vi "Autonomous Independent.vi"() -> ()   [LabVIEW 2020]
doc: "This VI is called when autonomous begins, and will automatically be terminated when autonomous ends. You can carry out timed or sensor driven robot movement independently without needing to return to the caller."
uses:
  <vilib>/Rock Robotics/WPI/ThirdParty/Phoenix-LabVIEW/Motor Controller/Controls/CTRE_Phoenix_MotorControl_ControlMode.ctl
  <vilib>/Rock Robotics/WPI/Solenoid/WPI_SolenoidValue.ctl
  <vilib>/Rock Robotics/WPI/Utilities/WPI_GetSetVariantRefNum.vi
  <vilib>/Rock Robotics/Network Tables/NT Read String.vi
  <vilib>/Rock Robotics/Network Tables/NT Write Numeric Array.vi
  AutonBoolean.vi
  <vilib>/Rock Robotics/Network Tables/NT Read Number.vi
  <vilib>/Rock Robotics/WPI/Solenoid/WPI_SolenoidSetEnum.vi
panel:
  out "Ty 60":dbl
  out "Ty 59":dbl
  out "Orange Limit Pressed 26":bool
  out "Blue Limit Pressed 26":bool
  out "Ty 58":dbl
  out "Orange Limit Pressed 25":bool
  out "Blue Limit Pressed 25":bool
  out "Ty 57":dbl
  out "Intake 13":bool
  out "Elevate 13":bool
  out "Ty 56":dbl
  out "Ty 55":dbl
  out "Orange Limit Pressed 24":bool
  out "Blue Limit Pressed 24":bool
  out "Ty 54":dbl
  out "Orange Limit Pressed 23":bool
  out "Blue Limit Pressed 23":bool
  out "Ty 53":dbl
  out "Intake 12":bool
  out "Elevate 12":bool
  out "Intake 11":bool
  out "Elevate 11":bool
  out "Orange Limit Pressed 22":bool
  out "Blue Limit Pressed 22":bool
  out "Ty 52":dbl
  out "Orange Limit Pressed 21":bool
  out "Blue Limit Pressed 21":bool
  out "Ty 51":dbl
  out "Ty 50":dbl
  out "Ty 49":dbl
  out "Ty 48":dbl
  out "Ty 47":dbl
  out "Ty 46":dbl
  out "Ty 45":dbl
  out "Intake 10":bool
  out "Elevate 10":bool
  out "Orange Limit Pressed 20":bool
  out "Blue Limit Pressed 20":bool
  out "Ty 44":dbl
  out "Orange Limit Pressed 19":bool
  out "Blue Limit Pressed 19":bool
  out "Ty 43":dbl
  out "Ty 42":dbl
  out "Ty 41":dbl
  out "Ty 40":dbl
  out "Ty 39":dbl
  out "Ty 38":dbl
  out "Ty 37":dbl
  out "Intake 9":bool
  out "Elevate 9":bool
  out "Orange Limit Pressed 18":bool
  out "Blue Limit Pressed 18":bool
  out "Ty 36":dbl
  out "Orange Limit Pressed 17":bool
  out "Blue Limit Pressed 17":bool
  out "Ty 35":dbl
  out "Ty 34":dbl
  out "Ty 33":dbl
  out "Intake 8":bool
  out "Elevate 8":bool
  out "Orange Limit Pressed 16":bool
  out "Blue Limit Pressed 16":bool
  out "Ty 28":dbl
  out "Orange Limit Pressed 15":bool
  out "Blue Limit Pressed 15":bool
  out "Ty 27":dbl
  out "Intake 6":bool
  out "Elevate 6":bool
  out "Orange Limit Pressed 12":bool
  out "Blue Limit Pressed 12":bool
  out "Ty 26":dbl
  out "Orange Limit Pressed 11":bool
  out "Blue Limit Pressed 11":bool
  out "Ty 25":dbl
  out "Intake 7":bool
  out "Elevate 7":bool
  out "Orange Limit Pressed 13":bool
  out "Blue Limit Pressed 13":bool
  out "Ty 29":dbl
  out "Orange Limit Pressed 14":bool
  out "Blue Limit Pressed 14":bool
  out "Ty 30":dbl
  out "Ty 31":dbl
  out "Ty 32":dbl
  out "Ty 24":dbl
  out "Ty 23":dbl
  out "Ty 22":dbl
  out "Ty 21":dbl
  out "Ty 20":dbl
  out "Ty 19":dbl
  out "Ty 18":dbl
  out "Ty 17":dbl
  out "Orange Limit Pressed 10":bool
  out "Blue Limit Pressed 10":bool
  out "Ty 16":dbl
  out "Orange Limit Pressed 9":bool
  out "Blue Limit Pressed 9":bool
  out "Ty 15":dbl
  out "Intake 5":bool
  out "Elevate 5":bool
  out "Ty 14":dbl
  out "Ty 13":dbl
  out "Ty 12":dbl
  out "Ty 11":dbl
  out "Ty 10":dbl
  out "Ty 9":dbl
  out "Orange Limit Pressed 4":bool
  out "Blue Limit Pressed 4":bool
  out "Ty 4":dbl
  out "Orange Limit Pressed 3":bool
  out "Blue Limit Pressed 3":bool
  out "Ty 3":dbl
  out "Intake 2":bool
  out "Elevate 2":bool
  out "Intake":bool
  out "Elevate":bool
  out "Orange Limit Pressed":bool
  out "Blue Limit Pressed":bool
  out "Ty":dbl
  out "Orange Limit Pressed 2":bool
  out "Blue Limit Pressed 2":bool
  out "Ty 2":dbl
  out "Intake 3":bool
  out "Elevate 3":bool
  out "Orange Limit Pressed 5":bool
  out "Blue Limit Pressed 5":bool
  out "Ty 5":dbl
  out "Orange Limit Pressed 6":bool
  out "Blue Limit Pressed 6":bool
  out "Ty 6":dbl
  out "Intake 4":bool
  out "Elevate 4":bool
  out "Orange Limit Pressed 7":bool
  out "Blue Limit Pressed 7":bool
  out "Ty 7":dbl
  out "Orange Limit Pressed 8":bool
  out "Blue Limit Pressed 8":bool
  out "Ty 8":dbl
  # "Be sure to right-click and choose Data Operations>>Make Current Value default if you want to save the array values with the VI"
types:
  T1 = typedef "WPI_JoystickDevRef.ctl" = cluster{"Device":T2}
  T2 = typedef "WPI_JoystickDeviceEnum.ctl" = enum16{"USB 0", "USB 1", "USB 2", "USB 3", "USB 4", "USB 5"}
  T3 = typedef "WPI_SolenoidValue.ctl" = enum16{"Off", "On", "Forward", "Reverse"}
  T4 = typedef "WPI_SwitchDevRef.ctl" = cluster{"DevStatus":errorcluster, "DIO Channel":T5, "CntIndex":T6, "Normally Closed":bool}
  T5 = typedef "FPGA_DIOChannel.ctl" = enum8{"DIO 0", "DIO 1", "DIO 2", "DIO 3", "DIO 4", "DIO 5", "DIO 6", "DIO 7", "DIO 8", "DIO 9", "DIO MXP 0", "DIO MXP 1", "DIO MXP 2", "DIO MXP 3", "DIO MXP 4", "DIO MXP 5", "DIO MXP 6", "DIO MXP 7", "DIO MXP 8", "DIO MXP 9", "DIO MXP 10", "DIO MXP 11", "DIO MXP 12", "DIO MXP 13", "DIO MXP 14", "DIO MXP 15", "SPI Port CS1", "SPI Port CS2", "SPI Port CS3", "SPI Port MISO", "SPI Port MOSI", "Invalid"}
  T6 = typedef "FPGA_CounterCtrSystemIndex.ctl" = enum8{"Ctr 0", "Ctr 1", "Ctr 2", "Ctr 3", "Ctr 4", "Ctr 5", "Ctr 6", "Ctr 7", "Invalid"}
  T7 = typedef "WPI_MotorControlDeviceRef.ctl" = cluster{"DeviceStatus":errorcluster, "Type":T8, "PWM":cluster{"PWM Channel":T9, "DeadBand":T10}, "CAN":cluster{"Device Number":u8, "SetOutput VI Ref":variant, "GetOutput VI Ref":variant, "Enable VI Ref":variant, "Disable VI Ref":variant, "Data":variant}, "Invert":bool, "DIO PWM":cluster{"PWM \"Enable\" Channel":T9, "DIOChannel":T5, "PWM Rate":dbl}}
  T8 = typedef "WPI_MotorControlType.ctl" = enum16{"PWM", "CAN", "DIO PWM"}
  T9 = typedef "FPGA_DIOPWMChannel.ctl" = enum8{"PWM 0", "PWM 1", "PWM 2", "PWM 3", "PWM 4", "PWM 5", "PWM 6", "PWM 7", "PWM 8", "PWM 9", "PWM MXP 0", "PWM MXP 1", "PWM MXP 2", "PWM MXP 3", "PWM MXP 4", "PWM MXP 5", "PWM MXP 6", "PWM MXP 7", "PWM MXP 8", "PWM MXP 9", "Invalid"}
  T10 = typedef "WPI_PWMDeadband.ctl" = cluster{"Name":string, "maxPositivePwm":i32, "minPositivePwm":i32, "centerPwm":i32, "maxNegativePwm":i32, "minNegativePwm":i32, "angularRange":u16}
  T11 = typedef "CTRE_Phoenix_MotorControl_ControlMode.ctl" = u16
  T12 = typedef "WPI_SolenoidDevRef.ctl" = cluster{"DevStatus":errorcluster, "Pneumatics Control Module":u8, "Forward Solenoid Channel":T13, "Reverse Solenoid Channel":T13}
  T13 = typedef "WPI_SolenoidChannel.ctl" = enum8{"Solenoid 0", "Solenoid 1", "Solenoid 2", "Solenoid 3", "Solenoid 4", "Solenoid 5", "Solenoid 6", "Solenoid 7", "Solenoid 8", "Solenoid 9", "Solenoid 10", "Solenoid 11", "Solenoid 12", "Solenoid 13", "Solenoid 14", "Solenoid 15", "Invalid"}
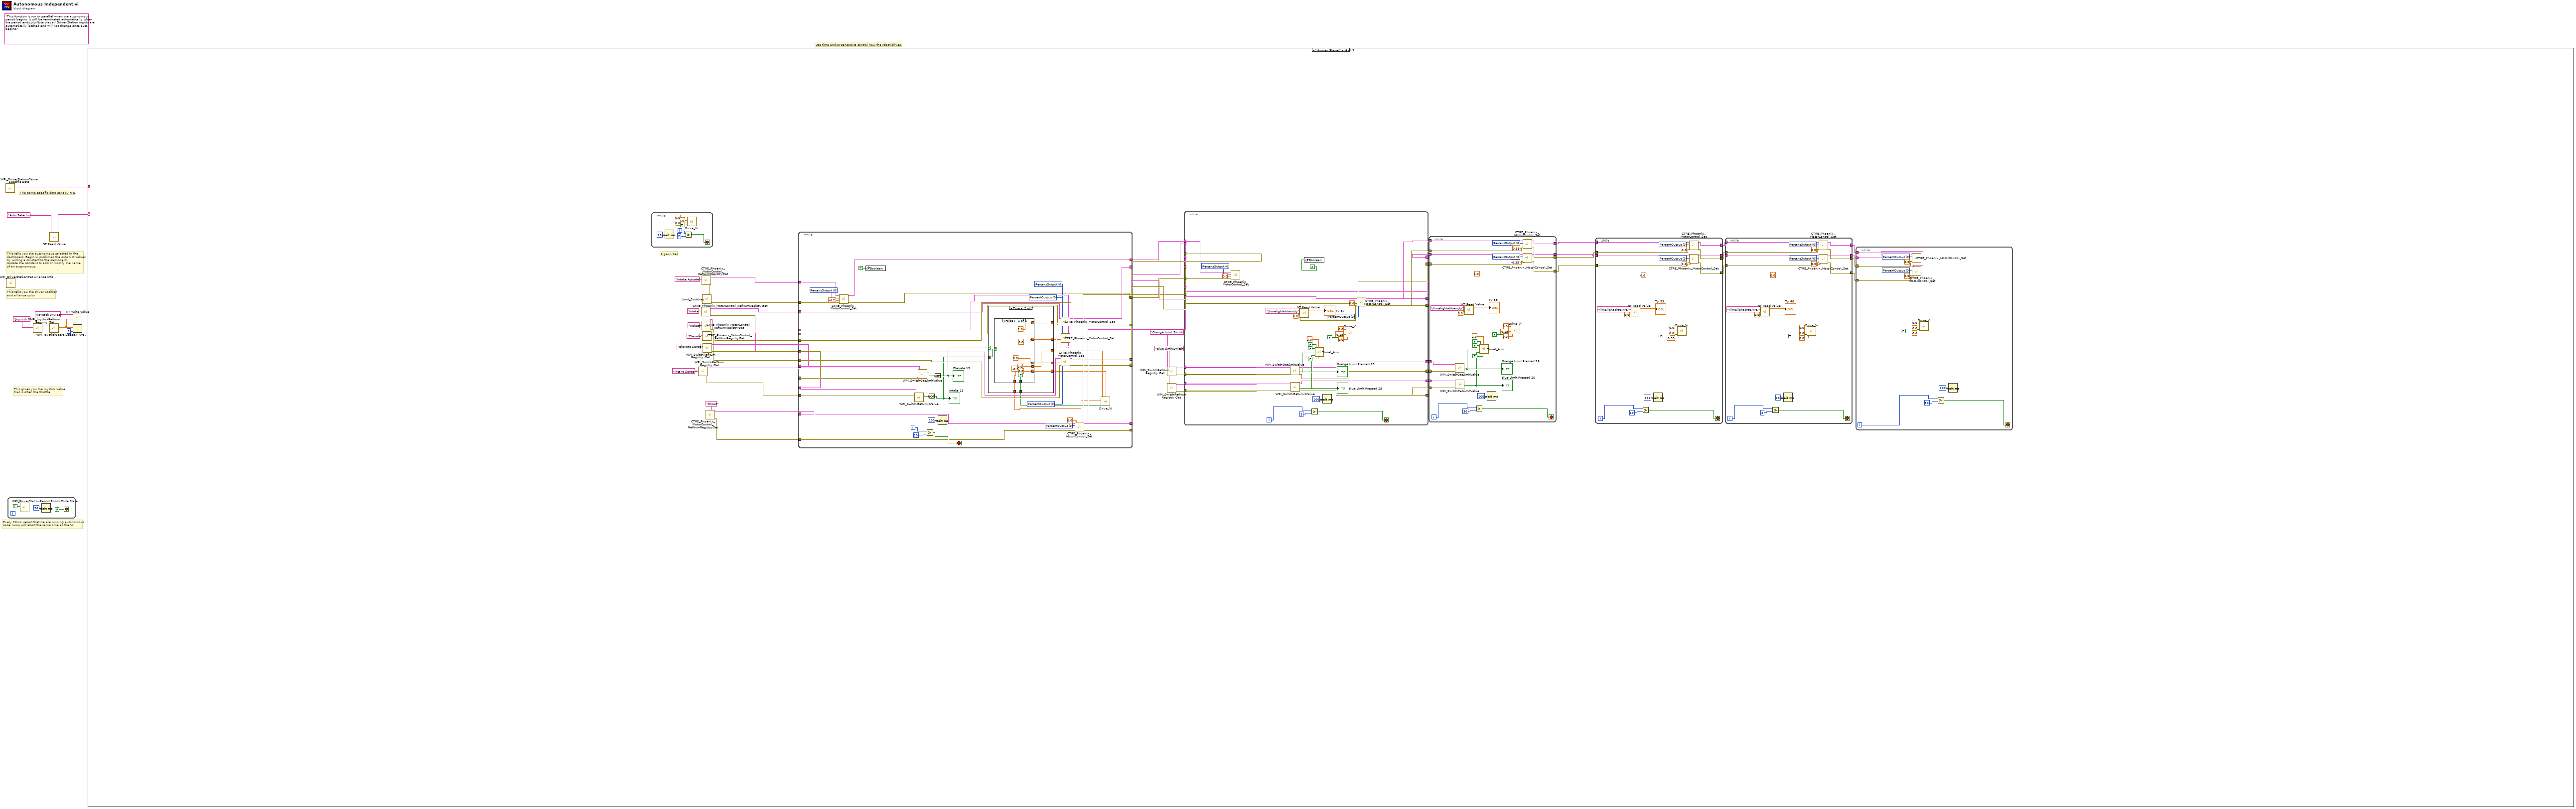
[diagram p0: block diagram]
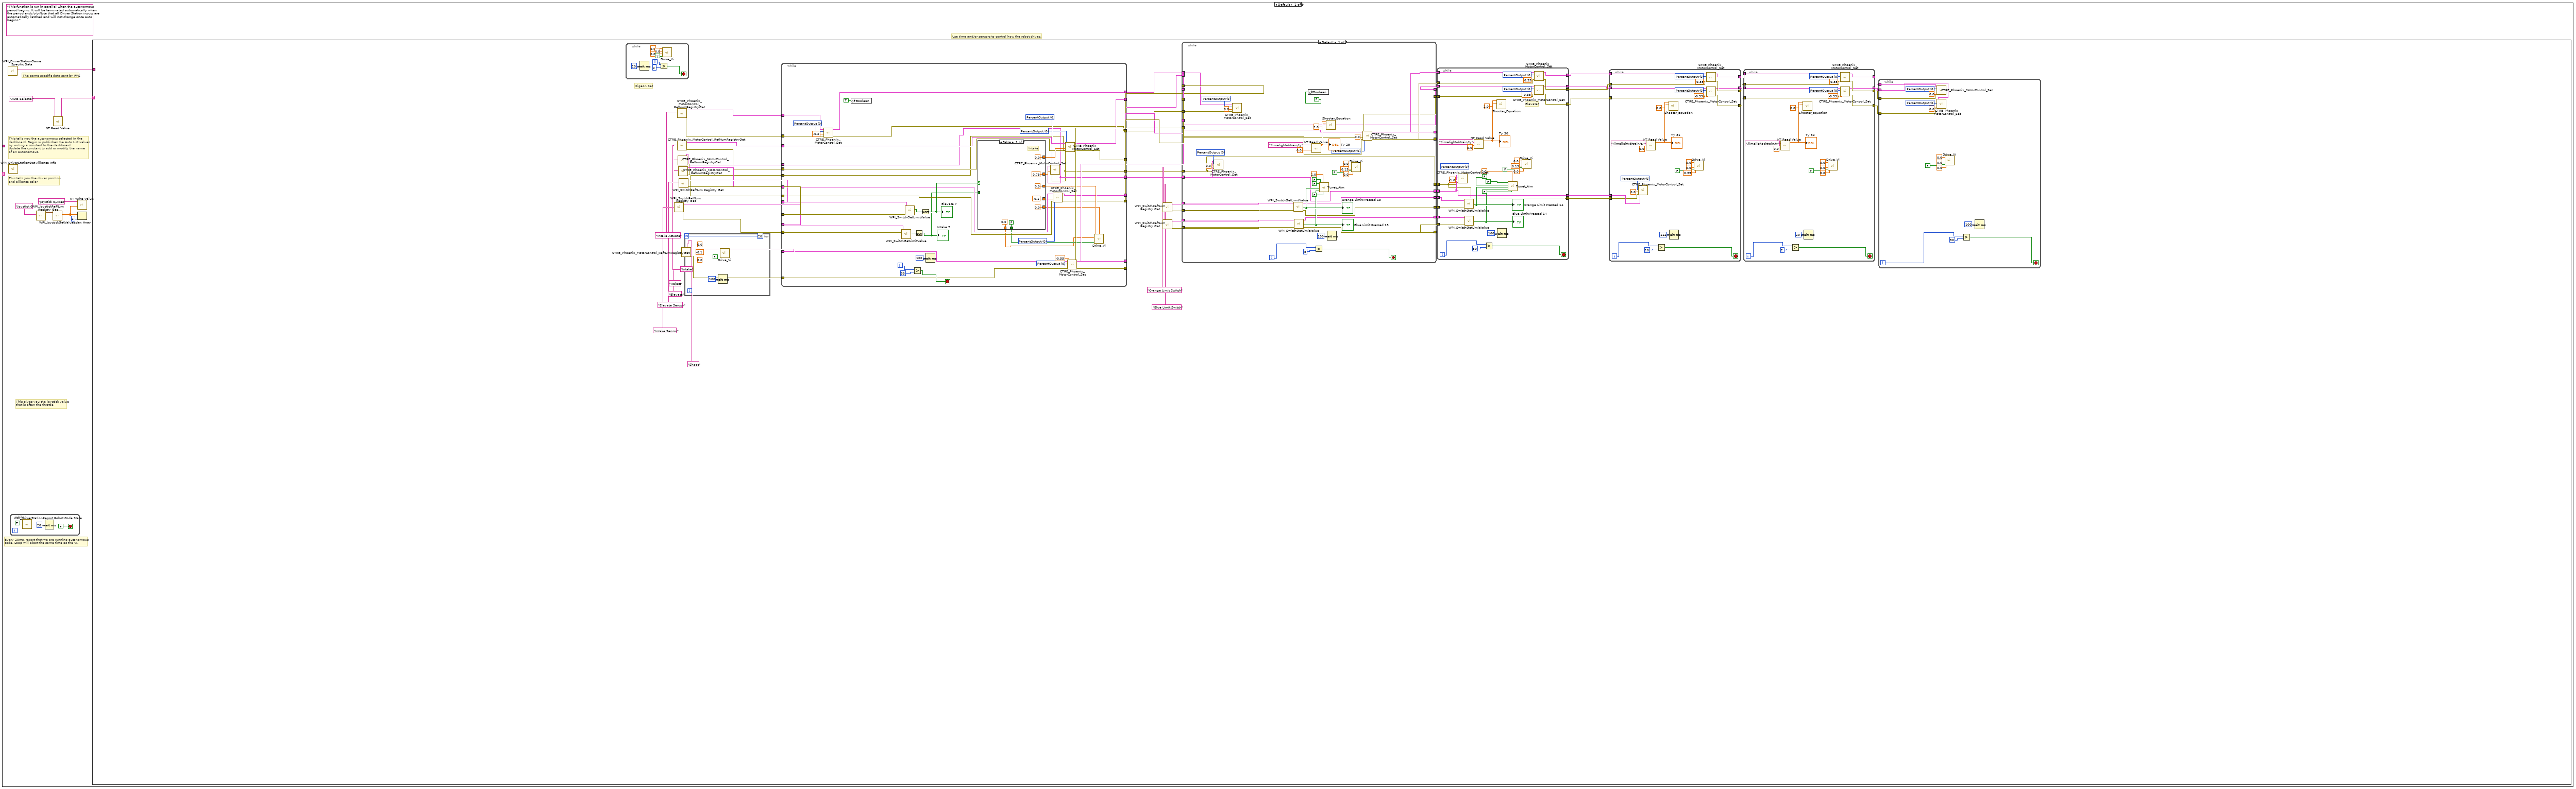
[diagram p2: hidden frame]
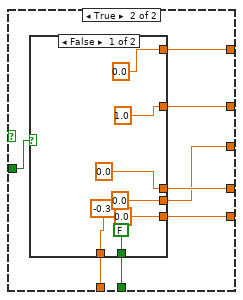
[diagram p3: hidden frame]
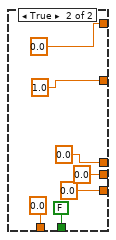
[diagram p4: hidden frame]
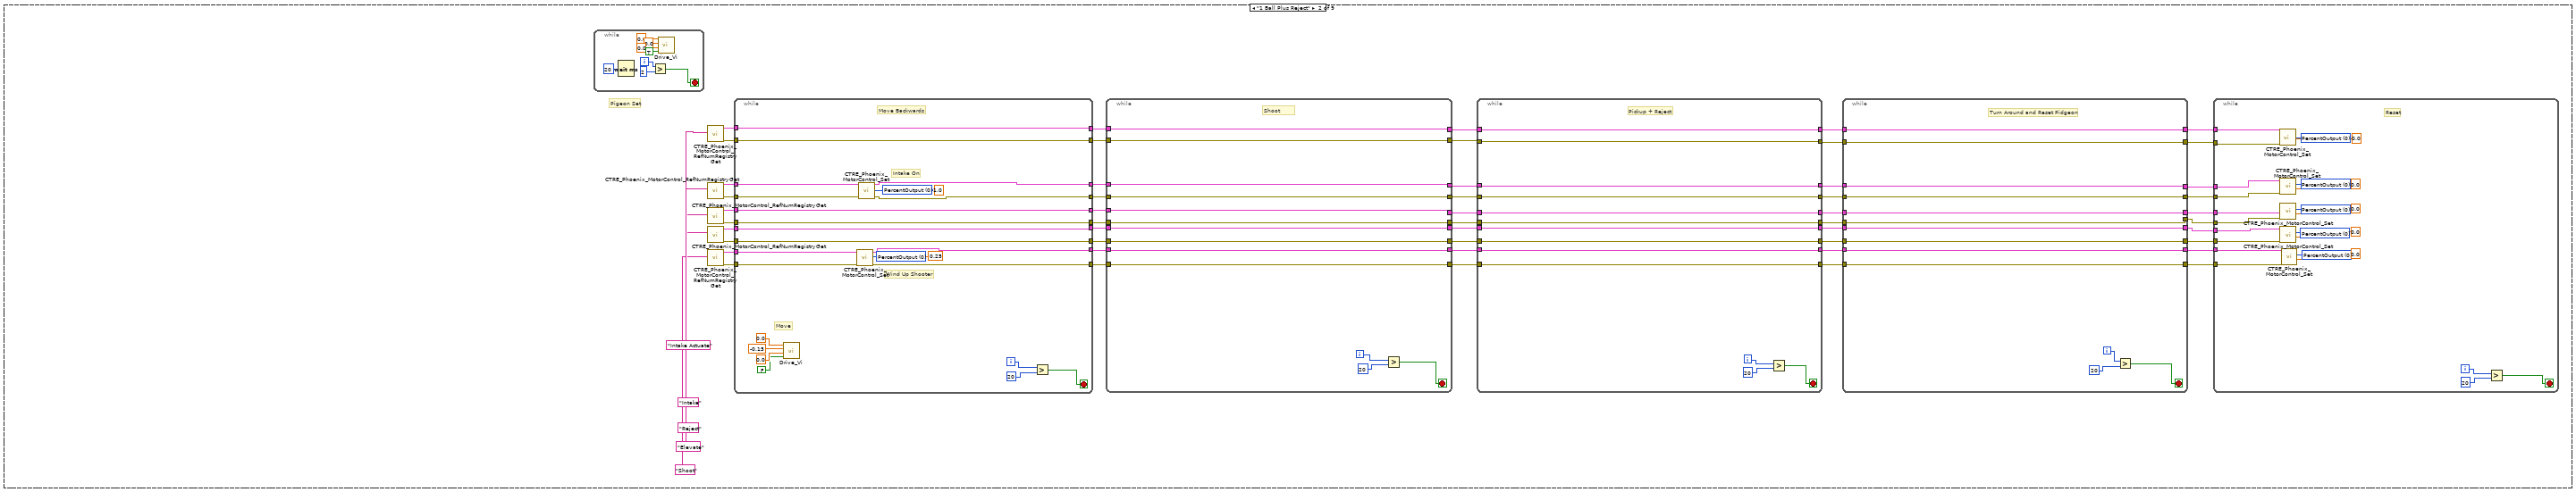
[diagram p5: hidden frame]
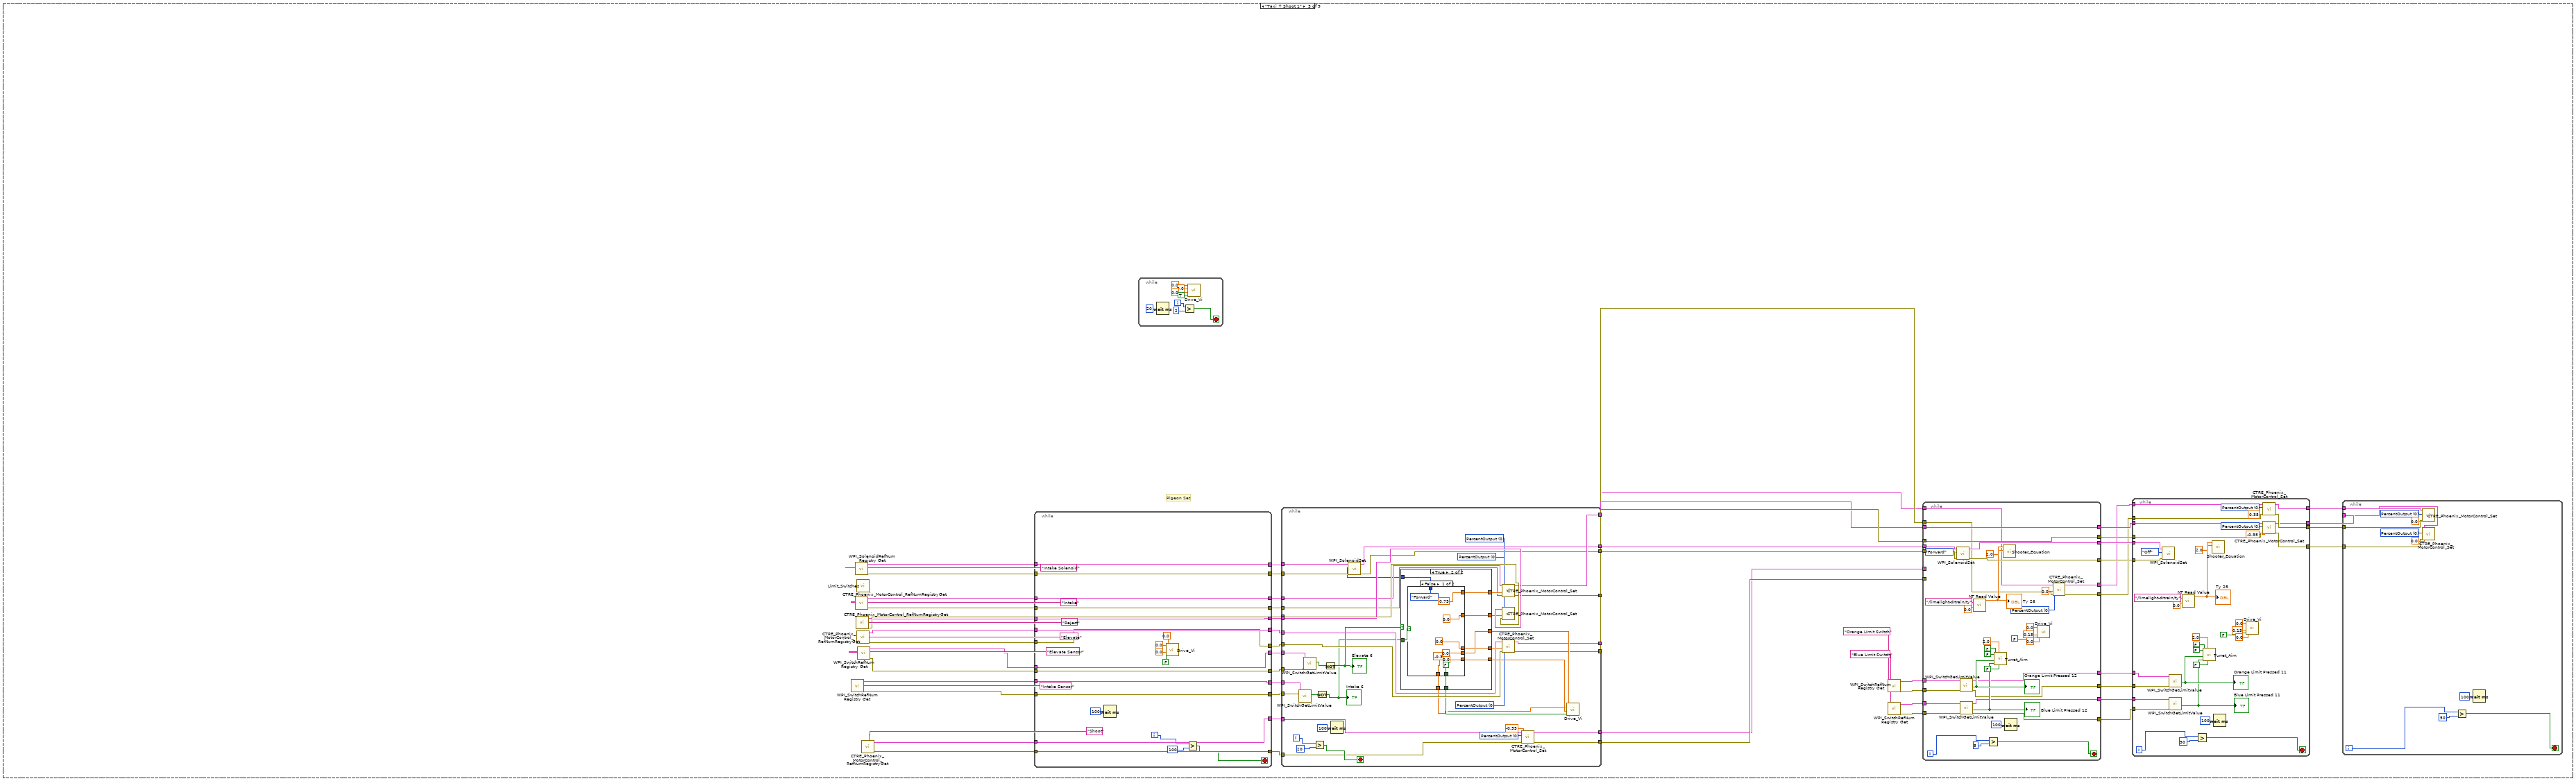
[diagram p6: hidden frame]
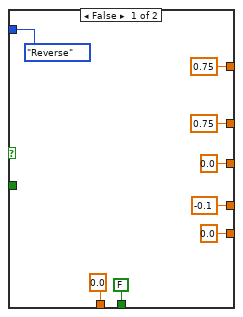
[diagram p7: hidden frame]
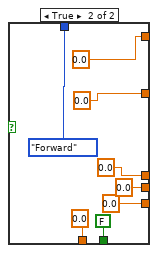
[diagram p8: hidden frame]
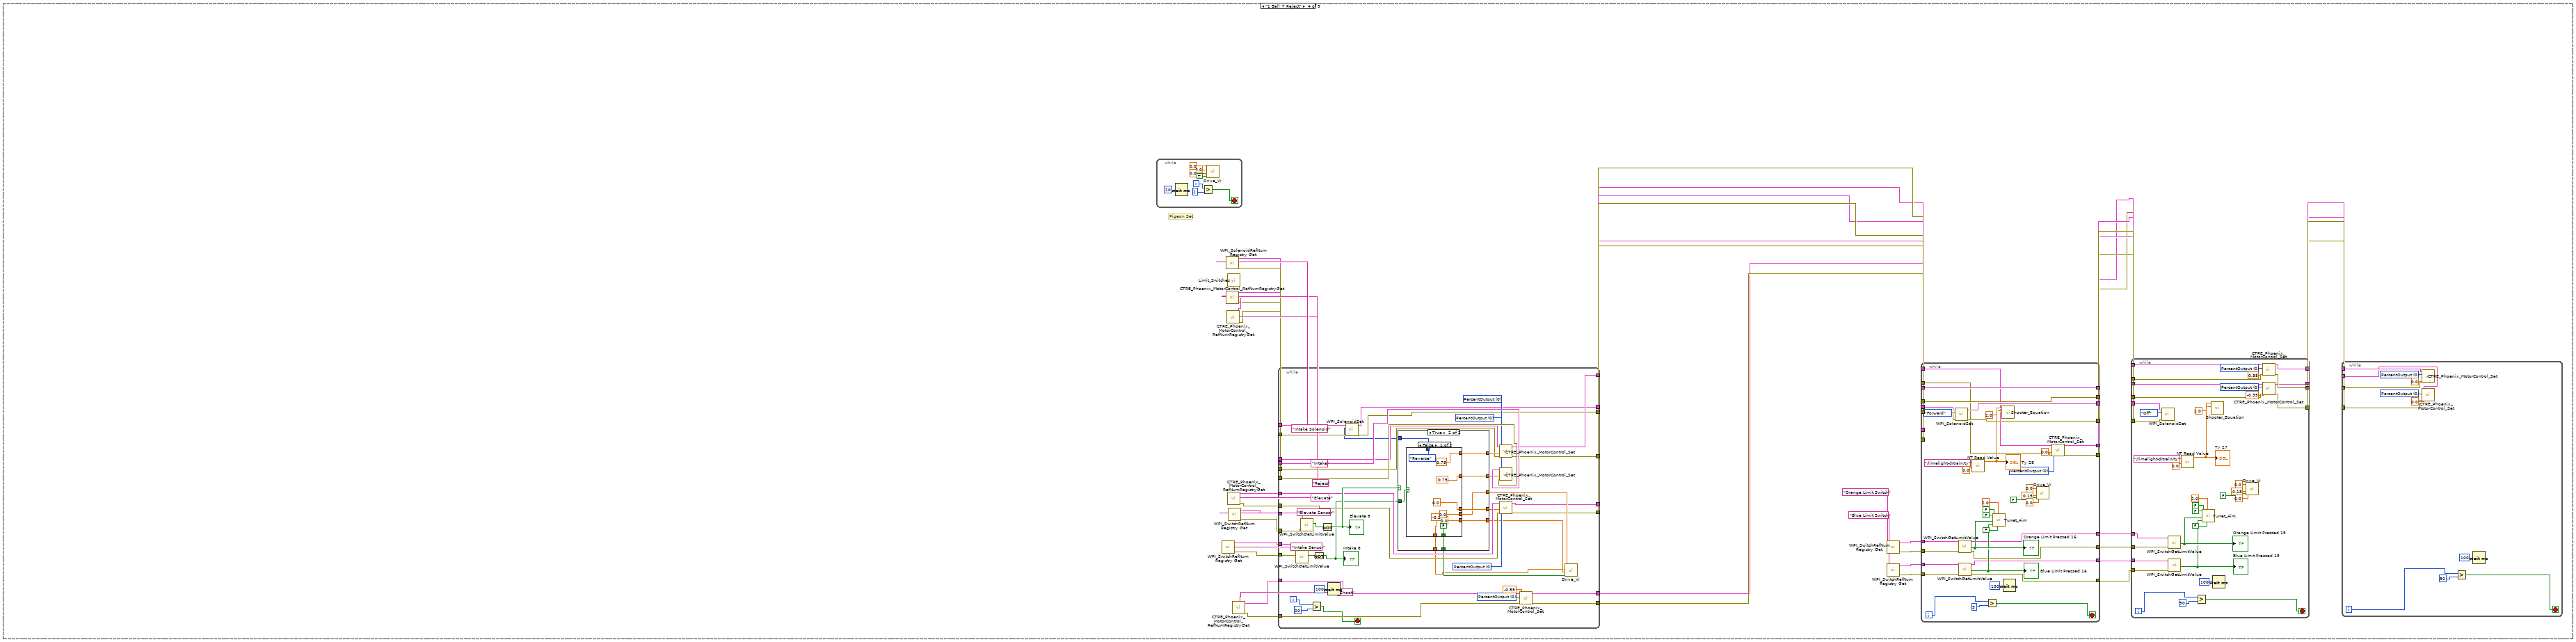
[diagram p9: hidden frame]
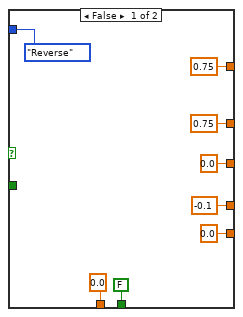
[diagram p10: hidden frame]
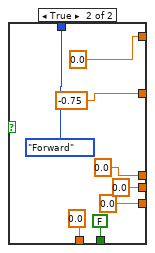
[diagram p11: hidden frame]
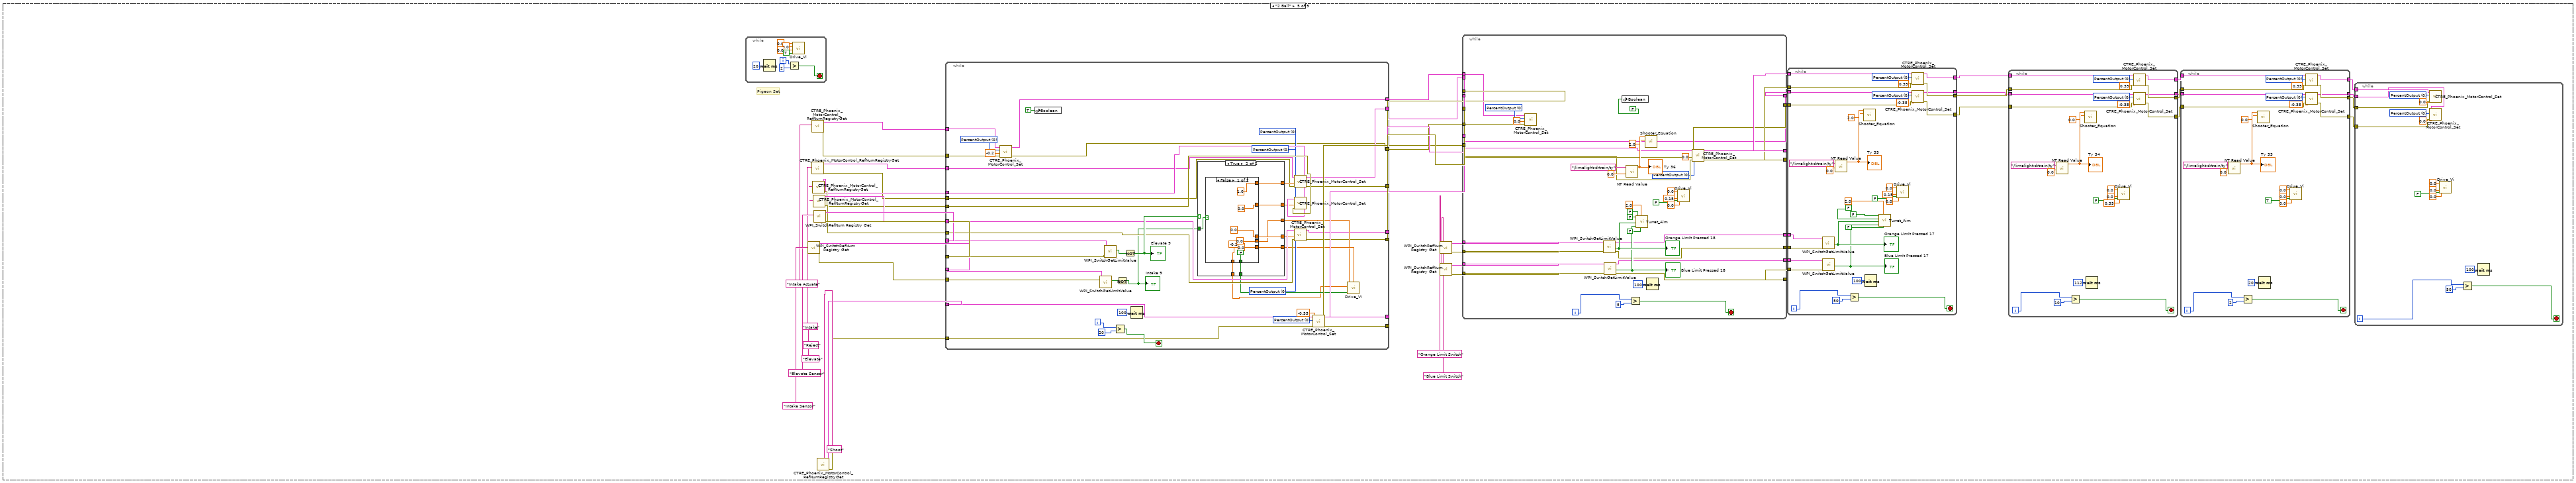
[diagram p12: hidden frame]
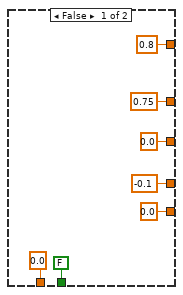
[diagram p13: hidden frame]
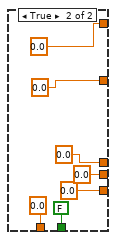
[diagram p14: hidden frame]
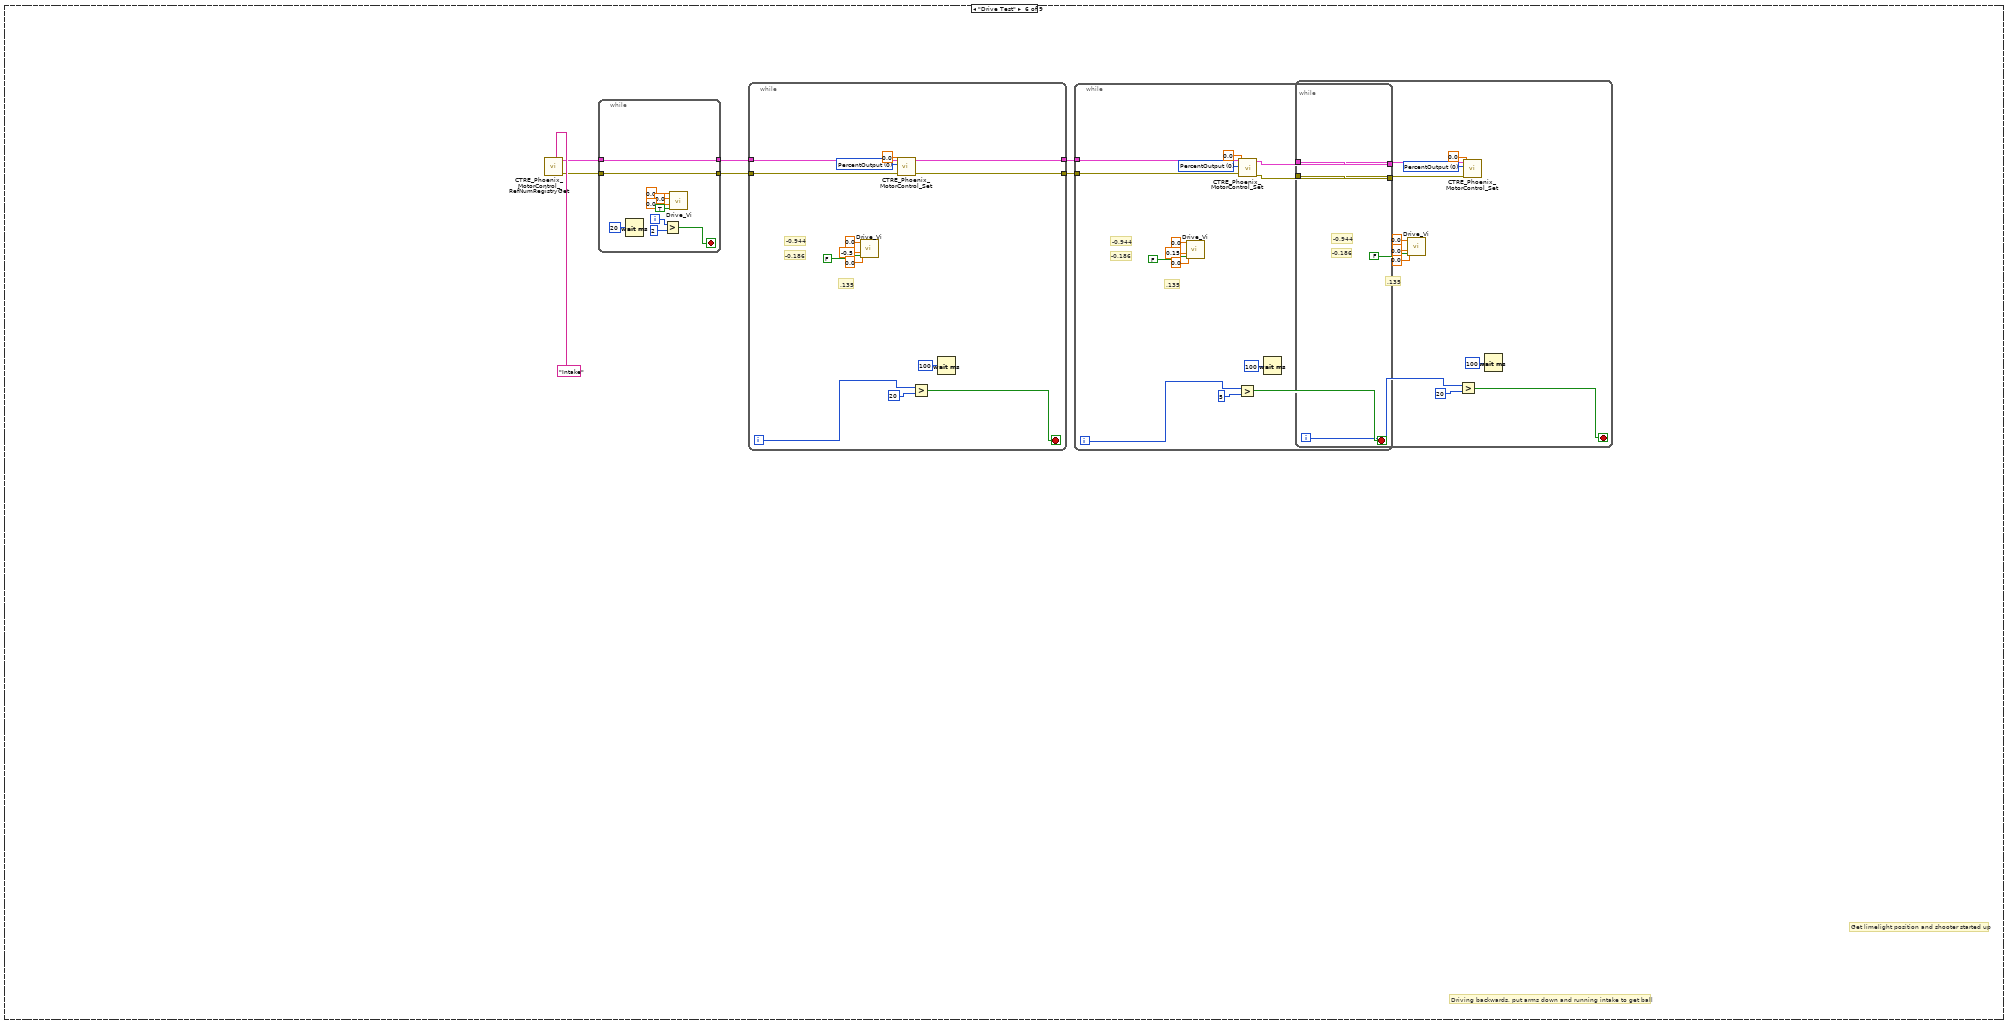
[diagram p15: hidden frame]
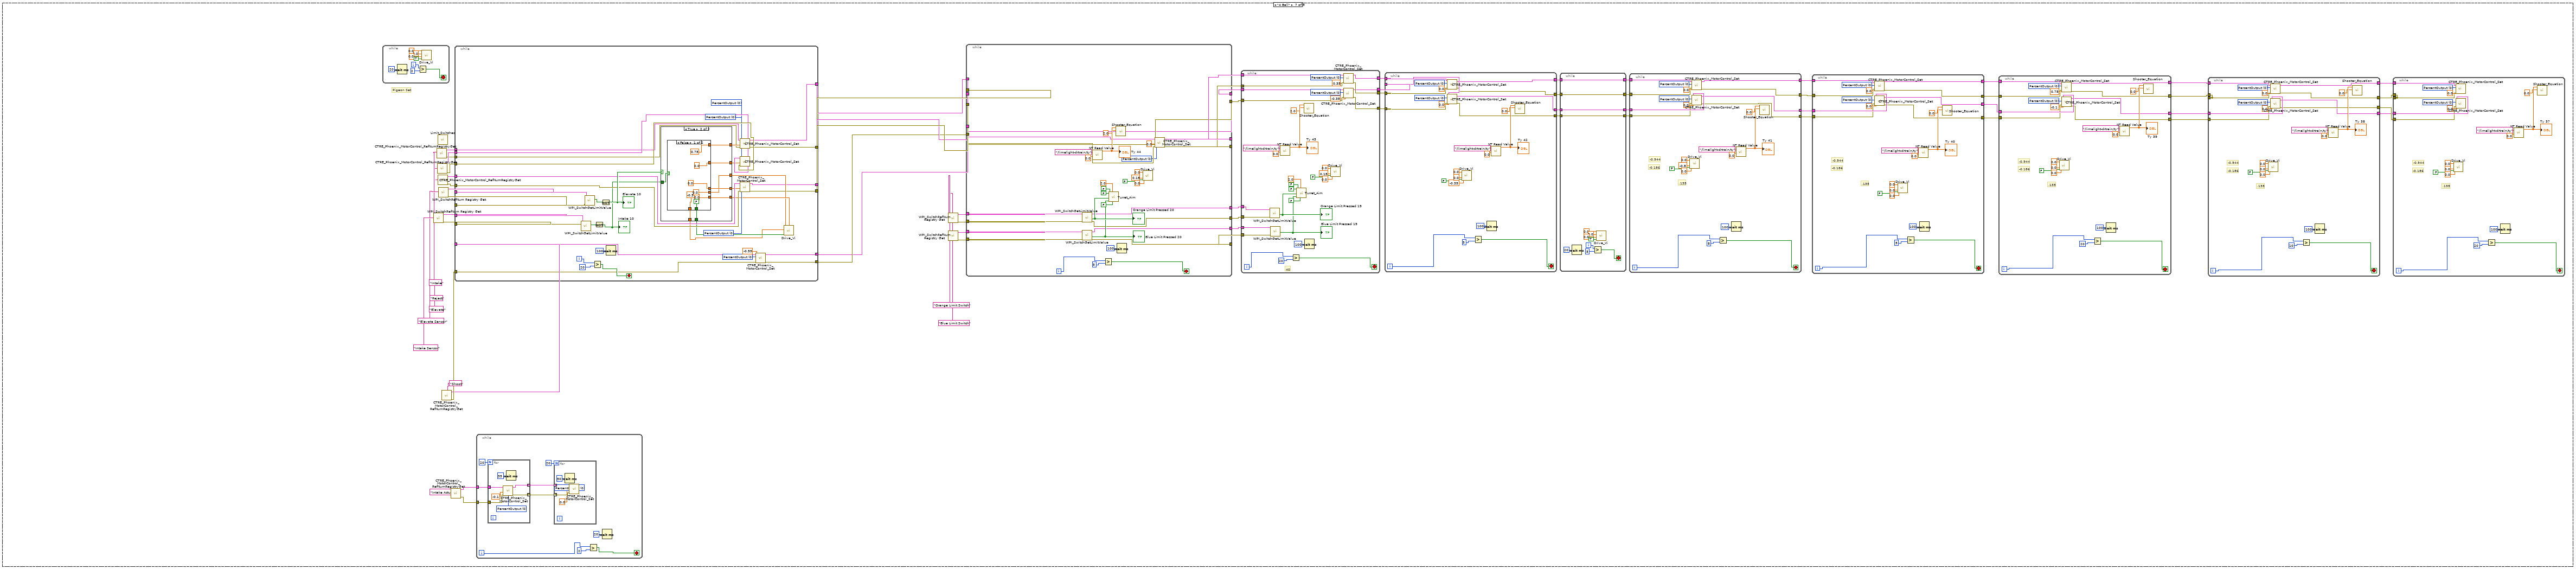
[diagram p16: hidden frame]
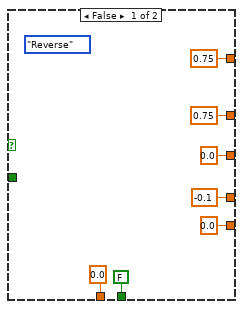
[diagram p17: hidden frame]
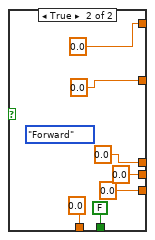
[diagram p18: hidden frame]
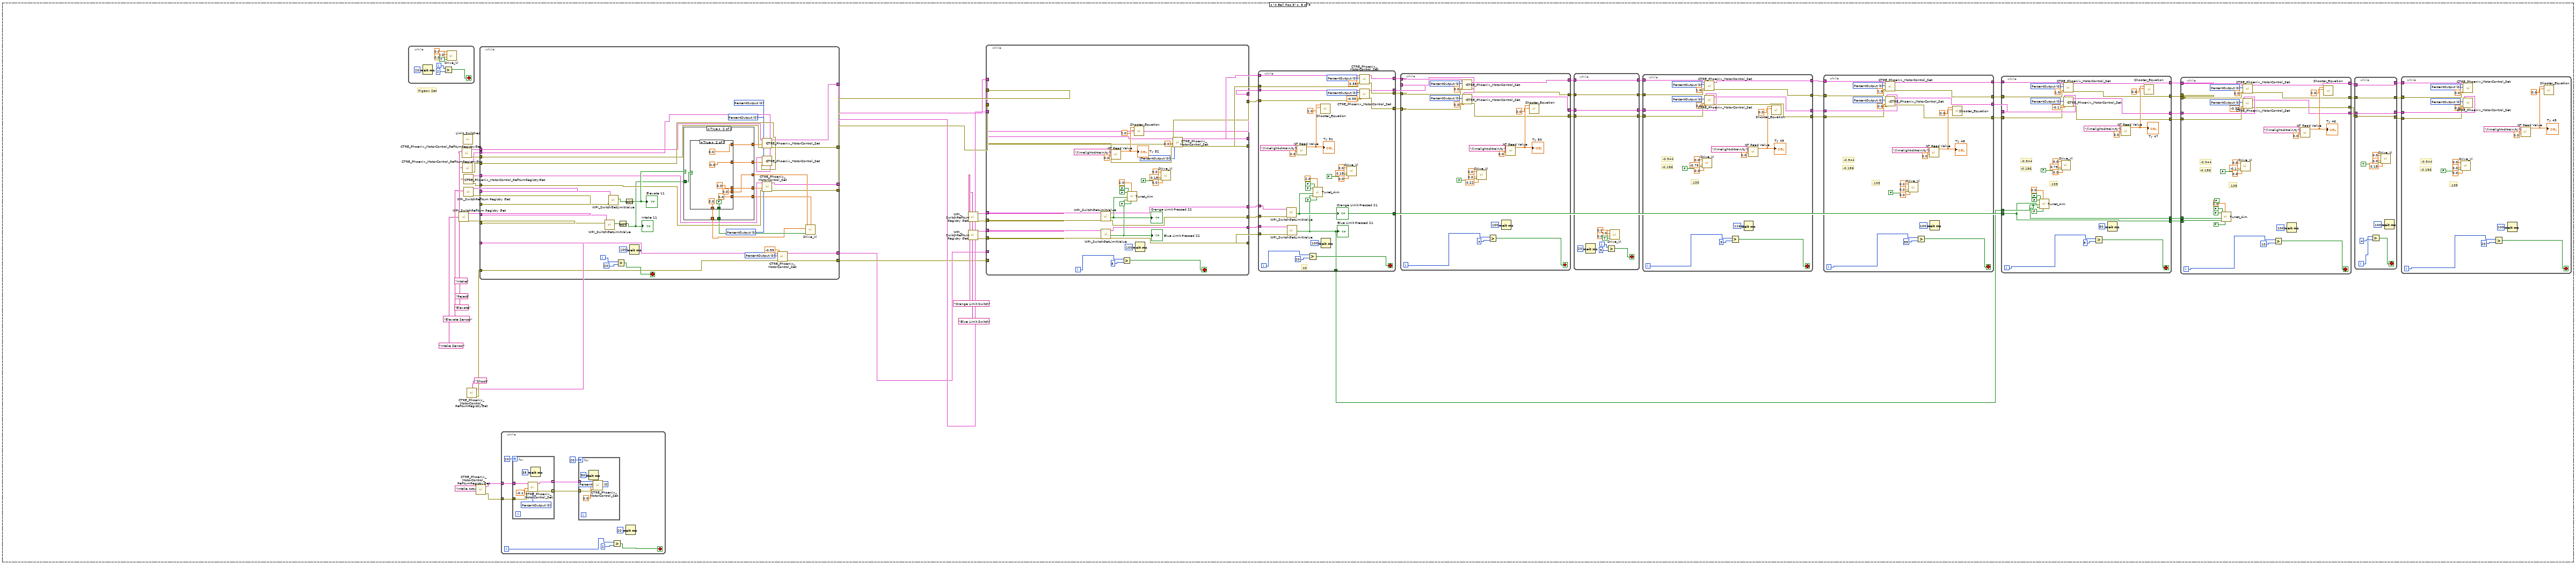
[diagram p19: hidden frame]
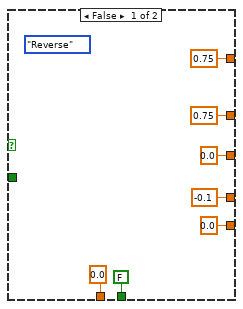
[diagram p20: hidden frame]
diagram:
  (unwired) "This function is run in parallel when the autonomous period begins. It will be terminated automatically when the period ends.\n\nNote that all Driver Station inputs are automatically latched and will not change once auto begins."
  # "The game specific data sent by FMS"
  # "This tells you the autonomous selected in the \ndashboard. Begin.vi publishes the Auto List values\nby writing a constant to the dashboard.\nUpdate the constant to add or modify the name\nof an autonomous."
  # "Every 20ms, report that we are running autonomous\ncode. Loop will abort the same time as the VI."
  # "This gives you the joystick value\nthat is often the throttle"
  # "Use time and/or sensors to control how the robot drives."
  # "This tells you the driver position\nand alliance color"
  n1 = call <vilib>:"WPI_DriverStationGame Specific Data.vi"() -> ("Game Specific Data"=w1:string)  [unwired: 11 in]
  n2 = call <vilib>:"WPI_DriverStationGet Alliance Info.vi"() -> ()  [unwired: 12 out]
  n3 = while {
    stop <- FALSE stop-if-true
    n4 = call <vilib>:"WPI_DriverStationReport Robot Code State.vi"("Autonomous"=TRUE) -> ()  [unwired: 10 in, 1 out]
    n5 = Wait (ms)(milliseconds to wait=u32 20) -> ()  [unwired: 1 out]
  }
  n6 = call <vilib>:"WPI_JoystickRefNum Registry Get.vi"("refnum name"="Joystick 0") -> ("JoystickDevRef"=w7:T1)  [unwired: 1 in, 9 out]
  n7 = call <vilib>:"WPI_JoystickGetValues.vi"("JoystickDevRef"=w7) -> ("Axes"=w3:dbl[])  [unwired: 6 in, 4 out]
  n8 = call-poly <vilib>:"NT Read Value.vi"("Name"="Auto Selector") -> ("String"=w4:string)  [unwired: 9 in, 1 out]
  n9 = call-poly <vilib>:"NT Write Value.vi"("Numeric Array"=w3, "Name"="Joystick 0/Axes") -> ()  [unwired: 9 in, 1 out]
  n10 = Index Array(array=w3, index=2) -> ()  [unwired: 1 out]
  n11 = case shown="\"Human Player\"" w4 {
    tunnel: w1 -> [_ _ _ _ _ _ _ _ _]
    frame Default {
      (unwired) "This function is run in parallel when the autonomous period begins. It will be terminated automatically when the period ends.\n\nNote that all Driver Station inputs are automatically latched and will not change once auto begins."
      # "The game specific data sent by FMS"
      # "This tells you the autonomous selected in the \ndashboard. Begin.vi publishes the Auto List values\nby writing a constant to the dashboard.\nUpdate the constant to add or modify the name\nof an autonomous."
      # "Every 20ms, report that we are running autonomous\ncode. Loop will abort the same time as the VI."
      # "This gives you the joystick value\nthat is often the throttle"
      # "Use time and/or sensors to control how the robot drives."
      # "This tells you the driver position\nand alliance color"
      n12 = call <vilib>:"WPI_DriverStationGame Specific Data.vi"() -> ("Game Specific Data"=w12:string)  [unwired: 11 in]
      n13 = call <vilib>:"WPI_DriverStationGet Alliance Info.vi"() -> ()  [unwired: 12 out]
      n14 = while {
        stop <- FALSE stop-if-true
        n15 = call <vilib>:"WPI_DriverStationReport Robot Code State.vi"("Autonomous"=TRUE) -> ()  [unwired: 10 in, 1 out]
        n16 = Wait (ms)(milliseconds to wait=u32 20) -> ()  [unwired: 1 out]
      }
      n17 = call <vilib>:"WPI_JoystickRefNum Registry Get.vi"("refnum name"="Joystick 0") -> ("JoystickDevRef"=w18:T1)  [unwired: 1 in, 9 out]
      n18 = call <vilib>:"WPI_JoystickGetValues.vi"("JoystickDevRef"=w18) -> ("Axes"=w14:dbl[])  [unwired: 6 in, 4 out]
      n19 = call-poly <vilib>:"NT Read Value.vi"("Name"="Auto Selector") -> ("String"=w15:string)  [unwired: 9 in, 1 out]
      n20 = call-poly <vilib>:"NT Write Value.vi"("Numeric Array"=w14, "Name"="Joystick 0/Axes") -> ()  [unwired: 9 in, 1 out]
      n21 = Index Array(array=w14, index=2) -> ()  [unwired: 1 out]
      n22 = case shown="Default" w15 {
        tunnel: w12 -> [_ _ _ _ _ _ _ _ _]
        frame Default {
          # "Pigeon Set"
          n23 = while {
            i -> [w310]
            stop <- w311 stop-if-true
            n24 = Wait (ms)(milliseconds to wait=u32 20) -> ()  [unwired: 1 out]
            n25 = Greater?(x=w310, y=2) -> (0:w311:bool)
            n26 = call "Drive_Vi.vi"("Middle Thumb"=TRUE, "Z"=0.0, "Y"=0.0, "X"=0.0) -> ()  [unwired: 8 in]
          }
          n27 = call <vilib>:"WPI_SwitchRefNum Registry Get.vi"("refnum name"="Intake Sensor") -> ("error out"=w73:errorcluster, "SwitchDevRef"=w72:T4)  [unwired: 9 in]
          n28 = call <vilib>:"CTRE_Phoenix_MotorControl_RefNumRegistryGet.vi"("refnum name"="Intake") -> ("error out"=w67:errorcluster, "PhoenixMotorControlDevRef"=w66:T7)  [unwired: 9 in]
          n29 = call <vilib>:"CTRE_Phoenix_MotorControl_RefNumRegistryGet.vi"("refnum name"="Intake Actuate") -> ("error out"=w42:errorcluster, "PhoenixMotorControlDevRef"=w41:T7)  [unwired: 9 in]
          n30 = call <vilib>:"CTRE_Phoenix_MotorControl_RefNumRegistryGet.vi"("refnum name"="Reject") -> ("error out"=w69:errorcluster, "PhoenixMotorControlDevRef"=w68:T7)  [unwired: 9 in]
          n31 = call <vilib>:"CTRE_Phoenix_MotorControl_RefNumRegistryGet.vi"("refnum name"="Elevate") -> ("error out"=w71:errorcluster, "PhoenixMotorControlDevRef"=w70:T7)  [unwired: 9 in]
          n32 = call <vilib>:"WPI_SwitchRefNum Registry Get.vi"("refnum name"="Elevate Sensor") -> ("error out"=w75:errorcluster, "SwitchDevRef"=w74:T4)  [unwired: 9 in]
          n33 = call <vilib>:"CTRE_Phoenix_MotorControl_RefNumRegistryGet.vi"("refnum name"="Shoot") -> ("error out"=w55:errorcluster, "PhoenixMotorControlDevRef"=w54:T7)  [unwired: 9 in]
          n34 = while {
            tunnel: w75 -> [w269]
            tunnel: w74 -> [w268]
            tunnel: w73 -> [w267]
            tunnel: w72 -> [w266]
            tunnel: w71 -> [w263]
            tunnel: w70 -> [w262]
            tunnel: w69 -> [w231]
            tunnel: w68 -> [w232]
            tunnel: w67 -> [w261]
            tunnel: w66 -> [w260]
            tunnel: [w249] -> w59
            tunnel: [w248] -> w58
            tunnel: [w247] -> w57
            tunnel: [w246] -> w56
            tunnel: w55 -> [w245]
            tunnel: w54 -> [w244]
            tunnel: [w241] -> w53
            tunnel: [w240] -> w52
            tunnel: w42 -> [w239]
            tunnel: w41 -> [w238]
            tunnel: [w235] -> w40
            tunnel: [w234] -> w39
            tunnel: [w232] -> w26
            tunnel: [w231] -> w25
            i -> [w272]
            stop <- w273 stop-if-true
            w237 = T11 0 items=["PercentOutput"=0, "Position"=1, "Velocity"=2, "Current"=3, "Follower"=5, "MotionProfile"=6, "MotionMagic"=7, "MotionProfileArc"=10, "Disabled"=15] ("Control Mode")
            w243 = T11 0 items=["PercentOutput"=0, "Position"=1, "Velocity"=2, "Current"=3, "Follower"=5, "MotionProfile"=6, "MotionMagic"=7, "MotionProfileArc"=10, "Disabled"=15] ("Control Mode")
            w254 = T11 0 items=["PercentOutput"=0, "Position"=1, "Velocity"=2, "Current"=3, "Follower"=5, "MotionProfile"=6, "MotionMagic"=7, "MotionProfileArc"=10, "Disabled"=15] ("Control Mode")
            w255 = T11 0 items=["PercentOutput"=0, "Position"=1, "Velocity"=2, "Current"=3, "Follower"=5, "MotionProfile"=6, "MotionMagic"=7, "MotionProfileArc"=10, "Disabled"=15] ("Control Mode")
            w256 = T11 0 items=["PercentOutput"=0, "Position"=1, "Velocity"=2, "Current"=3, "Follower"=5, "MotionProfile"=6, "MotionMagic"=7, "MotionProfileArc"=10, "Disabled"=15] ("Control Mode")
            n35 = call <vilib>:"CTRE_Phoenix_MotorControl_Set.vi"("error in (no error)"=w239, "Output"=-0.2, "Control Mode"=w237, "PhoenixMotorControlDevRef"=w238) -> ("error out"=w234:errorcluster, "PhoenixMotorControlDevRef"=w235:T7)  [unwired: 6 in]
            n36 = global write "AutonBoolean.vi" "Boolean"(TRUE ("Boolean")) -> ()
            n37 = call <vilib>:"WPI_SwitchGetLimitValue.vi"("error in (no error)"=w267, "SwitchDevRef"=w266) -> ("Switch Pressed"=w270:bool)  [unwired: 7 in, 2 out]
            n38 = call <vilib>:"WPI_SwitchGetLimitValue.vi"("error in (no error)"=w269, "SwitchDevRef"=w268) -> ("Switch Pressed"=w271:bool)  [unwired: 7 in, 2 out]
            n39 = Greater?(x=w272, y=35) -> (0:w273:bool)
            n40 = Not(x=w270) -> (.not. x?=w259:bool)
            "Intake 7" <- w259
            n41 = Not(x=w271) -> (.not. x?=w265:bool)
            "Elevate 7" <- w265
            n42 = Wait (ms)(milliseconds to wait=u32 100) -> ()  [unwired: 1 out]
            n43 = case shown="False" w265 {
              tunnel: [0.0 ("Output") w290] -> w264
              tunnel: w259 -> [_ w287]
              tunnel: [0.75 ("Output") w289] -> w258
              tunnel: [-0.1 ("Output") w288] -> w257
              tunnel: [FALSE ("Middle Thumb") w286] -> w253
              tunnel: [0.0 ("Z") w285] -> w252
              tunnel: [0.0 ("Y") w284] -> w251
              tunnel: [0.0 ("X") w283] -> w250
              frame False {
                # "Intake"
              }
              frame True {
                n44 = case shown="False" w287 {
                  tunnel: [0.0 ("Output") 0.0 ("Output")] -> w290
                  tunnel: [1.0 ("Output") 1.0 ("Output")] -> w289
                  tunnel: [0.0 ("Output") 0.0 ("Output")] -> w288
                  tunnel: [FALSE ("Middle Thumb") FALSE ("Middle Thumb")] -> w286
                  tunnel: [0.0 ("Z") 0.0 ("Z")] -> w285
                  tunnel: [-0.3 ("Y") 0.0 ("Y")] -> w284
                  tunnel: [0.0 ("X") 0.0 ("X")] -> w283
                  frame False {
                  }
                  frame True {
                  }
                }
              }
            }
            n45 = call <vilib>:"CTRE_Phoenix_MotorControl_Set.vi"("error in (no error)"=w231, "Output"=w258, "Control Mode"=w255, "PhoenixMotorControlDevRef"=w232) -> ()  [unwired: 6 in, 2 out]
            n46 = call <vilib>:"CTRE_Phoenix_MotorControl_Set.vi"("error in (no error)"=w263, "Output"=w257, "Control Mode"=w256, "PhoenixMotorControlDevRef"=w262) -> ("error out"=w249:errorcluster, "PhoenixMotorControlDevRef"=w248:T7)  [unwired: 6 in]
            n47 = call <vilib>:"CTRE_Phoenix_MotorControl_Set.vi"("error in (no error)"=w261, "Output"=w264, "Control Mode"=w254, "PhoenixMotorControlDevRef"=w260) -> ("error out"=w247:errorcluster, "PhoenixMotorControlDevRef"=w246:T7)  [unwired: 6 in]
            n48 = call <vilib>:"CTRE_Phoenix_MotorControl_Set.vi"("error in (no error)"=w245, "Output"=-0.55, "Control Mode"=w243, "PhoenixMotorControlDevRef"=w244) -> ("error out"=w241:errorcluster, "PhoenixMotorControlDevRef"=w240:T7)  [unwired: 6 in]
            n49 = call "Drive_Vi.vi"("Middle Thumb"=w253, "Z"=w252, "Y"=w251, "X"=w250) -> ()  [unwired: 8 in]
          }
          n50 = call <vilib>:"WPI_SwitchRefNum Registry Get.vi"("refnum name"="Orange Limit Switch") -> ("error out"=w61:errorcluster, "SwitchDevRef"=w60:T4)  [unwired: 9 in]
          n51 = call <vilib>:"WPI_SwitchRefNum Registry Get.vi"("refnum name"="Blue Limit Switch") -> ("error out"=w63:errorcluster, "SwitchDevRef"=w62:T4)  [unwired: 9 in]
          n52 = while {
            tunnel: w53 -> [_]
            tunnel: w52 -> [_]
            tunnel: w63 -> [w228]
            tunnel: w62 -> [w227]
            tunnel: w61 -> [w226]
            tunnel: w60 -> [w225]
            tunnel: w59 -> [w204]
            tunnel: w58 -> [w203]
            tunnel: w57 -> [w199]
            tunnel: w56 -> [w200]
            tunnel: [w208] -> w51
            tunnel: [w207] -> w50
            tunnel: [w206] -> w49
            tunnel: [w205] -> w48
            tunnel: [w204] -> w47
            tunnel: [w203] -> w46
            tunnel: [w202] -> w45
            tunnel: [w201] -> w44
            tunnel: w40 -> [w194]
            tunnel: w39 -> [w193]
            tunnel: w26 -> [w189]
            tunnel: w25 -> [w188]
            tunnel: [w189] -> w24
            tunnel: [w188] -> w23
            i -> [w214]
            stop <- w213 stop-if-true
            w191 = T11 0 items=["PercentOutput"=0, "Position"=1, "Velocity"=2, "Current"=3, "Follower"=5, "MotionProfile"=6, "MotionMagic"=7, "MotionProfileArc"=10, "Disabled"=15] ("Control Mode")
            w196 = T11 0 items=["PercentOutput"=0, "Position"=1, "Velocity"=2, "Current"=3, "Follower"=5, "MotionProfile"=6, "MotionMagic"=7, "MotionProfileArc"=10, "Disabled"=15] ("Control Mode")
            w198 = T11 0 items=["PercentOutput"=0, "Position"=1, "Velocity"=2, "Current"=3, "Follower"=5, "MotionProfile"=6, "MotionMagic"=7, "MotionProfileArc"=10, "Disabled"=15] ("Control Mode")
            n53 = call <vilib>:"CTRE_Phoenix_MotorControl_Set.vi"("error in (no error)"=w188, "Output"=0.0, "Control Mode"=w191, "PhoenixMotorControlDevRef"=w189) -> ()  [unwired: 6 in, 2 out]
            n54 = call <vilib>:"CTRE_Phoenix_MotorControl_Set.vi"("error in (no error)"=w193, "Output"=0.0, "Control Mode"=w196, "PhoenixMotorControlDevRef"=w194) -> ()  [unwired: 6 in, 2 out]
            n55 = call <vilib>:"WPI_SwitchGetLimitValue.vi"("error in (no error)"=w226, "SwitchDevRef"=w225) -> ("error out"=w205:errorcluster, "Switch Pressed"=w224:bool, "SwitchDevRef"=w206:T4)  [unwired: 7 in]
            "Orange Limit Pressed 13" <- w224
            n56 = call <vilib>:"WPI_SwitchGetLimitValue.vi"("error in (no error)"=w228, "SwitchDevRef"=w227) -> ("error out"=w207:errorcluster, "Switch Pressed"=w223:bool, "SwitchDevRef"=w208:T4)  [unwired: 7 in]
            "Blue Limit Pressed 13" <- w223
            n57 = global write "AutonBoolean.vi" "Boolean"(FALSE ("Boolean")) -> ()
            n58 = call-poly <vilib>:"NT Read Value.vi"("Default Value"=0.0, "Name"="/limelight-drtrain/ty") -> ("Numeric"=w218:dbl)  [unwired: 8 in, 1 out]
            "Ty 29" <- w218
            n59 = Greater?(x=w214, y=5) -> (0:w213:bool)
            n60 = call "Turret_Aim.vi"("View Button"=FALSE ("Driver Right Thumb"), "Left Trigger"=2.0, "Orange Limit Pressed"=w223, "Blue Limit Pressed"=w224, "Right Bumper"=FALSE, "Left Bumper"=FALSE) -> ()  [unwired: 6 in]
            n61 = call "Shooter_Equation.vi"("Right Trigger"=2.0, "Ty"=w218) -> ()  [unwired: 10 in]
            n62 = Wait (ms)(milliseconds to wait=u32 100) -> ()  [unwired: 1 out]
            n63 = call "Drive_Vi.vi"("Middle Thumb"=FALSE, "Z"=0.0, "Y"=0.15, "X"=0.0) -> ()  [unwired: 8 in]
            n64 = call <vilib>:"CTRE_Phoenix_MotorControl_Set.vi"("error in (no error)"=w199, "Output"=0.0, "Control Mode"=w198, "PhoenixMotorControlDevRef"=w200) -> ("error out"=w201:errorcluster, "PhoenixMotorControlDevRef"=w202:T7)  [unwired: 6 in]
          }
          n65 = while {
            tunnel: w50 -> [w185]
            tunnel: w51 -> [w184]
            tunnel: w48 -> [w183]
            tunnel: w47 -> [w170]
            tunnel: w46 -> [w169]
            tunnel: w44 -> [w168]
            tunnel: w45 -> [w167]
            tunnel: w49 -> [w158]
            tunnel: [w157] -> w37
            tunnel: [w156] -> w38
            tunnel: [w155] -> w36
            tunnel: [w154] -> w35
            tunnel: w24 -> [w151]
            tunnel: w23 -> [w150]
            tunnel: [w151] -> w22
            tunnel: [w150] -> w21
            i -> [w172]
            stop <- w171 stop-if-true
            w153 = T11 0 items=["PercentOutput"=0, "Position"=1, "Velocity"=2, "Current"=3, "Follower"=5, "MotionProfile"=6, "MotionMagic"=7, "MotionProfileArc"=10, "Disabled"=15] ("Control Mode")
            w165 = T11 0 items=["PercentOutput"=0, "Position"=1, "Velocity"=2, "Current"=3, "Follower"=5, "MotionProfile"=6, "MotionMagic"=7, "MotionProfileArc"=10, "Disabled"=15] ("Control Mode")
            w166 = T11 0 items=["PercentOutput"=0, "Position"=1, "Velocity"=2, "Current"=3, "Follower"=5, "MotionProfile"=6, "MotionMagic"=7, "MotionProfileArc"=10, "Disabled"=15] ("Control Mode")
            # "Elevate?"
            n66 = call <vilib>:"CTRE_Phoenix_MotorControl_Set.vi"("error in (no error)"=w150, "Output"=-1.0, "Control Mode"=w153, "PhoenixMotorControlDevRef"=w151) -> ()  [unwired: 6 in, 2 out]
            n67 = call <vilib>:"WPI_SwitchGetLimitValue.vi"("error in (no error)"=w183, "SwitchDevRef"=w158) -> ("Switch Pressed"=w182:bool)  [unwired: 7 in, 2 out]
            "Orange Limit Pressed 14" <- w182
            n68 = call <vilib>:"WPI_SwitchGetLimitValue.vi"("error in (no error)"=w185, "SwitchDevRef"=w184) -> ("Switch Pressed"=w181:bool)  [unwired: 7 in, 2 out]
            "Blue Limit Pressed 14" <- w181
            n69 = call-poly <vilib>:"NT Read Value.vi"("Default Value"=0.0, "Name"="/limelight-drtrain/ty") -> ("Numeric"=w176:dbl)  [unwired: 8 in, 1 out]
            "Ty 30" <- w176
            n70 = Greater?(x=w172, y=50) -> (0:w171:bool)
            n71 = call "Shooter_Equation.vi"("Right Trigger"=2.0, "Ty"=w176) -> ()  [unwired: 10 in]
            n72 = Wait (ms)(milliseconds to wait=u32 100) -> ()  [unwired: 1 out]
            n73 = call "Turret_Aim.vi"("View Button"=FALSE ("Driver Right Thumb"), "Left Trigger"=2.0, "Orange Limit Pressed"=w181, "Blue Limit Pressed"=w182, "Right Bumper"=FALSE, "Left Bumper"=FALSE) -> ()  [unwired: 6 in]
            n74 = call "Drive_Vi.vi"("Middle Thumb"=FALSE, "Z"=0.0, "Y"=0.15, "X"=0.0) -> ()  [unwired: 8 in]
            n75 = call <vilib>:"CTRE_Phoenix_MotorControl_Set.vi"("error in (no error)"=w168, "Output"=0.35, "Control Mode"=w165, "PhoenixMotorControlDevRef"=w167) -> ("error out"=w157:errorcluster, "PhoenixMotorControlDevRef"=w156:T7)  [unwired: 6 in]
            n76 = call <vilib>:"CTRE_Phoenix_MotorControl_Set.vi"("error in (no error)"=w170, "Output"=-0.35, "Control Mode"=w166, "PhoenixMotorControlDevRef"=w169) -> ("error out"=w154:errorcluster, "PhoenixMotorControlDevRef"=w155:T7)  [unwired: 6 in]
          }
          n77 = while {
            tunnel: w35 -> [w125]
            tunnel: w36 -> [w124]
            tunnel: w37 -> [w123]
            tunnel: w38 -> [w122]
            tunnel: [w113] -> w33
            tunnel: [w112] -> w34
            tunnel: [w111] -> w32
            tunnel: [w110] -> w31
            tunnel: w22 -> [w107]
            tunnel: w21 -> [w106]
            i -> [w127]
            stop <- w126 stop-if-true
            w109 = T11 0 items=["PercentOutput"=0, "Position"=1, "Velocity"=2, "Current"=3, "Follower"=5, "MotionProfile"=6, "MotionMagic"=7, "MotionProfileArc"=10, "Disabled"=15] ("Control Mode")
            w120 = T11 0 items=["PercentOutput"=0, "Position"=1, "Velocity"=2, "Current"=3, "Follower"=5, "MotionProfile"=6, "MotionMagic"=7, "MotionProfileArc"=10, "Disabled"=15] ("Control Mode")
            w121 = T11 0 items=["PercentOutput"=0, "Position"=1, "Velocity"=2, "Current"=3, "Follower"=5, "MotionProfile"=6, "MotionMagic"=7, "MotionProfileArc"=10, "Disabled"=15] ("Control Mode")
            n78 = call <vilib>:"CTRE_Phoenix_MotorControl_Set.vi"("error in (no error)"=w106, "Output"=0.0, "Control Mode"=w109, "PhoenixMotorControlDevRef"=w107) -> ()  [unwired: 6 in, 2 out]
            n79 = call-poly <vilib>:"NT Read Value.vi"("Default Value"=0.0, "Name"="/limelight-drtrain/ty") -> ("Numeric"=w131:dbl)  [unwired: 8 in, 1 out]
            "Ty 31" <- w131
            n80 = Greater?(x=w127, y=10) -> (0:w126:bool)
            n81 = call "Shooter_Equation.vi"("Right Trigger"=0.0, "Ty"=w131) -> ()  [unwired: 10 in]
            n82 = Wait (ms)(milliseconds to wait=u32 112) -> ()  [unwired: 1 out]
            n83 = call "Drive_Vi.vi"("Middle Thumb"=FALSE, "Z"=0.35, "Y"=0.0, "X"=0.0) -> ()  [unwired: 8 in]
            n84 = call <vilib>:"CTRE_Phoenix_MotorControl_Set.vi"("error in (no error)"=w123, "Output"=0.35, "Control Mode"=w120, "PhoenixMotorControlDevRef"=w122) -> ("error out"=w113:errorcluster, "PhoenixMotorControlDevRef"=w112:T7)  [unwired: 6 in]
            n85 = call <vilib>:"CTRE_Phoenix_MotorControl_Set.vi"("error in (no error)"=w125, "Output"=-0.35, "Control Mode"=w121, "PhoenixMotorControlDevRef"=w124) -> ("error out"=w110:errorcluster, "PhoenixMotorControlDevRef"=w111:T7)  [unwired: 6 in]
          }
          n86 = while {
            tunnel: w31 -> [w97]
            tunnel: w32 -> [w96]
            tunnel: w33 -> [w95]
            tunnel: w34 -> [w94]
            tunnel: [w85] -> w28
            tunnel: [w84] -> w30
            tunnel: [w83] -> w29
            tunnel: [w82] -> w27
            i -> [w99]
            stop <- w98 stop-if-true
            w92 = T11 0 items=["PercentOutput"=0, "Position"=1, "Velocity"=2, "Current"=3, "Follower"=5, "MotionProfile"=6, "MotionMagic"=7, "MotionProfileArc"=10, "Disabled"=15] ("Control Mode")
            w93 = T11 0 items=["PercentOutput"=0, "Position"=1, "Velocity"=2, "Current"=3, "Follower"=5, "MotionProfile"=6, "MotionMagic"=7, "MotionProfileArc"=10, "Disabled"=15] ("Control Mode")
            n87 = call-poly <vilib>:"NT Read Value.vi"("Default Value"=0.0, "Name"="/limelight-drtrain/ty") -> ("Numeric"=w103:dbl)  [unwired: 8 in, 1 out]
            "Ty 32" <- w103
            n88 = Greater?(x=w99, y=2) -> (0:w98:bool)
            n89 = call "Shooter_Equation.vi"("Right Trigger"=0.0, "Ty"=w103) -> ()  [unwired: 10 in]
            n90 = Wait (ms)(milliseconds to wait=u32 20) -> ()  [unwired: 1 out]
            n91 = call "Drive_Vi.vi"("Middle Thumb"=TRUE, "Z"=0.0, "Y"=0.0, "X"=0.0) -> ()  [unwired: 8 in]
            n92 = call <vilib>:"CTRE_Phoenix_MotorControl_Set.vi"("error in (no error)"=w95, "Output"=0.35, "Control Mode"=w92, "PhoenixMotorControlDevRef"=w94) -> ("error out"=w85:errorcluster, "PhoenixMotorControlDevRef"=w84:T7)  [unwired: 6 in]
            n93 = call <vilib>:"CTRE_Phoenix_MotorControl_Set.vi"("error in (no error)"=w97, "Output"=-0.35, "Control Mode"=w93, "PhoenixMotorControlDevRef"=w96) -> ("error out"=w82:errorcluster, "PhoenixMotorControlDevRef"=w83:T7)  [unwired: 6 in]
          }
          n94 = while {
            tunnel: w28 -> [w145]
            tunnel: w30 -> [w144]
            tunnel: w29 -> [w143]
            tunnel: w27 -> [w142]
            i -> [w140]
            stop <- w139 stop-if-true
            w148 = T11 0 items=["PercentOutput"=0, "Position"=1, "Velocity"=2, "Current"=3, "Follower"=5, "MotionProfile"=6, "MotionMagic"=7, "MotionProfileArc"=10, "Disabled"=15] ("Control Mode")
            w149 = T11 0 items=["PercentOutput"=0, "Position"=1, "Velocity"=2, "Current"=3, "Follower"=5, "MotionProfile"=6, "MotionMagic"=7, "MotionProfileArc"=10, "Disabled"=15] ("Control Mode")
            n95 = call <vilib>:"CTRE_Phoenix_MotorControl_Set.vi"("error in (no error)"=w145, "Output"=0.0, "Control Mode"=w148, "PhoenixMotorControlDevRef"=w144) -> ()  [unwired: 6 in, 2 out]
            n96 = call <vilib>:"CTRE_Phoenix_MotorControl_Set.vi"("error in (no error)"=w142, "Output"=0.0, "Control Mode"=w149, "PhoenixMotorControlDevRef"=w143) -> ()  [unwired: 6 in, 2 out]
            n97 = call "Drive_Vi.vi"("Middle Thumb"=FALSE, "Z"=0.0, "Y"=0.0, "X"=0.0) -> ()  [unwired: 8 in]
            n98 = Greater?(x=w140, y=50) -> (0:w139:bool)
            n99 = Wait (ms)(milliseconds to wait=u32 100) -> ()  [unwired: 1 out]
          }
        }
        frame "1 Ball Plus Reject" {
          # "Pigeon Set"
          n100 = while {
            i -> [w460]
            stop <- w461 stop-if-true
            n101 = Wait (ms)(milliseconds to wait=u32 20) -> ()  [unwired: 1 out]
            n102 = Greater?(x=w460, y=2) -> (0:w461:bool)
            n103 = call "Drive_Vi.vi"("Middle Thumb"=TRUE, "Z"=0.0, "Y"=0.0, "X"=0.0) -> ()  [unwired: 8 in]
          }
          n104 = call <vilib>:"CTRE_Phoenix_MotorControl_RefNumRegistryGet.vi"("refnum name"="Intake Actuate") -> ("error out"=w359:errorcluster, "PhoenixMotorControlDevRef"=w363:T7)  [unwired: 9 in]
          n105 = call <vilib>:"CTRE_Phoenix_MotorControl_RefNumRegistryGet.vi"("refnum name"="Intake") -> ("error out"=w351:errorcluster, "PhoenixMotorControlDevRef"=w355:T7)  [unwired: 9 in]
          n106 = call <vilib>:"CTRE_Phoenix_MotorControl_RefNumRegistryGet.vi"("refnum name"="Reject") -> ("error out"=w343:errorcluster, "PhoenixMotorControlDevRef"=w347:T7)  [unwired: 9 in]
          n107 = call <vilib>:"CTRE_Phoenix_MotorControl_RefNumRegistryGet.vi"("refnum name"="Elevate") -> ("error out"=w335:errorcluster, "PhoenixMotorControlDevRef"=w339:T7)  [unwired: 9 in]
          n108 = call <vilib>:"CTRE_Phoenix_MotorControl_RefNumRegistryGet.vi"("refnum name"="Shoot") -> ("error out"=w317:errorcluster, "PhoenixMotorControlDevRef"=w322:T7)  [unwired: 9 in]
          n109 = while {
            tunnel: [w447] -> w362
            tunnel: w363 -> [w447]
            tunnel: [w446] -> w358
            tunnel: w359 -> [w446]
            tunnel: [w437] -> w354
            tunnel: w355 -> [w440]
            tunnel: [w436] -> w350
            tunnel: w351 -> [w438]
            tunnel: [w445] -> w346
            tunnel: w347 -> [w445]
            tunnel: [w444] -> w342
            tunnel: w343 -> [w444]
            tunnel: [w443] -> w338
            tunnel: w339 -> [w443]
            tunnel: w335 -> [w442]
            tunnel: [w442] -> w334
            tunnel: [w431] -> w321
            tunnel: w322 -> [w433]
            tunnel: w317 -> [w432]
            tunnel: [w430] -> w316
            i -> [w450]
            stop <- w448 stop-if-true
            w435 = T11 0 items=["PercentOutput"=0, "Position"=1, "Velocity"=2, "Current"=3, "Follower"=5, "MotionProfile"=6, "MotionMagic"=7, "MotionProfileArc"=10, "Disabled"=15] ("Control Mode")
            w441 = T11 0 items=["PercentOutput"=0, "Position"=1, "Velocity"=2, "Current"=3, "Follower"=5, "MotionProfile"=6, "MotionMagic"=7, "MotionProfileArc"=10, "Disabled"=15] ("Control Mode")
            # "Wind Up Shooter"
            # "Intake On"
            # "Move"
            # "Move Backwards"
            n110 = call "Drive_Vi.vi"("Middle Thumb"=FALSE, "Z"=0.0, "Y"=-0.15, "X"=0.0) -> ()  [unwired: 8 in]
            n111 = call <vilib>:"CTRE_Phoenix_MotorControl_Set.vi"("error in (no error)"=w432, "Output"=0.25, "Control Mode"=w435, "PhoenixMotorControlDevRef"=w433) -> ("error out"=w430:errorcluster, "PhoenixMotorControlDevRef"=w431:T7)  [unwired: 6 in]
            n112 = call <vilib>:"CTRE_Phoenix_MotorControl_Set.vi"("error in (no error)"=w438, "Output"=1.0, "Control Mode"=w441, "PhoenixMotorControlDevRef"=w440) -> ("error out"=w436:errorcluster, "PhoenixMotorControlDevRef"=w437:T7)  [unwired: 6 in]
            n113 = Greater?(x=w450, y=20) -> (0:w448:bool)
          }
          n114 = while {
            tunnel: [w429] -> w361
            tunnel: w362 -> [w429]
            tunnel: w358 -> [w428]
            tunnel: [w428] -> w357
            tunnel: w354 -> [w427]
            tunnel: [w427] -> w353
            tunnel: w350 -> [w426]
            tunnel: [w426] -> w349
            tunnel: w346 -> [w425]
            tunnel: [w425] -> w345
            tunnel: [w424] -> w341
            tunnel: w342 -> [w424]
            tunnel: [w423] -> w337
            tunnel: w338 -> [w423]
            tunnel: w334 -> [w422]
            tunnel: [w422] -> w333
            tunnel: w321 -> [w421]
            tunnel: [w421] -> w320
            tunnel: w316 -> [w420]
            tunnel: [w420] -> w315
            i -> [w417]
            stop <- w418 stop-if-true
            # "Shoot"
            n115 = Greater?(x=w417, y=20) -> (0:w418:bool)
          }
          n116 = while {
            tunnel: w361 -> [w416]
            tunnel: [w416] -> w360
            tunnel: [w415] -> w356
            tunnel: w357 -> [w415]
            tunnel: w353 -> [w414]
            tunnel: [w414] -> w352
            tunnel: w349 -> [w413]
            tunnel: [w413] -> w348
            tunnel: w345 -> [w412]
            tunnel: [w412] -> w344
            tunnel: [w411] -> w340
            tunnel: w341 -> [w411]
            tunnel: [w410] -> w336
            tunnel: w337 -> [w410]
            tunnel: w333 -> [w409]
            tunnel: [w409] -> w332
            tunnel: w320 -> [w408]
            tunnel: [w408] -> w319
            tunnel: w315 -> [w407]
            tunnel: [w407] -> w314
            i -> [w405]
            stop <- w404 stop-if-true
            # "Pickup + Reject"
            n117 = Greater?(x=w405, y=20) -> (0:w404:bool)
          }
          n118 = while {
            tunnel: w360 -> [w403]
            tunnel: [w403] -> w331
            tunnel: w356 -> [w402]
            tunnel: [w402] -> w330
            tunnel: w352 -> [w401]
            tunnel: [w401] -> w329
            tunnel: w348 -> [w400]
            tunnel: [w400] -> w328
            tunnel: w344 -> [w399]
            tunnel: [w399] -> w327
            tunnel: [w398] -> w326
            tunnel: w340 -> [w398]
            tunnel: [w397] -> w325
            tunnel: w336 -> [w397]
            tunnel: w332 -> [w396]
            tunnel: [w396] -> w324
            tunnel: w319 -> [w395]
            tunnel: [w395] -> w318
            tunnel: [w394] -> w313
            tunnel: w314 -> [w394]
            i -> [w391]
            stop <- w392 stop-if-true
            # "Turn Around and Reset Pidgeon"
            n119 = Greater?(x=w391, y=20) -> (0:w392:bool)
          }
          n120 = while {
            tunnel: w331 -> [w390]
            tunnel: w330 -> [w387]
            tunnel: w329 -> [w386]
            tunnel: w328 -> [w385]
            tunnel: w327 -> [w380]
            tunnel: w326 -> [w379]
            tunnel: w325 -> [w378]
            tunnel: w324 -> [w377]
            tunnel: w318 -> [w372]
            tunnel: w313 -> [w371]
            i -> [w369]
            stop <- w368 stop-if-true
            w374 = T11 0 items=["PercentOutput"=0, "Position"=1, "Velocity"=2, "Current"=3, "Follower"=5, "MotionProfile"=6, "MotionMagic"=7, "MotionProfileArc"=10, "Disabled"=15] ("Control Mode")
            w376 = T11 0 items=["PercentOutput"=0, "Position"=1, "Velocity"=2, "Current"=3, "Follower"=5, "MotionProfile"=6, "MotionMagic"=7, "MotionProfileArc"=10, "Disabled"=15] ("Control Mode")
            w382 = T11 0 items=["PercentOutput"=0, "Position"=1, "Velocity"=2, "Current"=3, "Follower"=5, "MotionProfile"=6, "MotionMagic"=7, "MotionProfileArc"=10, "Disabled"=15] ("Control Mode")
            w384 = T11 0 items=["PercentOutput"=0, "Position"=1, "Velocity"=2, "Current"=3, "Follower"=5, "MotionProfile"=6, "MotionMagic"=7, "MotionProfileArc"=10, "Disabled"=15] ("Control Mode")
            w388 = T11 0 items=["PercentOutput"=0, "Position"=1, "Velocity"=2, "Current"=3, "Follower"=5, "MotionProfile"=6, "MotionMagic"=7, "MotionProfileArc"=10, "Disabled"=15] ("Control Mode")
            # "Reset"
            n121 = call <vilib>:"CTRE_Phoenix_MotorControl_Set.vi"("error in (no error)"=w387, "Output"=0.0, "Control Mode"=w388, "PhoenixMotorControlDevRef"=w390) -> ()  [unwired: 6 in, 2 out]
            n122 = call <vilib>:"CTRE_Phoenix_MotorControl_Set.vi"("error in (no error)"=w385, "Output"=0.0, "Control Mode"=w384, "PhoenixMotorControlDevRef"=w386) -> ()  [unwired: 6 in, 2 out]
            n123 = call <vilib>:"CTRE_Phoenix_MotorControl_Set.vi"("error in (no error)"=w379, "Output"=0.0, "Control Mode"=w382, "PhoenixMotorControlDevRef"=w380) -> ()  [unwired: 6 in, 2 out]
            n124 = call <vilib>:"CTRE_Phoenix_MotorControl_Set.vi"("error in (no error)"=w377, "Output"=0.0, "Control Mode"=w376, "PhoenixMotorControlDevRef"=w378) -> ()  [unwired: 6 in, 2 out]
            n125 = call <vilib>:"CTRE_Phoenix_MotorControl_Set.vi"("error in (no error)"=w371, "Output"=0.0, "Control Mode"=w374, "PhoenixMotorControlDevRef"=w372) -> ()  [unwired: 6 in, 2 out]
            n126 = Greater?(x=w369, y=20) -> (0:w368:bool)
          }
        }
        frame "Taxi + Shoot 1" {
          # "Pigeon Set"
          n127 = call <vilib>:"WPI_SwitchRefNum Registry Get.vi"("refnum name"="Intake Sensor") -> ("error out"=w467:errorcluster, "SwitchDevRef"=w469:T4)  [unwired: 9 in]
          n128 = call <vilib>:"WPI_SolenoidRefNum Registry Get.vi"("refnum name"="Intake Solenoid") -> ("error out"=w486:errorcluster, "SolenoidDevRef"=w488:T12)  [unwired: 9 in]
          n129 = call <vilib>:"CTRE_Phoenix_MotorControl_RefNumRegistryGet.vi"("refnum name"="Intake") -> ("error out"=w481:errorcluster, "PhoenixMotorControlDevRef"=w483:T7)  [unwired: 9 in]
          n130 = call <vilib>:"CTRE_Phoenix_MotorControl_RefNumRegistryGet.vi"("refnum name"="Reject") -> ("error out"=w517:errorcluster, "PhoenixMotorControlDevRef"=w479:T7)  [unwired: 9 in]
          n131 = call "Limit_Switches.vi"() -> ()  [unwired: 10 in, 2 out]
          n132 = call <vilib>:"CTRE_Phoenix_MotorControl_RefNumRegistryGet.vi"("refnum name"="Elevate") -> ("error out"=w475:errorcluster, "PhoenixMotorControlDevRef"=w477:T7)  [unwired: 9 in]
          n133 = call <vilib>:"WPI_SwitchRefNum Registry Get.vi"("refnum name"="Elevate Sensor") -> ("error out"=w471:errorcluster, "SwitchDevRef"=w473:T4)  [unwired: 9 in]
          n134 = call <vilib>:"CTRE_Phoenix_MotorControl_RefNumRegistryGet.vi"("refnum name"="Shoot") -> ("error out"=w463:errorcluster, "PhoenixMotorControlDevRef"=w466:T7)  [unwired: 9 in]
          n135 = while {
            tunnel: [w541] -> w487
            tunnel: w488 -> [w541]
            tunnel: [w540] -> w485
            tunnel: w486 -> [w540]
            tunnel: [w539] -> w484
            tunnel: w483 -> [w539]
            tunnel: [w538] -> w482
            tunnel: w481 -> [w538]
            tunnel: [w537] -> w480
            tunnel: w479 -> [w537]
            tunnel: [w536] -> w478
            tunnel: w477 -> [w536]
            tunnel: [w535] -> w476
            tunnel: w475 -> [w535]
            tunnel: [w534] -> w474
            tunnel: w473 -> [w534]
            tunnel: [w533] -> w472
            tunnel: w471 -> [w533]
            tunnel: [w532] -> w470
            tunnel: w469 -> [w532]
            tunnel: [w531] -> w468
            tunnel: w467 -> [w531]
            tunnel: [w530] -> w465
            tunnel: w466 -> [w530]
            tunnel: [w529] -> w464
            tunnel: w463 -> [w529]
            i -> [w525]
            stop <- w527 stop-if-true
            n136 = Wait (ms)(milliseconds to wait=u32 100) -> ()  [unwired: 1 out]
            n137 = call "Drive_Vi.vi"("Middle Thumb"=FALSE, "Z"=0.0, "Y"=0.0, "X"=0.0) -> ()  [unwired: 8 in]
            n138 = Greater?(x=w525, y=100) -> (0:w527:bool)
          }
          n139 = while {
            i -> [w715]
            stop <- w716 stop-if-true
            n140 = Wait (ms)(milliseconds to wait=u32 20) -> ()  [unwired: 1 out]
            n141 = Greater?(x=w715, y=2) -> (0:w716:bool)
            n142 = call "Drive_Vi.vi"("Middle Thumb"=TRUE, "Z"=0.0, "Y"=0.0, "X"=0.0) -> ()  [unwired: 8 in]
          }
          n143 = while {
            tunnel: w472 -> [w670]
            tunnel: w474 -> [w669]
            tunnel: w468 -> [w668]
            tunnel: w470 -> [w667]
            tunnel: w485 -> [w666]
            tunnel: w487 -> [w665]
            tunnel: w476 -> [w662]
            tunnel: w478 -> [w661]
            tunnel: w517 -> [w660]
            tunnel: w480 -> [w659]
            tunnel: w482 -> [w658]
            tunnel: w484 -> [w657]
            tunnel: [w645] -> w510
            tunnel: [w644] -> w509
            tunnel: [w643] -> w508
            tunnel: [w642] -> w507
            tunnel: w464 -> [w641]
            tunnel: w465 -> [w640]
            tunnel: [w637] -> w506
            tunnel: [w636] -> w505
            tunnel: [w635] -> w498
            tunnel: [w634] -> w497
            i -> [w673]
            stop <- w674 stop-if-true
            w639 = T11 0 items=["PercentOutput"=0, "Position"=1, "Velocity"=2, "Current"=3, "Follower"=5, "MotionProfile"=6, "MotionMagic"=7, "MotionProfileArc"=10, "Disabled"=15] ("Control Mode")
            w651 = T11 0 items=["PercentOutput"=0, "Position"=1, "Velocity"=2, "Current"=3, "Follower"=5, "MotionProfile"=6, "MotionMagic"=7, "MotionProfileArc"=10, "Disabled"=15] ("Control Mode")
            w652 = T11 0 items=["PercentOutput"=0, "Position"=1, "Velocity"=2, "Current"=3, "Follower"=5, "MotionProfile"=6, "MotionMagic"=7, "MotionProfileArc"=10, "Disabled"=15] ("Control Mode")
            w653 = T11 0 items=["PercentOutput"=0, "Position"=1, "Velocity"=2, "Current"=3, "Follower"=5, "MotionProfile"=6, "MotionMagic"=7, "MotionProfileArc"=10, "Disabled"=15] ("Control Mode")
            n144 = call <vilib>:"WPI_SwitchGetLimitValue.vi"("error in (no error)"=w668, "SwitchDevRef"=w667) -> ("Switch Pressed"=w671:bool)  [unwired: 7 in, 2 out]
            n145 = call <vilib>:"WPI_SwitchGetLimitValue.vi"("error in (no error)"=w670, "SwitchDevRef"=w669) -> ("Switch Pressed"=w672:bool)  [unwired: 7 in, 2 out]
            n146 = Greater?(x=w673, y=20) -> (0:w674:bool)
            n147 = Not(x=w671) -> (.not. x?=w656:bool)
            "Intake 6" <- w656
            n148 = Not(x=w672) -> (.not. x?=w664:bool)
            "Elevate 6" <- w664
            n149 = Wait (ms)(milliseconds to wait=u32 100) -> ()  [unwired: 1 out]
            n150 = case shown="True" w664 {
              tunnel: [0.75 ("Output") w693] -> w663
              tunnel: w656 -> [_ w690]
              tunnel: [0.75 ("Output") w692] -> w655
              tunnel: [-0.1 ("Output") w691] -> w654
              tunnel: [FALSE ("Middle Thumb") w689] -> w650
              tunnel: [0.0 ("Z") w688] -> w649
              tunnel: [0.0 ("Y") w687] -> w648
              tunnel: [0.0 ("X") w686] -> w647
              tunnel: [WPI_SolenoidValue."Reverse" ("Value") w685] -> w646
              frame False {
              }
              frame True {
                n151 = case shown="False" w690 {
                  tunnel: [0.75 ("Output") 0.0 ("Output")] -> w693
                  tunnel: [0.0 ("Output") 0.0 ("Output")] -> w692
                  tunnel: [0.0 ("Output") 0.0 ("Output")] -> w691
                  tunnel: [FALSE ("Middle Thumb") FALSE ("Middle Thumb")] -> w689
                  tunnel: [0.0 ("Z") 0.0 ("Z")] -> w688
                  tunnel: [-0.3 ("Y") 0.0 ("Y")] -> w687
                  tunnel: [0.0 ("X") 0.0 ("X")] -> w686
                  tunnel: [WPI_SolenoidValue."Forward" ("Value") WPI_SolenoidValue."Forward" ("Value")] -> w685
                  frame False {
                  }
                  frame True {
                  }
                }
              }
            }
            n152 = call-poly <vilib>:"WPI_SolenoidSet.vi"("error in (no error)"=w666, "Value"=w646, "SolenoidDevRef"=w665) -> ("error out"=w634:errorcluster, "SolenoidDevRef"=w635:T12)  [unwired: 7 in]
            n153 = call <vilib>:"CTRE_Phoenix_MotorControl_Set.vi"("error in (no error)"=w658, "Output"=w663, "Control Mode"=w651, "PhoenixMotorControlDevRef"=w657) -> ("error out"=w643:errorcluster, "PhoenixMotorControlDevRef"=w642:T7)  [unwired: 6 in]
            n154 = call <vilib>:"CTRE_Phoenix_MotorControl_Set.vi"("error in (no error)"=w660, "Output"=w655, "Control Mode"=w652, "PhoenixMotorControlDevRef"=w659) -> ()  [unwired: 6 in, 2 out]
            n155 = call <vilib>:"CTRE_Phoenix_MotorControl_Set.vi"("error in (no error)"=w662, "Output"=w654, "Control Mode"=w653, "PhoenixMotorControlDevRef"=w661) -> ("error out"=w645:errorcluster, "PhoenixMotorControlDevRef"=w644:T7)  [unwired: 6 in]
            n156 = call <vilib>:"CTRE_Phoenix_MotorControl_Set.vi"("error in (no error)"=w641, "Output"=-0.55, "Control Mode"=w639, "PhoenixMotorControlDevRef"=w640) -> ("error out"=w637:errorcluster, "PhoenixMotorControlDevRef"=w636:T7)  [unwired: 6 in]
            n157 = call "Drive_Vi.vi"("Middle Thumb"=w650, "Z"=w649, "Y"=w648, "X"=w647) -> ()  [unwired: 8 in]
          }
          n158 = call <vilib>:"WPI_SwitchRefNum Registry Get.vi"("refnum name"="Orange Limit Switch") -> ("error out"=w512:errorcluster, "SwitchDevRef"=w511:T4)  [unwired: 9 in]
          n159 = call <vilib>:"WPI_SwitchRefNum Registry Get.vi"("refnum name"="Blue Limit Switch") -> ("error out"=w514:errorcluster, "SwitchDevRef"=w513:T4)  [unwired: 9 in]
          n160 = while {
            tunnel: w506 -> [_]
            tunnel: w505 -> [_]
            tunnel: w514 -> [w631]
            tunnel: w513 -> [w630]
            tunnel: w512 -> [w629]
            tunnel: w511 -> [w628]
            tunnel: w510 -> [w607]
            tunnel: w509 -> [w606]
            tunnel: w508 -> [w597]
            tunnel: w507 -> [w598]
            tunnel: [w611] -> w504
            tunnel: [w610] -> w503
            tunnel: [w609] -> w502
            tunnel: [w608] -> w501
            tunnel: [w607] -> w500
            tunnel: [w606] -> w499
            tunnel: w498 -> [w605]
            tunnel: w497 -> [w604]
            tunnel: [w602] -> w496
            tunnel: [w601] -> w495
            tunnel: [w600] -> w494
            tunnel: [w599] -> w493
            i -> [w617]
            stop <- w616 stop-if-true
            w596 = T11 0 items=["PercentOutput"=0, "Position"=1, "Velocity"=2, "Current"=3, "Follower"=5, "MotionProfile"=6, "MotionMagic"=7, "MotionProfileArc"=10, "Disabled"=15] ("Control Mode")
            n161 = call-poly <vilib>:"WPI_SolenoidSet.vi"("error in (no error)"=w604, "Value"=WPI_SolenoidValue."Forward", "SolenoidDevRef"=w605) -> ("error out"=w601:errorcluster, "SolenoidDevRef"=w602:T12)  [unwired: 7 in]
            n162 = call <vilib>:"WPI_SwitchGetLimitValue.vi"("error in (no error)"=w629, "SwitchDevRef"=w628) -> ("error out"=w608:errorcluster, "Switch Pressed"=w627:bool, "SwitchDevRef"=w609:T4)  [unwired: 7 in]
            "Orange Limit Pressed 12" <- w627
            n163 = call <vilib>:"WPI_SwitchGetLimitValue.vi"("error in (no error)"=w631, "SwitchDevRef"=w630) -> ("error out"=w610:errorcluster, "Switch Pressed"=w626:bool, "SwitchDevRef"=w611:T4)  [unwired: 7 in]
            "Blue Limit Pressed 12" <- w626
            n164 = call-poly <vilib>:"NT Read Value.vi"("Default Value"=0.0, "Name"="/limelight-drtrain/ty") -> ("Numeric"=w621:dbl)  [unwired: 8 in, 1 out]
            "Ty 26" <- w621
            n165 = Greater?(x=w617, y=5) -> (0:w616:bool)
            n166 = call "Turret_Aim.vi"("View Button"=FALSE ("Driver Right Thumb"), "Left Trigger"=2.0, "Orange Limit Pressed"=w626, "Blue Limit Pressed"=w627, "Right Bumper"=FALSE, "Left Bumper"=FALSE) -> ()  [unwired: 6 in]
            n167 = call "Shooter_Equation.vi"("Right Trigger"=2.0, "Ty"=w621) -> ()  [unwired: 10 in]
            n168 = Wait (ms)(milliseconds to wait=u32 100) -> ()  [unwired: 1 out]
            n169 = call "Drive_Vi.vi"("Middle Thumb"=FALSE, "Z"=0.0, "Y"=0.15, "X"=0.0) -> ()  [unwired: 8 in]
            n170 = call <vilib>:"CTRE_Phoenix_MotorControl_Set.vi"("error in (no error)"=w597, "Output"=0.0, "Control Mode"=w596, "PhoenixMotorControlDevRef"=w598) -> ("error out"=w599:errorcluster, "PhoenixMotorControlDevRef"=w600:T7)  [unwired: 6 in]
          }
          n171 = while {
            tunnel: w503 -> [w592]
            tunnel: w504 -> [w591]
            tunnel: w501 -> [w590]
            tunnel: w500 -> [w577]
            tunnel: w499 -> [w576]
            tunnel: w493 -> [w575]
            tunnel: w494 -> [w574]
            tunnel: w502 -> [w565]
            tunnel: w496 -> [w564]
            tunnel: w495 -> [w563]
            tunnel: [w561] -> w492
            tunnel: [w560] -> w491
            tunnel: [w559] -> w490
            tunnel: [w558] -> w489
            i -> [w579]
            stop <- w578 stop-if-true
            w572 = T11 0 items=["PercentOutput"=0, "Position"=1, "Velocity"=2, "Current"=3, "Follower"=5, "MotionProfile"=6, "MotionMagic"=7, "MotionProfileArc"=10, "Disabled"=15] ("Control Mode")
            w573 = T11 0 items=["PercentOutput"=0, "Position"=1, "Velocity"=2, "Current"=3, "Follower"=5, "MotionProfile"=6, "MotionMagic"=7, "MotionProfileArc"=10, "Disabled"=15] ("Control Mode")
            n172 = call-poly <vilib>:"WPI_SolenoidSet.vi"("error in (no error)"=w563, "Value"=WPI_SolenoidValue."Off", "SolenoidDevRef"=w564) -> ()  [unwired: 7 in, 2 out]
            n173 = call <vilib>:"WPI_SwitchGetLimitValue.vi"("error in (no error)"=w590, "SwitchDevRef"=w565) -> ("Switch Pressed"=w589:bool)  [unwired: 7 in, 2 out]
            "Orange Limit Pressed 11" <- w589
            n174 = call <vilib>:"WPI_SwitchGetLimitValue.vi"("error in (no error)"=w592, "SwitchDevRef"=w591) -> ("Switch Pressed"=w588:bool)  [unwired: 7 in, 2 out]
            "Blue Limit Pressed 11" <- w588
            n175 = call-poly <vilib>:"NT Read Value.vi"("Default Value"=0.0, "Name"="/limelight-drtrain/ty") -> ("Numeric"=w583:dbl)  [unwired: 8 in, 1 out]
            "Ty 25" <- w583
            n176 = Greater?(x=w579, y=50) -> (0:w578:bool)
            n177 = call "Turret_Aim.vi"("View Button"=FALSE ("Driver Right Thumb"), "Left Trigger"=2.0, "Orange Limit Pressed"=w588, "Blue Limit Pressed"=w589, "Right Bumper"=FALSE, "Left Bumper"=FALSE) -> ()  [unwired: 6 in]
            n178 = call "Shooter_Equation.vi"("Right Trigger"=2.0, "Ty"=w583) -> ()  [unwired: 10 in]
            n179 = Wait (ms)(milliseconds to wait=u32 100) -> ()  [unwired: 1 out]
            n180 = call "Drive_Vi.vi"("Middle Thumb"=FALSE, "Z"=0.0, "Y"=0.15, "X"=0.0) -> ()  [unwired: 8 in]
            n181 = call <vilib>:"CTRE_Phoenix_MotorControl_Set.vi"("error in (no error)"=w575, "Output"=0.35, "Control Mode"=w572, "PhoenixMotorControlDevRef"=w574) -> ("error out"=w561:errorcluster, "PhoenixMotorControlDevRef"=w560:T7)  [unwired: 6 in]
            n182 = call <vilib>:"CTRE_Phoenix_MotorControl_Set.vi"("error in (no error)"=w577, "Output"=-0.35, "Control Mode"=w573, "PhoenixMotorControlDevRef"=w576) -> ("error out"=w558:errorcluster, "PhoenixMotorControlDevRef"=w559:T7)  [unwired: 6 in]
          }
          n183 = while {
            tunnel: w492 -> [w553]
            tunnel: w491 -> [w552]
            tunnel: w490 -> [w551]
            tunnel: w489 -> [w550]
            i -> [w548]
            stop <- w547 stop-if-true
            w556 = T11 0 items=["PercentOutput"=0, "Position"=1, "Velocity"=2, "Current"=3, "Follower"=5, "MotionProfile"=6, "MotionMagic"=7, "MotionProfileArc"=10, "Disabled"=15] ("Control Mode")
            w557 = T11 0 items=["PercentOutput"=0, "Position"=1, "Velocity"=2, "Current"=3, "Follower"=5, "MotionProfile"=6, "MotionMagic"=7, "MotionProfileArc"=10, "Disabled"=15] ("Control Mode")
            n184 = call <vilib>:"CTRE_Phoenix_MotorControl_Set.vi"("error in (no error)"=w553, "Output"=0.0, "Control Mode"=w556, "PhoenixMotorControlDevRef"=w552) -> ()  [unwired: 6 in, 2 out]
            n185 = call <vilib>:"CTRE_Phoenix_MotorControl_Set.vi"("error in (no error)"=w550, "Output"=0.0, "Control Mode"=w557, "PhoenixMotorControlDevRef"=w551) -> ()  [unwired: 6 in, 2 out]
            n186 = Greater?(x=w548, y=50) -> (0:w547:bool)
            n187 = Wait (ms)(milliseconds to wait=u32 100) -> ()  [unwired: 1 out]
          }
        }
        frame "1 Ball + Reject" {
          # "Pigeon Set"
          n188 = while {
            i -> [w936]
            stop <- w937 stop-if-true
            n189 = Wait (ms)(milliseconds to wait=u32 20) -> ()  [unwired: 1 out]
            n190 = Greater?(x=w936, y=2) -> (0:w937:bool)
            n191 = call "Drive_Vi.vi"("Middle Thumb"=TRUE, "Z"=0.0, "Y"=0.0, "X"=0.0) -> ()  [unwired: 8 in]
          }
          n192 = call <vilib>:"WPI_SwitchRefNum Registry Get.vi"("refnum name"="Intake Sensor") -> ("error out"=w757:errorcluster, "SwitchDevRef"=w756:T4)  [unwired: 9 in]
          n193 = call <vilib>:"WPI_SolenoidRefNum Registry Get.vi"("refnum name"="Intake Solenoid") -> ("error out"=w755:errorcluster, "SolenoidDevRef"=w754:T12)  [unwired: 9 in]
          n194 = call <vilib>:"CTRE_Phoenix_MotorControl_RefNumRegistryGet.vi"("refnum name"="Intake") -> ("error out"=w749:errorcluster, "PhoenixMotorControlDevRef"=w748:T7)  [unwired: 9 in]
          n195 = call <vilib>:"CTRE_Phoenix_MotorControl_RefNumRegistryGet.vi"("refnum name"="Reject") -> ("error out"=w751:errorcluster, "PhoenixMotorControlDevRef"=w750:T7)  [unwired: 9 in]
          n196 = call "Limit_Switches.vi"() -> ()  [unwired: 10 in, 2 out]
          n197 = call <vilib>:"CTRE_Phoenix_MotorControl_RefNumRegistryGet.vi"("refnum name"="Elevate") -> ("error out"=w753:errorcluster, "PhoenixMotorControlDevRef"=w752:T7)  [unwired: 9 in]
          n198 = call <vilib>:"WPI_SwitchRefNum Registry Get.vi"("refnum name"="Elevate Sensor") -> ("error out"=w759:errorcluster, "SwitchDevRef"=w758:T4)  [unwired: 9 in]
          n199 = call <vilib>:"CTRE_Phoenix_MotorControl_RefNumRegistryGet.vi"("refnum name"="Shoot") -> ("error out"=w737:errorcluster, "PhoenixMotorControlDevRef"=w736:T7)  [unwired: 9 in]
          n200 = while {
            tunnel: w759 -> [w891]
            tunnel: w758 -> [w890]
            tunnel: w757 -> [w889]
            tunnel: w756 -> [w888]
            tunnel: w755 -> [w887]
            tunnel: w754 -> [w886]
            tunnel: w753 -> [w883]
            tunnel: w752 -> [w882]
            tunnel: w751 -> [w881]
            tunnel: w750 -> [w880]
            tunnel: w749 -> [w879]
            tunnel: w748 -> [w878]
            tunnel: [w866] -> w741
            tunnel: [w865] -> w740
            tunnel: [w864] -> w739
            tunnel: [w863] -> w738
            tunnel: w737 -> [w862]
            tunnel: w736 -> [w861]
            tunnel: [w858] -> w735
            tunnel: [w857] -> w734
            tunnel: [w856] -> w727
            tunnel: [w855] -> w726
            i -> [w894]
            stop <- w895 stop-if-true
            w860 = T11 0 items=["PercentOutput"=0, "Position"=1, "Velocity"=2, "Current"=3, "Follower"=5, "MotionProfile"=6, "MotionMagic"=7, "MotionProfileArc"=10, "Disabled"=15] ("Control Mode")
            w872 = T11 0 items=["PercentOutput"=0, "Position"=1, "Velocity"=2, "Current"=3, "Follower"=5, "MotionProfile"=6, "MotionMagic"=7, "MotionProfileArc"=10, "Disabled"=15] ("Control Mode")
            w873 = T11 0 items=["PercentOutput"=0, "Position"=1, "Velocity"=2, "Current"=3, "Follower"=5, "MotionProfile"=6, "MotionMagic"=7, "MotionProfileArc"=10, "Disabled"=15] ("Control Mode")
            w874 = T11 0 items=["PercentOutput"=0, "Position"=1, "Velocity"=2, "Current"=3, "Follower"=5, "MotionProfile"=6, "MotionMagic"=7, "MotionProfileArc"=10, "Disabled"=15] ("Control Mode")
            n201 = call <vilib>:"WPI_SwitchGetLimitValue.vi"("error in (no error)"=w889, "SwitchDevRef"=w888) -> ("Switch Pressed"=w892:bool)  [unwired: 7 in, 2 out]
            n202 = call <vilib>:"WPI_SwitchGetLimitValue.vi"("error in (no error)"=w891, "SwitchDevRef"=w890) -> ("Switch Pressed"=w893:bool)  [unwired: 7 in, 2 out]
            n203 = Greater?(x=w894, y=20) -> (0:w895:bool)
            n204 = Not(x=w892) -> (.not. x?=w877:bool)
            "Intake 8" <- w877
            n205 = Not(x=w893) -> (.not. x?=w885:bool)
            "Elevate 8" <- w885
            n206 = Wait (ms)(milliseconds to wait=u32 100) -> ()  [unwired: 1 out]
            n207 = case shown="True" w885 {
              tunnel: [0.75 ("Output") w914] -> w884
              tunnel: w877 -> [_ w911]
              tunnel: [0.75 ("Output") w913] -> w876
              tunnel: [-0.1 ("Output") w912] -> w875
              tunnel: [FALSE ("Middle Thumb") w910] -> w871
              tunnel: [0.0 ("Z") w909] -> w870
              tunnel: [0.0 ("Y") w908] -> w869
              tunnel: [0.0 ("X") w907] -> w868
              tunnel: [WPI_SolenoidValue."Reverse" ("Value") w906] -> w867
              frame False {
              }
              frame True {
                n208 = case shown="False" w911 {
                  tunnel: [0.75 ("Output") 0.0 ("Output")] -> w914
                  tunnel: [0.75 ("Output") -0.75 ("Output")] -> w913
                  tunnel: [0.0 ("Output") 0.0 ("Output")] -> w912
                  tunnel: [FALSE ("Middle Thumb") FALSE ("Middle Thumb")] -> w910
                  tunnel: [0.0 ("Z") 0.0 ("Z")] -> w909
                  tunnel: [-0.3 ("Y") 0.0 ("Y")] -> w908
                  tunnel: [0.0 ("X") 0.0 ("X")] -> w907
                  tunnel: [WPI_SolenoidValue."Reverse" ("Value") WPI_SolenoidValue."Forward" ("Value")] -> w906
                  frame False {
                  }
                  frame True {
                  }
                }
              }
            }
            n209 = call-poly <vilib>:"WPI_SolenoidSet.vi"("error in (no error)"=w887, "Value"=w867, "SolenoidDevRef"=w886) -> ("error out"=w855:errorcluster, "SolenoidDevRef"=w856:T12)  [unwired: 7 in]
            n210 = call <vilib>:"CTRE_Phoenix_MotorControl_Set.vi"("error in (no error)"=w879, "Output"=w884, "Control Mode"=w872, "PhoenixMotorControlDevRef"=w878) -> ("error out"=w864:errorcluster, "PhoenixMotorControlDevRef"=w863:T7)  [unwired: 6 in]
            n211 = call <vilib>:"CTRE_Phoenix_MotorControl_Set.vi"("error in (no error)"=w881, "Output"=w876, "Control Mode"=w873, "PhoenixMotorControlDevRef"=w880) -> ()  [unwired: 6 in, 2 out]
            n212 = call <vilib>:"CTRE_Phoenix_MotorControl_Set.vi"("error in (no error)"=w883, "Output"=w875, "Control Mode"=w874, "PhoenixMotorControlDevRef"=w882) -> ("error out"=w866:errorcluster, "PhoenixMotorControlDevRef"=w865:T7)  [unwired: 6 in]
            n213 = call <vilib>:"CTRE_Phoenix_MotorControl_Set.vi"("error in (no error)"=w862, "Output"=-0.55, "Control Mode"=w860, "PhoenixMotorControlDevRef"=w861) -> ("error out"=w858:errorcluster, "PhoenixMotorControlDevRef"=w857:T7)  [unwired: 6 in]
            n214 = call "Drive_Vi.vi"("Middle Thumb"=w871, "Z"=w870, "Y"=w869, "X"=w868) -> ()  [unwired: 8 in]
          }
          n215 = call <vilib>:"WPI_SwitchRefNum Registry Get.vi"("refnum name"="Orange Limit Switch") -> ("error out"=w743:errorcluster, "SwitchDevRef"=w742:T4)  [unwired: 9 in]
          n216 = call <vilib>:"WPI_SwitchRefNum Registry Get.vi"("refnum name"="Blue Limit Switch") -> ("error out"=w745:errorcluster, "SwitchDevRef"=w744:T4)  [unwired: 9 in]
          n217 = while {
            tunnel: w735 -> [_]
            tunnel: w734 -> [_]
            tunnel: w745 -> [w852]
            tunnel: w744 -> [w851]
            tunnel: w743 -> [w850]
            tunnel: w742 -> [w849]
            tunnel: w741 -> [w828]
            tunnel: w740 -> [w827]
            tunnel: w739 -> [w818]
            tunnel: w738 -> [w819]
            tunnel: [w832] -> w733
            tunnel: [w831] -> w732
            tunnel: [w830] -> w731
            tunnel: [w829] -> w730
            tunnel: [w828] -> w729
            tunnel: [w827] -> w728
            tunnel: w727 -> [w826]
            tunnel: w726 -> [w825]
            tunnel: [w823] -> w725
            tunnel: [w822] -> w724
            tunnel: [w821] -> w723
            tunnel: [w820] -> w722
            i -> [w838]
            stop <- w837 stop-if-true
            w817 = T11 0 items=["PercentOutput"=0, "Position"=1, "Velocity"=2, "Current"=3, "Follower"=5, "MotionProfile"=6, "MotionMagic"=7, "MotionProfileArc"=10, "Disabled"=15] ("Control Mode")
            n218 = call-poly <vilib>:"WPI_SolenoidSet.vi"("error in (no error)"=w825, "Value"=WPI_SolenoidValue."Forward", "SolenoidDevRef"=w826) -> ("error out"=w822:errorcluster, "SolenoidDevRef"=w823:T12)  [unwired: 7 in]
            n219 = call <vilib>:"WPI_SwitchGetLimitValue.vi"("error in (no error)"=w850, "SwitchDevRef"=w849) -> ("error out"=w829:errorcluster, "Switch Pressed"=w848:bool, "SwitchDevRef"=w830:T4)  [unwired: 7 in]
            "Orange Limit Pressed 16" <- w848
            n220 = call <vilib>:"WPI_SwitchGetLimitValue.vi"("error in (no error)"=w852, "SwitchDevRef"=w851) -> ("error out"=w831:errorcluster, "Switch Pressed"=w847:bool, "SwitchDevRef"=w832:T4)  [unwired: 7 in]
            "Blue Limit Pressed 16" <- w847
            n221 = call-poly <vilib>:"NT Read Value.vi"("Default Value"=0.0, "Name"="/limelight-drtrain/ty") -> ("Numeric"=w842:dbl)  [unwired: 8 in, 1 out]
            "Ty 28" <- w842
            n222 = Greater?(x=w838, y=5) -> (0:w837:bool)
            n223 = call "Turret_Aim.vi"("View Button"=FALSE ("Driver Right Thumb"), "Left Trigger"=2.0, "Orange Limit Pressed"=w847, "Blue Limit Pressed"=w848, "Right Bumper"=FALSE, "Left Bumper"=FALSE) -> ()  [unwired: 6 in]
            n224 = call "Shooter_Equation.vi"("Right Trigger"=2.0, "Ty"=w842) -> ()  [unwired: 10 in]
            n225 = Wait (ms)(milliseconds to wait=u32 100) -> ()  [unwired: 1 out]
            n226 = call "Drive_Vi.vi"("Middle Thumb"=FALSE, "Z"=0.0, "Y"=0.15, "X"=0.0) -> ()  [unwired: 8 in]
            n227 = call <vilib>:"CTRE_Phoenix_MotorControl_Set.vi"("error in (no error)"=w818, "Output"=0.0, "Control Mode"=w817, "PhoenixMotorControlDevRef"=w819) -> ("error out"=w820:errorcluster, "PhoenixMotorControlDevRef"=w821:T7)  [unwired: 6 in]
          }
          n228 = while {
            tunnel: w732 -> [w813]
            tunnel: w733 -> [w812]
            tunnel: w730 -> [w811]
            tunnel: w729 -> [w798]
            tunnel: w728 -> [w797]
            tunnel: w722 -> [w796]
            tunnel: w723 -> [w795]
            tunnel: w731 -> [w786]
            tunnel: w725 -> [w785]
            tunnel: w724 -> [w784]
            tunnel: [w782] -> w721
            tunnel: [w781] -> w720
            tunnel: [w780] -> w719
            tunnel: [w779] -> w718
            i -> [w800]
            stop <- w799 stop-if-true
            w793 = T11 0 items=["PercentOutput"=0, "Position"=1, "Velocity"=2, "Current"=3, "Follower"=5, "MotionProfile"=6, "MotionMagic"=7, "MotionProfileArc"=10, "Disabled"=15] ("Control Mode")
            w794 = T11 0 items=["PercentOutput"=0, "Position"=1, "Velocity"=2, "Current"=3, "Follower"=5, "MotionProfile"=6, "MotionMagic"=7, "MotionProfileArc"=10, "Disabled"=15] ("Control Mode")
            n229 = call-poly <vilib>:"WPI_SolenoidSet.vi"("error in (no error)"=w784, "Value"=WPI_SolenoidValue."Off", "SolenoidDevRef"=w785) -> ()  [unwired: 7 in, 2 out]
            n230 = call <vilib>:"WPI_SwitchGetLimitValue.vi"("error in (no error)"=w811, "SwitchDevRef"=w786) -> ("Switch Pressed"=w810:bool)  [unwired: 7 in, 2 out]
            "Orange Limit Pressed 15" <- w810
            n231 = call <vilib>:"WPI_SwitchGetLimitValue.vi"("error in (no error)"=w813, "SwitchDevRef"=w812) -> ("Switch Pressed"=w809:bool)  [unwired: 7 in, 2 out]
            "Blue Limit Pressed 15" <- w809
            n232 = call-poly <vilib>:"NT Read Value.vi"("Default Value"=0.0, "Name"="/limelight-drtrain/ty") -> ("Numeric"=w804:dbl)  [unwired: 8 in, 1 out]
            "Ty 27" <- w804
            n233 = Greater?(x=w800, y=50) -> (0:w799:bool)
            n234 = call "Turret_Aim.vi"("View Button"=FALSE ("Driver Right Thumb"), "Left Trigger"=2.0, "Orange Limit Pressed"=w809, "Blue Limit Pressed"=w810, "Right Bumper"=FALSE, "Left Bumper"=FALSE) -> ()  [unwired: 6 in]
            n235 = call "Shooter_Equation.vi"("Right Trigger"=2.0, "Ty"=w804) -> ()  [unwired: 10 in]
            n236 = Wait (ms)(milliseconds to wait=u32 100) -> ()  [unwired: 1 out]
            n237 = call "Drive_Vi.vi"("Middle Thumb"=FALSE, "Z"=0.0, "Y"=0.15, "X"=0.0) -> ()  [unwired: 8 in]
            n238 = call <vilib>:"CTRE_Phoenix_MotorControl_Set.vi"("error in (no error)"=w796, "Output"=0.35, "Control Mode"=w793, "PhoenixMotorControlDevRef"=w795) -> ("error out"=w782:errorcluster, "PhoenixMotorControlDevRef"=w781:T7)  [unwired: 6 in]
            n239 = call <vilib>:"CTRE_Phoenix_MotorControl_Set.vi"("error in (no error)"=w798, "Output"=-0.35, "Control Mode"=w794, "PhoenixMotorControlDevRef"=w797) -> ("error out"=w779:errorcluster, "PhoenixMotorControlDevRef"=w780:T7)  [unwired: 6 in]
          }
          n240 = while {
            tunnel: w721 -> [w774]
            tunnel: w720 -> [w773]
            tunnel: w719 -> [w772]
            tunnel: w718 -> [w771]
            i -> [w769]
            stop <- w768 stop-if-true
            w777 = T11 0 items=["PercentOutput"=0, "Position"=1, "Velocity"=2, "Current"=3, "Follower"=5, "MotionProfile"=6, "MotionMagic"=7, "MotionProfileArc"=10, "Disabled"=15] ("Control Mode")
            w778 = T11 0 items=["PercentOutput"=0, "Position"=1, "Velocity"=2, "Current"=3, "Follower"=5, "MotionProfile"=6, "MotionMagic"=7, "MotionProfileArc"=10, "Disabled"=15] ("Control Mode")
            n241 = call <vilib>:"CTRE_Phoenix_MotorControl_Set.vi"("error in (no error)"=w774, "Output"=0.0, "Control Mode"=w777, "PhoenixMotorControlDevRef"=w773) -> ()  [unwired: 6 in, 2 out]
            n242 = call <vilib>:"CTRE_Phoenix_MotorControl_Set.vi"("error in (no error)"=w771, "Output"=0.0, "Control Mode"=w778, "PhoenixMotorControlDevRef"=w772) -> ()  [unwired: 6 in, 2 out]
            n243 = Greater?(x=w769, y=50) -> (0:w768:bool)
            n244 = Wait (ms)(milliseconds to wait=u32 100) -> ()  [unwired: 1 out]
          }
        }
        frame "2 Ball" {
          # "Pigeon Set"
          n245 = while {
            i -> [w1210]
            stop <- w1211 stop-if-true
            n246 = Wait (ms)(milliseconds to wait=u32 20) -> ()  [unwired: 1 out]
            n247 = Greater?(x=w1210, y=2) -> (0:w1211:bool)
            n248 = call "Drive_Vi.vi"("Middle Thumb"=TRUE, "Z"=0.0, "Y"=0.0, "X"=0.0) -> ()  [unwired: 8 in]
          }
          n249 = call <vilib>:"WPI_SwitchRefNum Registry Get.vi"("refnum name"="Intake Sensor") -> ("error out"=w985:errorcluster, "SwitchDevRef"=w984:T4)  [unwired: 9 in]
          n250 = call <vilib>:"CTRE_Phoenix_MotorControl_RefNumRegistryGet.vi"("refnum name"="Intake") -> ("error out"=w979:errorcluster, "PhoenixMotorControlDevRef"=w978:T7)  [unwired: 9 in]
          n251 = call <vilib>:"CTRE_Phoenix_MotorControl_RefNumRegistryGet.vi"("refnum name"="Intake Actuate") -> ("error out"=w954:errorcluster, "PhoenixMotorControlDevRef"=w953:T7)  [unwired: 9 in]
          n252 = call <vilib>:"CTRE_Phoenix_MotorControl_RefNumRegistryGet.vi"("refnum name"="Reject") -> ("error out"=w981:errorcluster, "PhoenixMotorControlDevRef"=w980:T7)  [unwired: 9 in]
          n253 = call <vilib>:"CTRE_Phoenix_MotorControl_RefNumRegistryGet.vi"("refnum name"="Elevate") -> ("error out"=w983:errorcluster, "PhoenixMotorControlDevRef"=w982:T7)  [unwired: 9 in]
          n254 = call <vilib>:"WPI_SwitchRefNum Registry Get.vi"("refnum name"="Elevate Sensor") -> ("error out"=w987:errorcluster, "SwitchDevRef"=w986:T4)  [unwired: 9 in]
          n255 = call <vilib>:"CTRE_Phoenix_MotorControl_RefNumRegistryGet.vi"("refnum name"="Shoot") -> ("error out"=w967:errorcluster, "PhoenixMotorControlDevRef"=w966:T7)  [unwired: 9 in]
          n256 = while {
            tunnel: w987 -> [w1169]
            tunnel: w986 -> [w1168]
            tunnel: w985 -> [w1167]
            tunnel: w984 -> [w1166]
            tunnel: w983 -> [w1163]
            tunnel: w982 -> [w1162]
            tunnel: w981 -> [w1161]
            tunnel: w980 -> [w1160]
            tunnel: w979 -> [w1159]
            tunnel: w978 -> [w1158]
            tunnel: [w1147] -> w971
            tunnel: [w1146] -> w970
            tunnel: [w1145] -> w969
            tunnel: [w1144] -> w968
            tunnel: w967 -> [w1143]
            tunnel: w966 -> [w1142]
            tunnel: [w1139] -> w965
            tunnel: [w1138] -> w964
            tunnel: w954 -> [w1137]
            tunnel: w953 -> [w1136]
            tunnel: [w1133] -> w952
            tunnel: [w1132] -> w951
            i -> [w1172]
            stop <- w1173 stop-if-true
            w1135 = T11 0 items=["PercentOutput"=0, "Position"=1, "Velocity"=2, "Current"=3, "Follower"=5, "MotionProfile"=6, "MotionMagic"=7, "MotionProfileArc"=10, "Disabled"=15] ("Control Mode")
            w1141 = T11 0 items=["PercentOutput"=0, "Position"=1, "Velocity"=2, "Current"=3, "Follower"=5, "MotionProfile"=6, "MotionMagic"=7, "MotionProfileArc"=10, "Disabled"=15] ("Control Mode")
            w1152 = T11 0 items=["PercentOutput"=0, "Position"=1, "Velocity"=2, "Current"=3, "Follower"=5, "MotionProfile"=6, "MotionMagic"=7, "MotionProfileArc"=10, "Disabled"=15] ("Control Mode")
            w1153 = T11 0 items=["PercentOutput"=0, "Position"=1, "Velocity"=2, "Current"=3, "Follower"=5, "MotionProfile"=6, "MotionMagic"=7, "MotionProfileArc"=10, "Disabled"=15] ("Control Mode")
            w1154 = T11 0 items=["PercentOutput"=0, "Position"=1, "Velocity"=2, "Current"=3, "Follower"=5, "MotionProfile"=6, "MotionMagic"=7, "MotionProfileArc"=10, "Disabled"=15] ("Control Mode")
            n257 = call <vilib>:"CTRE_Phoenix_MotorControl_Set.vi"("error in (no error)"=w1137, "Output"=-0.2, "Control Mode"=w1135, "PhoenixMotorControlDevRef"=w1136) -> ("error out"=w1132:errorcluster, "PhoenixMotorControlDevRef"=w1133:T7)  [unwired: 6 in]
            n258 = global write "AutonBoolean.vi" "Boolean"(TRUE ("Boolean")) -> ()
            n259 = call <vilib>:"WPI_SwitchGetLimitValue.vi"("error in (no error)"=w1167, "SwitchDevRef"=w1166) -> ("Switch Pressed"=w1170:bool)  [unwired: 7 in, 2 out]
            n260 = call <vilib>:"WPI_SwitchGetLimitValue.vi"("error in (no error)"=w1169, "SwitchDevRef"=w1168) -> ("Switch Pressed"=w1171:bool)  [unwired: 7 in, 2 out]
            n261 = Greater?(x=w1172, y=20) -> (0:w1173:bool)
            n262 = Not(x=w1170) -> (.not. x?=w1157:bool)
            "Intake 9" <- w1157
            n263 = Not(x=w1171) -> (.not. x?=w1165:bool)
            "Elevate 9" <- w1165
            n264 = Wait (ms)(milliseconds to wait=u32 100) -> ()  [unwired: 1 out]
            n265 = case shown="True" w1165 {
              tunnel: [0.8 ("Output") w1190] -> w1164
              tunnel: w1157 -> [_ w1187]
              tunnel: [0.75 ("Output") w1189] -> w1156
              tunnel: [-0.1 ("Output") w1188] -> w1155
              tunnel: [FALSE ("Middle Thumb") w1186] -> w1151
              tunnel: [0.0 ("Z") w1185] -> w1150
              tunnel: [0.0 ("Y") w1184] -> w1149
              tunnel: [0.0 ("X") w1183] -> w1148
              frame False {
              }
              frame True {
                n266 = case shown="False" w1187 {
                  tunnel: [1.0 ("Output") 0.0 ("Output")] -> w1190
                  tunnel: [0.0 ("Output") 0.0 ("Output")] -> w1189
                  tunnel: [0.0 ("Output") 0.0 ("Output")] -> w1188
                  tunnel: [FALSE ("Middle Thumb") FALSE ("Middle Thumb")] -> w1186
                  tunnel: [0.0 ("Z") 0.0 ("Z")] -> w1185
                  tunnel: [-0.3 ("Y") 0.0 ("Y")] -> w1184
                  tunnel: [0.0 ("X") 0.0 ("X")] -> w1183
                  frame False {
                  }
                  frame True {
                  }
                }
              }
            }
            n267 = call <vilib>:"CTRE_Phoenix_MotorControl_Set.vi"("error in (no error)"=w1159, "Output"=w1164, "Control Mode"=w1152, "PhoenixMotorControlDevRef"=w1158) -> ("error out"=w1145:errorcluster, "PhoenixMotorControlDevRef"=w1144:T7)  [unwired: 6 in]
            n268 = call <vilib>:"CTRE_Phoenix_MotorControl_Set.vi"("error in (no error)"=w1161, "Output"=w1156, "Control Mode"=w1153, "PhoenixMotorControlDevRef"=w1160) -> ()  [unwired: 6 in, 2 out]
            n269 = call <vilib>:"CTRE_Phoenix_MotorControl_Set.vi"("error in (no error)"=w1163, "Output"=w1155, "Control Mode"=w1154, "PhoenixMotorControlDevRef"=w1162) -> ("error out"=w1147:errorcluster, "PhoenixMotorControlDevRef"=w1146:T7)  [unwired: 6 in]
            n270 = call <vilib>:"CTRE_Phoenix_MotorControl_Set.vi"("error in (no error)"=w1143, "Output"=-0.55, "Control Mode"=w1141, "PhoenixMotorControlDevRef"=w1142) -> ("error out"=w1139:errorcluster, "PhoenixMotorControlDevRef"=w1138:T7)  [unwired: 6 in]
            n271 = call "Drive_Vi.vi"("Middle Thumb"=w1151, "Z"=w1150, "Y"=w1149, "X"=w1148) -> ()  [unwired: 8 in]
          }
          n272 = call <vilib>:"WPI_SwitchRefNum Registry Get.vi"("refnum name"="Orange Limit Switch") -> ("error out"=w973:errorcluster, "SwitchDevRef"=w972:T4)  [unwired: 9 in]
          n273 = call <vilib>:"WPI_SwitchRefNum Registry Get.vi"("refnum name"="Blue Limit Switch") -> ("error out"=w975:errorcluster, "SwitchDevRef"=w974:T4)  [unwired: 9 in]
          n274 = while {
            tunnel: w965 -> [_]
            tunnel: w964 -> [_]
            tunnel: w975 -> [w1128]
            tunnel: w974 -> [w1127]
            tunnel: w973 -> [w1126]
            tunnel: w972 -> [w1125]
            tunnel: w971 -> [w1104]
            tunnel: w970 -> [w1103]
            tunnel: w969 -> [w1099]
            tunnel: w968 -> [w1100]
            tunnel: [w1108] -> w963
            tunnel: [w1107] -> w962
            tunnel: [w1106] -> w961
            tunnel: [w1105] -> w960
            tunnel: [w1104] -> w959
            tunnel: [w1103] -> w958
            tunnel: [w1102] -> w957
            tunnel: [w1101] -> w956
            tunnel: w952 -> [w1094]
            tunnel: w951 -> [w1093]
            i -> [w1114]
            stop <- w1113 stop-if-true
            w1096 = T11 0 items=["PercentOutput"=0, "Position"=1, "Velocity"=2, "Current"=3, "Follower"=5, "MotionProfile"=6, "MotionMagic"=7, "MotionProfileArc"=10, "Disabled"=15] ("Control Mode")
            w1098 = T11 0 items=["PercentOutput"=0, "Position"=1, "Velocity"=2, "Current"=3, "Follower"=5, "MotionProfile"=6, "MotionMagic"=7, "MotionProfileArc"=10, "Disabled"=15] ("Control Mode")
            n275 = call <vilib>:"CTRE_Phoenix_MotorControl_Set.vi"("error in (no error)"=w1093, "Output"=0.0, "Control Mode"=w1096, "PhoenixMotorControlDevRef"=w1094) -> ()  [unwired: 6 in, 2 out]
            n276 = call <vilib>:"WPI_SwitchGetLimitValue.vi"("error in (no error)"=w1126, "SwitchDevRef"=w1125) -> ("error out"=w1105:errorcluster, "Switch Pressed"=w1124:bool, "SwitchDevRef"=w1106:T4)  [unwired: 7 in]
            "Orange Limit Pressed 18" <- w1124
            n277 = call <vilib>:"WPI_SwitchGetLimitValue.vi"("error in (no error)"=w1128, "SwitchDevRef"=w1127) -> ("error out"=w1107:errorcluster, "Switch Pressed"=w1123:bool, "SwitchDevRef"=w1108:T4)  [unwired: 7 in]
            "Blue Limit Pressed 18" <- w1123
            n278 = global write "AutonBoolean.vi" "Boolean"(FALSE ("Boolean")) -> ()
            n279 = call-poly <vilib>:"NT Read Value.vi"("Default Value"=0.0, "Name"="/limelight-drtrain/ty") -> ("Numeric"=w1118:dbl)  [unwired: 8 in, 1 out]
            "Ty 36" <- w1118
            n280 = Greater?(x=w1114, y=5) -> (0:w1113:bool)
            n281 = call "Turret_Aim.vi"("View Button"=FALSE ("Driver Right Thumb"), "Left Trigger"=2.0, "Orange Limit Pressed"=w1123, "Blue Limit Pressed"=w1124, "Right Bumper"=FALSE, "Left Bumper"=FALSE) -> ()  [unwired: 6 in]
            n282 = call "Shooter_Equation.vi"("Right Trigger"=2.0, "Ty"=w1118) -> ()  [unwired: 10 in]
            n283 = Wait (ms)(milliseconds to wait=u32 100) -> ()  [unwired: 1 out]
            n284 = call "Drive_Vi.vi"("Middle Thumb"=FALSE, "Z"=0.0, "Y"=0.15, "X"=0.0) -> ()  [unwired: 8 in]
            n285 = call <vilib>:"CTRE_Phoenix_MotorControl_Set.vi"("error in (no error)"=w1099, "Output"=0.0, "Control Mode"=w1098, "PhoenixMotorControlDevRef"=w1100) -> ("error out"=w1101:errorcluster, "PhoenixMotorControlDevRef"=w1102:T7)  [unwired: 6 in]
          }
          n286 = while {
            tunnel: w962 -> [w1089]
            tunnel: w963 -> [w1088]
            tunnel: w960 -> [w1087]
            tunnel: w959 -> [w1074]
            tunnel: w958 -> [w1073]
            tunnel: w956 -> [w1072]
            tunnel: w957 -> [w1071]
            tunnel: w961 -> [w1062]
            tunnel: [w1061] -> w949
            tunnel: [w1060] -> w950
            tunnel: [w1059] -> w948
            tunnel: [w1058] -> w947
            i -> [w1076]
            stop <- w1075 stop-if-true
            w1069 = T11 0 items=["PercentOutput"=0, "Position"=1, "Velocity"=2, "Current"=3, "Follower"=5, "MotionProfile"=6, "MotionMagic"=7, "MotionProfileArc"=10, "Disabled"=15] ("Control Mode")
            w1070 = T11 0 items=["PercentOutput"=0, "Position"=1, "Velocity"=2, "Current"=3, "Follower"=5, "MotionProfile"=6, "MotionMagic"=7, "MotionProfileArc"=10, "Disabled"=15] ("Control Mode")
            n287 = call <vilib>:"WPI_SwitchGetLimitValue.vi"("error in (no error)"=w1087, "SwitchDevRef"=w1062) -> ("Switch Pressed"=w1086:bool)  [unwired: 7 in, 2 out]
            "Orange Limit Pressed 17" <- w1086
            n288 = call <vilib>:"WPI_SwitchGetLimitValue.vi"("error in (no error)"=w1089, "SwitchDevRef"=w1088) -> ("Switch Pressed"=w1085:bool)  [unwired: 7 in, 2 out]
            "Blue Limit Pressed 17" <- w1085
            n289 = call-poly <vilib>:"NT Read Value.vi"("Default Value"=0.0, "Name"="/limelight-drtrain/ty") -> ("Numeric"=w1080:dbl)  [unwired: 8 in, 1 out]
            "Ty 35" <- w1080
            n290 = Greater?(x=w1076, y=50) -> (0:w1075:bool)
            n291 = call "Shooter_Equation.vi"("Right Trigger"=2.0, "Ty"=w1080) -> ()  [unwired: 10 in]
            n292 = Wait (ms)(milliseconds to wait=u32 100) -> ()  [unwired: 1 out]
            n293 = call "Turret_Aim.vi"("View Button"=FALSE ("Driver Right Thumb"), "Left Trigger"=2.0, "Orange Limit Pressed"=w1085, "Blue Limit Pressed"=w1086, "Right Bumper"=FALSE, "Left Bumper"=FALSE) -> ()  [unwired: 6 in]
            n294 = call "Drive_Vi.vi"("Middle Thumb"=FALSE, "Z"=0.0, "Y"=0.15, "X"=0.0) -> ()  [unwired: 8 in]
            n295 = call <vilib>:"CTRE_Phoenix_MotorControl_Set.vi"("error in (no error)"=w1072, "Output"=0.35, "Control Mode"=w1069, "PhoenixMotorControlDevRef"=w1071) -> ("error out"=w1061:errorcluster, "PhoenixMotorControlDevRef"=w1060:T7)  [unwired: 6 in]
            n296 = call <vilib>:"CTRE_Phoenix_MotorControl_Set.vi"("error in (no error)"=w1074, "Output"=-0.35, "Control Mode"=w1070, "PhoenixMotorControlDevRef"=w1073) -> ("error out"=w1058:errorcluster, "PhoenixMotorControlDevRef"=w1059:T7)  [unwired: 6 in]
          }
          n297 = while {
            tunnel: w947 -> [w1033]
            tunnel: w948 -> [w1032]
            tunnel: w949 -> [w1031]
            tunnel: w950 -> [w1030]
            tunnel: [w1021] -> w945
            tunnel: [w1020] -> w946
            tunnel: [w1019] -> w944
            tunnel: [w1018] -> w943
            i -> [w1035]
            stop <- w1034 stop-if-true
            w1028 = T11 0 items=["PercentOutput"=0, "Position"=1, "Velocity"=2, "Current"=3, "Follower"=5, "MotionProfile"=6, "MotionMagic"=7, "MotionProfileArc"=10, "Disabled"=15] ("Control Mode")
            w1029 = T11 0 items=["PercentOutput"=0, "Position"=1, "Velocity"=2, "Current"=3, "Follower"=5, "MotionProfile"=6, "MotionMagic"=7, "MotionProfileArc"=10, "Disabled"=15] ("Control Mode")
            n298 = call-poly <vilib>:"NT Read Value.vi"("Default Value"=0.0, "Name"="/limelight-drtrain/ty") -> ("Numeric"=w1039:dbl)  [unwired: 8 in, 1 out]
            "Ty 34" <- w1039
            n299 = Greater?(x=w1035, y=10) -> (0:w1034:bool)
            n300 = call "Shooter_Equation.vi"("Right Trigger"=0.0, "Ty"=w1039) -> ()  [unwired: 10 in]
            n301 = Wait (ms)(milliseconds to wait=u32 112) -> ()  [unwired: 1 out]
            n302 = call "Drive_Vi.vi"("Middle Thumb"=FALSE, "Z"=0.35, "Y"=0.0, "X"=0.0) -> ()  [unwired: 8 in]
            n303 = call <vilib>:"CTRE_Phoenix_MotorControl_Set.vi"("error in (no error)"=w1031, "Output"=0.35, "Control Mode"=w1028, "PhoenixMotorControlDevRef"=w1030) -> ("error out"=w1021:errorcluster, "PhoenixMotorControlDevRef"=w1020:T7)  [unwired: 6 in]
            n304 = call <vilib>:"CTRE_Phoenix_MotorControl_Set.vi"("error in (no error)"=w1033, "Output"=-0.35, "Control Mode"=w1029, "PhoenixMotorControlDevRef"=w1032) -> ("error out"=w1018:errorcluster, "PhoenixMotorControlDevRef"=w1019:T7)  [unwired: 6 in]
          }
          n305 = while {
            tunnel: w943 -> [w1009]
            tunnel: w944 -> [w1008]
            tunnel: w945 -> [w1007]
            tunnel: w946 -> [w1006]
            tunnel: [w997] -> w940
            tunnel: [w996] -> w942
            tunnel: [w995] -> w941
            tunnel: [w994] -> w939
            i -> [w1011]
            stop <- w1010 stop-if-true
            w1004 = T11 0 items=["PercentOutput"=0, "Position"=1, "Velocity"=2, "Current"=3, "Follower"=5, "MotionProfile"=6, "MotionMagic"=7, "MotionProfileArc"=10, "Disabled"=15] ("Control Mode")
            w1005 = T11 0 items=["PercentOutput"=0, "Position"=1, "Velocity"=2, "Current"=3, "Follower"=5, "MotionProfile"=6, "MotionMagic"=7, "MotionProfileArc"=10, "Disabled"=15] ("Control Mode")
            n306 = call-poly <vilib>:"NT Read Value.vi"("Default Value"=0.0, "Name"="/limelight-drtrain/ty") -> ("Numeric"=w1015:dbl)  [unwired: 8 in, 1 out]
            "Ty 33" <- w1015
            n307 = Greater?(x=w1011, y=2) -> (0:w1010:bool)
            n308 = call "Shooter_Equation.vi"("Right Trigger"=0.0, "Ty"=w1015) -> ()  [unwired: 10 in]
            n309 = Wait (ms)(milliseconds to wait=u32 20) -> ()  [unwired: 1 out]
            n310 = call "Drive_Vi.vi"("Middle Thumb"=TRUE, "Z"=0.0, "Y"=0.0, "X"=0.0) -> ()  [unwired: 8 in]
            n311 = call <vilib>:"CTRE_Phoenix_MotorControl_Set.vi"("error in (no error)"=w1007, "Output"=0.35, "Control Mode"=w1004, "PhoenixMotorControlDevRef"=w1006) -> ("error out"=w997:errorcluster, "PhoenixMotorControlDevRef"=w996:T7)  [unwired: 6 in]
            n312 = call <vilib>:"CTRE_Phoenix_MotorControl_Set.vi"("error in (no error)"=w1009, "Output"=-0.35, "Control Mode"=w1005, "PhoenixMotorControlDevRef"=w1008) -> ("error out"=w994:errorcluster, "PhoenixMotorControlDevRef"=w995:T7)  [unwired: 6 in]
          }
          n313 = while {
            tunnel: w940 -> [w1053]
            tunnel: w942 -> [w1052]
            tunnel: w941 -> [w1051]
            tunnel: w939 -> [w1050]
            i -> [w1048]
            stop <- w1047 stop-if-true
            w1056 = T11 0 items=["PercentOutput"=0, "Position"=1, "Velocity"=2, "Current"=3, "Follower"=5, "MotionProfile"=6, "MotionMagic"=7, "MotionProfileArc"=10, "Disabled"=15] ("Control Mode")
            w1057 = T11 0 items=["PercentOutput"=0, "Position"=1, "Velocity"=2, "Current"=3, "Follower"=5, "MotionProfile"=6, "MotionMagic"=7, "MotionProfileArc"=10, "Disabled"=15] ("Control Mode")
            n314 = call <vilib>:"CTRE_Phoenix_MotorControl_Set.vi"("error in (no error)"=w1053, "Output"=0.0, "Control Mode"=w1056, "PhoenixMotorControlDevRef"=w1052) -> ()  [unwired: 6 in, 2 out]
            n315 = call <vilib>:"CTRE_Phoenix_MotorControl_Set.vi"("error in (no error)"=w1050, "Output"=0.0, "Control Mode"=w1057, "PhoenixMotorControlDevRef"=w1051) -> ()  [unwired: 6 in, 2 out]
            n316 = call "Drive_Vi.vi"("Middle Thumb"=FALSE, "Z"=0.0, "Y"=0.0, "X"=0.0) -> ()  [unwired: 8 in]
            n317 = Greater?(x=w1048, y=50) -> (0:w1047:bool)
            n318 = Wait (ms)(milliseconds to wait=u32 100) -> ()  [unwired: 1 out]
          }
        }
        frame "Drive Test" {
          # "Get limelight position and shooter started up"
          # "Driving backwards, put arms down and running intake to get ball"
          n319 = call <vilib>:"CTRE_Phoenix_MotorControl_RefNumRegistryGet.vi"("refnum name"="Intake") -> ("error out"=w1214:errorcluster, "PhoenixMotorControlDevRef"=w1216:T7)  [unwired: 9 in]
          n320 = while {
            tunnel: [w1223] -> w1215
            tunnel: w1216 -> [w1223]
            tunnel: [w1222] -> w1213
            tunnel: w1214 -> [w1222]
            i -> [w1229]
            stop <- w1230 stop-if-true
            n321 = Wait (ms)(milliseconds to wait=u32 20) -> ()  [unwired: 1 out]
            n322 = Greater?(x=w1229, y=2) -> (0:w1230:bool)
            n323 = call "Drive_Vi.vi"("Middle Thumb"=TRUE, "Z"=0.0, "Y"=0.0, "X"=0.0) -> ()  [unwired: 8 in]
          }
          n324 = while {
            tunnel: w1215 -> [w1263]
            tunnel: w1213 -> [w1262]
            tunnel: [w1261] -> w1220
            tunnel: [w1260] -> w1219
            i -> [w1270]
            stop <- w1269 stop-if-true
            w1259 = T11 0 items=["PercentOutput"=0, "Position"=1, "Velocity"=2, "Current"=3, "Follower"=5, "MotionProfile"=6, "MotionMagic"=7, "MotionProfileArc"=10, "Disabled"=15] ("Control Mode")
            # "-0.186"
            # "-0.944"
            # ".135"
            n325 = call "Drive_Vi.vi"("Middle Thumb"=FALSE, "Z"=0.0, "Y"=-0.5, "X"=0.0) -> ()  [unwired: 8 in]
            n326 = call <vilib>:"CTRE_Phoenix_MotorControl_Set.vi"("error in (no error)"=w1262, "Output"=0.0, "Control Mode"=w1259, "PhoenixMotorControlDevRef"=w1263) -> ("error out"=w1260:errorcluster, "PhoenixMotorControlDevRef"=w1261:T7)  [unwired: 6 in]
            n327 = Greater?(x=w1270, y=20) -> (0:w1269:bool)
            n328 = Wait (ms)(milliseconds to wait=u32 100) -> ()  [unwired: 1 out]
          }
          n329 = while {
            tunnel: w1220 -> [w1249]
            tunnel: w1219 -> [w1248]
            tunnel: [w1247] -> w1218
            tunnel: [w1246] -> w1217
            i -> [w1256]
            stop <- w1255 stop-if-true
            w1245 = T11 0 items=["PercentOutput"=0, "Position"=1, "Velocity"=2, "Current"=3, "Follower"=5, "MotionProfile"=6, "MotionMagic"=7, "MotionProfileArc"=10, "Disabled"=15] ("Control Mode")
            # "-0.186"
            # "-0.944"
            # ".135"
            n330 = call "Drive_Vi.vi"("Middle Thumb"=FALSE, "Z"=0.0, "Y"=0.15, "X"=0.0) -> ()  [unwired: 8 in]
            n331 = Greater?(x=w1256, y=5) -> (0:w1255:bool)
            n332 = call <vilib>:"CTRE_Phoenix_MotorControl_Set.vi"("error in (no error)"=w1248, "Output"=0.0, "Control Mode"=w1245, "PhoenixMotorControlDevRef"=w1249) -> ("error out"=w1246:errorcluster, "PhoenixMotorControlDevRef"=w1247:T7)  [unwired: 6 in]
            n333 = Wait (ms)(milliseconds to wait=u32 100) -> ()  [unwired: 1 out]
          }
          n334 = while {
            tunnel: w1218 -> [w1235]
            tunnel: w1217 -> [w1234]
            i -> [w1242]
            stop <- w1241 stop-if-true
            w1233 = T11 0 items=["PercentOutput"=0, "Position"=1, "Velocity"=2, "Current"=3, "Follower"=5, "MotionProfile"=6, "MotionMagic"=7, "MotionProfileArc"=10, "Disabled"=15] ("Control Mode")
            # "-0.186"
            # "-0.944"
            # ".135"
            n335 = call "Drive_Vi.vi"("Middle Thumb"=FALSE, "Z"=0.0, "Y"=0.0, "X"=0.0) -> ()  [unwired: 8 in]
            n336 = Greater?(x=w1242, y=20) -> (0:w1241:bool)
            n337 = call <vilib>:"CTRE_Phoenix_MotorControl_Set.vi"("error in (no error)"=w1234, "Output"=0.0, "Control Mode"=w1233, "PhoenixMotorControlDevRef"=w1235) -> ()  [unwired: 6 in, 2 out]
            n338 = Wait (ms)(milliseconds to wait=u32 100) -> ()  [unwired: 1 out]
          }
        }
        frame "4 Ball" {
          # "Pigeon Set"
          n339 = while {
            i -> [w1655]
            stop <- w1656 stop-if-true
            n340 = Wait (ms)(milliseconds to wait=u32 20) -> ()  [unwired: 1 out]
            n341 = Greater?(x=w1655, y=2) -> (0:w1656:bool)
            n342 = call "Drive_Vi.vi"("Middle Thumb"=TRUE, "Z"=0.0, "Y"=0.0, "X"=0.0) -> ()  [unwired: 8 in]
          }
          n343 = call <vilib>:"WPI_SwitchRefNum Registry Get.vi"("refnum name"="Intake Sensor") -> ("error out"=w1332:errorcluster, "SwitchDevRef"=w1331:T4)  [unwired: 9 in]
          n344 = call <vilib>:"CTRE_Phoenix_MotorControl_RefNumRegistryGet.vi"("refnum name"="Intake") -> ("error out"=w1326:errorcluster, "PhoenixMotorControlDevRef"=w1325:T7)  [unwired: 9 in]
          n345 = call <vilib>:"CTRE_Phoenix_MotorControl_RefNumRegistryGet.vi"("refnum name"="Reject") -> ("error out"=w1328:errorcluster, "PhoenixMotorControlDevRef"=w1327:T7)  [unwired: 9 in]
          n346 = call "Limit_Switches.vi"() -> ()  [unwired: 10 in, 2 out]
          n347 = call <vilib>:"CTRE_Phoenix_MotorControl_RefNumRegistryGet.vi"("refnum name"="Elevate") -> ("error out"=w1330:errorcluster, "PhoenixMotorControlDevRef"=w1329:T7)  [unwired: 9 in]
          n348 = call <vilib>:"WPI_SwitchRefNum Registry Get.vi"("refnum name"="Elevate Sensor") -> ("error out"=w1334:errorcluster, "SwitchDevRef"=w1333:T4)  [unwired: 9 in]
          n349 = call <vilib>:"CTRE_Phoenix_MotorControl_RefNumRegistryGet.vi"("refnum name"="Shoot") -> ("error out"=w1314:errorcluster, "PhoenixMotorControlDevRef"=w1313:T7)  [unwired: 9 in]
          n350 = call <vilib>:"CTRE_Phoenix_MotorControl_RefNumRegistryGet.vi"("refnum name"="Intake Actuate") -> ("error out"=w1280:errorcluster, "PhoenixMotorControlDevRef"=w1281:T7)  [unwired: 9 in]
          n351 = while {
            tunnel: w1334 -> [w1614]
            tunnel: w1333 -> [w1613]
            tunnel: w1332 -> [w1612]
            tunnel: w1331 -> [w1611]
            tunnel: w1330 -> [w1608]
            tunnel: w1329 -> [w1607]
            tunnel: w1328 -> [w1606]
            tunnel: w1327 -> [w1605]
            tunnel: w1326 -> [w1604]
            tunnel: w1325 -> [w1603]
            tunnel: [w1592] -> w1318
            tunnel: [w1591] -> w1317
            tunnel: [w1590] -> w1316
            tunnel: [w1589] -> w1315
            tunnel: w1314 -> [w1588]
            tunnel: w1313 -> [w1587]
            tunnel: [w1584] -> w1312
            tunnel: [w1583] -> w1311
            i -> [w1617]
            stop <- w1618 stop-if-true
            w1586 = T11 0 items=["PercentOutput"=0, "Position"=1, "Velocity"=2, "Current"=3, "Follower"=5, "MotionProfile"=6, "MotionMagic"=7, "MotionProfileArc"=10, "Disabled"=15] ("Control Mode")
            w1597 = T11 0 items=["PercentOutput"=0, "Position"=1, "Velocity"=2, "Current"=3, "Follower"=5, "MotionProfile"=6, "MotionMagic"=7, "MotionProfileArc"=10, "Disabled"=15] ("Control Mode")
            w1598 = T11 0 items=["PercentOutput"=0, "Position"=1, "Velocity"=2, "Current"=3, "Follower"=5, "MotionProfile"=6, "MotionMagic"=7, "MotionProfileArc"=10, "Disabled"=15] ("Control Mode")
            w1599 = T11 0 items=["PercentOutput"=0, "Position"=1, "Velocity"=2, "Current"=3, "Follower"=5, "MotionProfile"=6, "MotionMagic"=7, "MotionProfileArc"=10, "Disabled"=15] ("Control Mode")
            n352 = call <vilib>:"WPI_SwitchGetLimitValue.vi"("error in (no error)"=w1612, "SwitchDevRef"=w1611) -> ("Switch Pressed"=w1615:bool)  [unwired: 7 in, 2 out]
            n353 = call <vilib>:"WPI_SwitchGetLimitValue.vi"("error in (no error)"=w1614, "SwitchDevRef"=w1613) -> ("Switch Pressed"=w1616:bool)  [unwired: 7 in, 2 out]
            n354 = Greater?(x=w1617, y=20) -> (0:w1618:bool)
            n355 = Not(x=w1615) -> (.not. x?=w1602:bool)
            "Intake 10" <- w1602
            n356 = Not(x=w1616) -> (.not. x?=w1610:bool)
            "Elevate 10" <- w1610
            n357 = Wait (ms)(milliseconds to wait=u32 100) -> ()  [unwired: 1 out]
            n358 = case shown="True" w1610 {
              tunnel: [0.75 ("Output") w1635] -> w1609
              tunnel: w1602 -> [_ w1632]
              tunnel: [0.75 ("Output") w1634] -> w1601
              tunnel: [-0.1 ("Output") w1633] -> w1600
              tunnel: [FALSE ("Middle Thumb") w1631] -> w1596
              tunnel: [0.0 ("Z") w1630] -> w1595
              tunnel: [0.0 ("Y") w1629] -> w1594
              tunnel: [0.0 ("X") w1628] -> w1593
              frame False {
                (unwired) WPI_SolenoidValue."Reverse" ("Value")
              }
              frame True {
                n359 = case shown="False" w1632 {
                  tunnel: [0.75 ("Output") 0.0 ("Output")] -> w1635
                  tunnel: [0.0 ("Output") 0.0 ("Output")] -> w1634
                  tunnel: [0.0 ("Output") 0.0 ("Output")] -> w1633
                  tunnel: [FALSE ("Middle Thumb") FALSE ("Middle Thumb")] -> w1631
                  tunnel: [0.0 ("Z") 0.0 ("Z")] -> w1630
                  tunnel: [-0.3 ("Y") 0.0 ("Y")] -> w1629
                  tunnel: [0.0 ("X") 0.0 ("X")] -> w1628
                  frame False {
                  }
                  frame True {
                    (unwired) WPI_SolenoidValue."Forward" ("Value")
                  }
                }
              }
            }
            n360 = call <vilib>:"CTRE_Phoenix_MotorControl_Set.vi"("error in (no error)"=w1604, "Output"=w1609, "Control Mode"=w1597, "PhoenixMotorControlDevRef"=w1603) -> ("error out"=w1590:errorcluster, "PhoenixMotorControlDevRef"=w1589:T7)  [unwired: 6 in]
            n361 = call <vilib>:"CTRE_Phoenix_MotorControl_Set.vi"("error in (no error)"=w1606, "Output"=w1601, "Control Mode"=w1598, "PhoenixMotorControlDevRef"=w1605) -> ()  [unwired: 6 in, 2 out]
            n362 = call <vilib>:"CTRE_Phoenix_MotorControl_Set.vi"("error in (no error)"=w1608, "Output"=w1600, "Control Mode"=w1599, "PhoenixMotorControlDevRef"=w1607) -> ("error out"=w1592:errorcluster, "PhoenixMotorControlDevRef"=w1591:T7)  [unwired: 6 in]
            n363 = call <vilib>:"CTRE_Phoenix_MotorControl_Set.vi"("error in (no error)"=w1588, "Output"=-0.55, "Control Mode"=w1586, "PhoenixMotorControlDevRef"=w1587) -> ("error out"=w1584:errorcluster, "PhoenixMotorControlDevRef"=w1583:T7)  [unwired: 6 in]
            n364 = call "Drive_Vi.vi"("Middle Thumb"=w1596, "Z"=w1595, "Y"=w1594, "X"=w1593) -> ()  [unwired: 8 in]
          }
          n365 = while {
            tunnel: w1281 -> [w1362]
            tunnel: w1280 -> [w1361]
            i -> [w1354]
            stop <- w1353 stop-if-true
            n366 = for {
              N: 20 -> [_]
              tunnel: w1362 -> [w1374]
              tunnel: w1361 -> [w1373]
              tunnel: [w1372] -> w1360 mode=indexing
              tunnel: [w1371] -> w1359 mode=indexing
              w1369 = T11 0 items=["PercentOutput"=0, "Position"=1, "Velocity"=2, "Current"=3, "Follower"=5, "MotionProfile"=6, "MotionMagic"=7, "MotionProfileArc"=10, "Disabled"=15] ("Control Mode")
              n367 = call <vilib>:"CTRE_Phoenix_MotorControl_Set.vi"("error in (no error)"=w1373, "Output"=-0.1, "Control Mode"=w1369, "PhoenixMotorControlDevRef"=w1374) -> ("error out"=w1371:errorcluster, "PhoenixMotorControlDevRef"=w1372:T7)  [unwired: 6 in]
              n368 = Wait (ms)(milliseconds to wait=u32 35) -> ()  [unwired: 1 out]
            }
            n369 = for {
              N: 20 -> [_]
              tunnel: w1360 -> [w1367] mode=indexing
              tunnel: w1359 -> [w1366] mode=indexing
              w1364 = T11 0 items=["PercentOutput"=0, "Position"=1, "Velocity"=2, "Current"=3, "Follower"=5, "MotionProfile"=6, "MotionMagic"=7, "MotionProfileArc"=10, "Disabled"=15] ("Control Mode")
              n370 = Wait (ms)(milliseconds to wait=u32 50) -> ()  [unwired: 1 out]
              n371 = call <vilib>:"CTRE_Phoenix_MotorControl_Set.vi"("error in (no error)"=w1366, "Output"=0.0, "Control Mode"=w1364, "PhoenixMotorControlDevRef"=w1367) -> ()  [unwired: 6 in, 2 out]
            }
            n372 = Greater?(x=w1354, y=2) -> (0:w1353:bool)
            n373 = Wait (ms)(milliseconds to wait=u32 20) -> ()  [unwired: 1 out]
          }
          n374 = call <vilib>:"WPI_SwitchRefNum Registry Get.vi"("refnum name"="Orange Limit Switch") -> ("error out"=w1320:errorcluster, "SwitchDevRef"=w1319:T4)  [unwired: 9 in]
          n375 = call <vilib>:"WPI_SwitchRefNum Registry Get.vi"("refnum name"="Blue Limit Switch") -> ("error out"=w1322:errorcluster, "SwitchDevRef"=w1321:T4)  [unwired: 9 in]
          n376 = while {
            tunnel: w1312 -> [_]
            tunnel: w1311 -> [_]
            tunnel: w1322 -> [w1580]
            tunnel: w1321 -> [w1579]
            tunnel: w1320 -> [w1578]
            tunnel: w1319 -> [w1577]
            tunnel: w1318 -> [w1556]
            tunnel: w1317 -> [w1555]
            tunnel: w1316 -> [w1551]
            tunnel: w1315 -> [w1552]
            tunnel: [w1560] -> w1310
            tunnel: [w1559] -> w1309
            tunnel: [w1558] -> w1308
            tunnel: [w1557] -> w1307
            tunnel: [w1556] -> w1306
            tunnel: [w1555] -> w1305
            tunnel: [w1554] -> w1304
            tunnel: [w1553] -> w1303
            i -> [w1566]
            stop <- w1565 stop-if-true
            w1550 = T11 0 items=["PercentOutput"=0, "Position"=1, "Velocity"=2, "Current"=3, "Follower"=5, "MotionProfile"=6, "MotionMagic"=7, "MotionProfileArc"=10, "Disabled"=15] ("Control Mode")
            n377 = call <vilib>:"WPI_SwitchGetLimitValue.vi"("error in (no error)"=w1578, "SwitchDevRef"=w1577) -> ("error out"=w1557:errorcluster, "Switch Pressed"=w1576:bool, "SwitchDevRef"=w1558:T4)  [unwired: 7 in]
            "Orange Limit Pressed 20" <- w1576
            n378 = call <vilib>:"WPI_SwitchGetLimitValue.vi"("error in (no error)"=w1580, "SwitchDevRef"=w1579) -> ("error out"=w1559:errorcluster, "Switch Pressed"=w1575:bool, "SwitchDevRef"=w1560:T4)  [unwired: 7 in]
            "Blue Limit Pressed 20" <- w1575
            n379 = call-poly <vilib>:"NT Read Value.vi"("Default Value"=0.0, "Name"="/limelight-drtrain/ty") -> ("Numeric"=w1570:dbl)  [unwired: 8 in, 1 out]
            "Ty 44" <- w1570
            n380 = Greater?(x=w1566, y=5) -> (0:w1565:bool)
            n381 = call "Turret_Aim.vi"("View Button"=FALSE ("Driver Right Thumb"), "Left Trigger"=2.0, "Orange Limit Pressed"=w1575, "Blue Limit Pressed"=w1576, "Right Bumper"=FALSE, "Left Bumper"=FALSE) -> ()  [unwired: 6 in]
            n382 = call "Shooter_Equation.vi"("Right Trigger"=2.0, "Ty"=w1570) -> ()  [unwired: 10 in]
            n383 = Wait (ms)(milliseconds to wait=u32 100) -> ()  [unwired: 1 out]
            n384 = call "Drive_Vi.vi"("Middle Thumb"=FALSE, "Z"=0.0, "Y"=0.15, "X"=0.0) -> ()  [unwired: 8 in]
            n385 = call <vilib>:"CTRE_Phoenix_MotorControl_Set.vi"("error in (no error)"=w1551, "Output"=0.0, "Control Mode"=w1550, "PhoenixMotorControlDevRef"=w1552) -> ("error out"=w1553:errorcluster, "PhoenixMotorControlDevRef"=w1554:T7)  [unwired: 6 in]
          }
          n386 = while {
            tunnel: w1309 -> [w1546]
            tunnel: w1310 -> [w1545]
            tunnel: w1307 -> [w1544]
            tunnel: w1306 -> [w1531]
            tunnel: w1305 -> [w1530]
            tunnel: w1303 -> [w1529]
            tunnel: w1304 -> [w1528]
            tunnel: w1308 -> [w1519]
            tunnel: [w1518] -> w1302
            tunnel: [w1517] -> w1301
            tunnel: [w1516] -> w1300
            tunnel: [w1515] -> w1299
            i -> [w1533]
            stop <- w1532 stop-if-true
            w1526 = T11 0 items=["PercentOutput"=0, "Position"=1, "Velocity"=2, "Current"=3, "Follower"=5, "MotionProfile"=6, "MotionMagic"=7, "MotionProfileArc"=10, "Disabled"=15] ("Control Mode")
            w1527 = T11 0 items=["PercentOutput"=0, "Position"=1, "Velocity"=2, "Current"=3, "Follower"=5, "MotionProfile"=6, "MotionMagic"=7, "MotionProfileArc"=10, "Disabled"=15] ("Control Mode")
            # "40"
            n387 = call <vilib>:"WPI_SwitchGetLimitValue.vi"("error in (no error)"=w1544, "SwitchDevRef"=w1519) -> ("Switch Pressed"=w1543:bool)  [unwired: 7 in, 2 out]
            "Orange Limit Pressed 19" <- w1543
            n388 = call <vilib>:"WPI_SwitchGetLimitValue.vi"("error in (no error)"=w1546, "SwitchDevRef"=w1545) -> ("Switch Pressed"=w1542:bool)  [unwired: 7 in, 2 out]
            "Blue Limit Pressed 19" <- w1542
            n389 = call-poly <vilib>:"NT Read Value.vi"("Default Value"=0.0, "Name"="/limelight-drtrain/ty") -> ("Numeric"=w1537:dbl)  [unwired: 8 in, 1 out]
            "Ty 43" <- w1537
            n390 = Greater?(x=w1533, y=20) -> (0:w1532:bool)
            n391 = call "Turret_Aim.vi"("View Button"=FALSE ("Driver Right Thumb"), "Left Trigger"=2.0, "Orange Limit Pressed"=w1542, "Blue Limit Pressed"=w1543, "Right Bumper"=FALSE, "Left Bumper"=FALSE) -> ()  [unwired: 6 in]
            n392 = call "Shooter_Equation.vi"("Right Trigger"=2.0, "Ty"=w1537) -> ()  [unwired: 10 in]
            n393 = Wait (ms)(milliseconds to wait=u32 100) -> ()  [unwired: 1 out]
            n394 = call "Drive_Vi.vi"("Middle Thumb"=FALSE, "Z"=0.0, "Y"=0.15, "X"=0.0) -> ()  [unwired: 8 in]
            n395 = call <vilib>:"CTRE_Phoenix_MotorControl_Set.vi"("error in (no error)"=w1529, "Output"=0.35, "Control Mode"=w1526, "PhoenixMotorControlDevRef"=w1528) -> ("error out"=w1518:errorcluster, "PhoenixMotorControlDevRef"=w1517:T7)  [unwired: 6 in]
            n396 = call <vilib>:"CTRE_Phoenix_MotorControl_Set.vi"("error in (no error)"=w1531, "Output"=-0.35, "Control Mode"=w1527, "PhoenixMotorControlDevRef"=w1530) -> ("error out"=w1515:errorcluster, "PhoenixMotorControlDevRef"=w1516:T7)  [unwired: 6 in]
          }
          n397 = while {
            tunnel: w1302 -> [w1510]
            tunnel: w1301 -> [w1509]
            tunnel: w1300 -> [w1508]
            tunnel: w1299 -> [w1507]
            tunnel: [w1498] -> w1279
            tunnel: [w1497] -> w1277
            tunnel: [w1496] -> w1275
            tunnel: [w1495] -> w1273
            i -> [w1505]
            stop <- w1504 stop-if-true
            w1513 = T11 0 items=["PercentOutput"=0, "Position"=1, "Velocity"=2, "Current"=3, "Follower"=5, "MotionProfile"=6, "MotionMagic"=7, "MotionProfileArc"=10, "Disabled"=15] ("Control Mode")
            w1514 = T11 0 items=["PercentOutput"=0, "Position"=1, "Velocity"=2, "Current"=3, "Follower"=5, "MotionProfile"=6, "MotionMagic"=7, "MotionProfileArc"=10, "Disabled"=15] ("Control Mode")
            n398 = call <vilib>:"CTRE_Phoenix_MotorControl_Set.vi"("error in (no error)"=w1510, "Output"=0.0, "Control Mode"=w1513, "PhoenixMotorControlDevRef"=w1509) -> ("error out"=w1497:errorcluster, "PhoenixMotorControlDevRef"=w1498:T7)  [unwired: 6 in]
            n399 = call <vilib>:"CTRE_Phoenix_MotorControl_Set.vi"("error in (no error)"=w1507, "Output"=0.0, "Control Mode"=w1514, "PhoenixMotorControlDevRef"=w1508) -> ("error out"=w1495:errorcluster, "PhoenixMotorControlDevRef"=w1496:T7)  [unwired: 6 in]
            n400 = call "Drive_Vi.vi"("Middle Thumb"=FALSE, "Z"=-0.35, "Y"=0.0, "X"=0.0) -> ()  [unwired: 8 in]
            n401 = Greater?(x=w1505, y=5) -> (0:w1504:bool)
            n402 = Wait (ms)(milliseconds to wait=u32 100) -> ()  [unwired: 1 out]
            n403 = call-poly <vilib>:"NT Read Value.vi"("Default Value"=0.0, "Name"="/limelight-drtrain/ty") -> ("Numeric"=w1500:dbl)  [unwired: 8 in, 1 out]
            "Ty 42" <- w1500
            n404 = call "Shooter_Equation.vi"("Right Trigger"=0.0, "Ty"=w1500) -> ()  [unwired: 10 in]
          }
          n405 = while {
            tunnel: [w1344] -> w1278
            tunnel: w1279 -> [w1344]
            tunnel: [w1343] -> w1276
            tunnel: w1277 -> [w1343]
            tunnel: [w1342] -> w1274
            tunnel: w1275 -> [w1342]
            tunnel: [w1341] -> w1272
            tunnel: w1273 -> [w1341]
            i -> [w1350]
            stop <- w1351 stop-if-true
            n406 = Wait (ms)(milliseconds to wait=u32 20) -> ()  [unwired: 1 out]
            n407 = Greater?(x=w1350, y=5) -> (0:w1351:bool)
            n408 = call "Drive_Vi.vi"("Middle Thumb"=TRUE, "Z"=0.0, "Y"=0.0, "X"=0.0) -> ()  [unwired: 8 in]
          }
          n409 = while {
            tunnel: w1278 -> [w1474]
            tunnel: w1276 -> [w1473]
            tunnel: w1274 -> [w1472]
            tunnel: w1272 -> [w1471]
            tunnel: [w1470] -> w1298
            tunnel: [w1469] -> w1297
            tunnel: [w1468] -> w1296
            tunnel: [w1467] -> w1295
            i -> [w1485]
            stop <- w1484 stop-if-true
            w1489 = T11 0 items=["PercentOutput"=0, "Position"=1, "Velocity"=2, "Current"=3, "Follower"=5, "MotionProfile"=6, "MotionMagic"=7, "MotionProfileArc"=10, "Disabled"=15] ("Control Mode")
            w1490 = T11 0 items=["PercentOutput"=0, "Position"=1, "Velocity"=2, "Current"=3, "Follower"=5, "MotionProfile"=6, "MotionMagic"=7, "MotionProfileArc"=10, "Disabled"=15] ("Control Mode")
            # "-0.186"
            # "-0.944"
            # ".135"
            n410 = call "Drive_Vi.vi"("Middle Thumb"=FALSE, "Z"=0.0, "Y"=-0.8, "X"=0.0) -> ()  [unwired: 8 in]
            n411 = call <vilib>:"CTRE_Phoenix_MotorControl_Set.vi"("error in (no error)"=w1473, "Output"=0.0, "Control Mode"=w1489, "PhoenixMotorControlDevRef"=w1474) -> ("error out"=w1469:errorcluster, "PhoenixMotorControlDevRef"=w1470:T7)  [unwired: 6 in]
            n412 = call <vilib>:"CTRE_Phoenix_MotorControl_Set.vi"("error in (no error)"=w1471, "Output"=0.0, "Control Mode"=w1490, "PhoenixMotorControlDevRef"=w1472) -> ("error out"=w1467:errorcluster, "PhoenixMotorControlDevRef"=w1468:T7)  [unwired: 6 in]
            n413 = Greater?(x=w1485, y=8) -> (0:w1484:bool)
            n414 = Wait (ms)(milliseconds to wait=u32 100) -> ()  [unwired: 1 out]
            n415 = call-poly <vilib>:"NT Read Value.vi"("Default Value"=0.0, "Name"="/limelight-drtrain/ty") -> ("Numeric"=w1476:dbl)  [unwired: 8 in, 1 out]
            "Ty 41" <- w1476
            n416 = call "Shooter_Equation.vi"("Right Trigger"=0.0, "Ty"=w1476) -> ()  [unwired: 10 in]
          }
          n417 = while {
            tunnel: w1298 -> [w1458]
            tunnel: w1297 -> [w1457]
            tunnel: w1296 -> [w1456]
            tunnel: w1295 -> [w1455]
            tunnel: [w1450] -> w1294
            tunnel: [w1449] -> w1293
            tunnel: [w1448] -> w1292
            tunnel: [w1447] -> w1291
            i -> [w1452]
            stop <- w1451 stop-if-true
            w1465 = T11 0 items=["PercentOutput"=0, "Position"=1, "Velocity"=2, "Current"=3, "Follower"=5, "MotionProfile"=6, "MotionMagic"=7, "MotionProfileArc"=10, "Disabled"=15] ("Control Mode")
            w1466 = T11 0 items=["PercentOutput"=0, "Position"=1, "Velocity"=2, "Current"=3, "Follower"=5, "MotionProfile"=6, "MotionMagic"=7, "MotionProfileArc"=10, "Disabled"=15] ("Control Mode")
            # "-0.186"
            # "-0.944"
            # ".135"
            n418 = call <vilib>:"CTRE_Phoenix_MotorControl_Set.vi"("error in (no error)"=w1457, "Output"=0.0, "Control Mode"=w1465, "PhoenixMotorControlDevRef"=w1458) -> ("error out"=w1449:errorcluster, "PhoenixMotorControlDevRef"=w1450:T7)  [unwired: 6 in]
            n419 = call <vilib>:"CTRE_Phoenix_MotorControl_Set.vi"("error in (no error)"=w1455, "Output"=0.0, "Control Mode"=w1466, "PhoenixMotorControlDevRef"=w1456) -> ("error out"=w1447:errorcluster, "PhoenixMotorControlDevRef"=w1448:T7)  [unwired: 6 in]
            n420 = call "Drive_Vi.vi"("Middle Thumb"=FALSE, "Z"=0.0, "Y"=0.0, "X"=0.0) -> ()  [unwired: 8 in]
            n421 = Greater?(x=w1452, y=5) -> (0:w1451:bool)
            n422 = call-poly <vilib>:"NT Read Value.vi"("Default Value"=0.0, "Name"="/limelight-drtrain/ty") -> ("Numeric"=w1460:dbl)  [unwired: 8 in, 1 out]
            "Ty 40" <- w1460
            n423 = Wait (ms)(milliseconds to wait=u32 100) -> ()  [unwired: 1 out]
            n424 = call "Shooter_Equation.vi"("Right Trigger"=0.0, "Ty"=w1460) -> ()  [unwired: 10 in]
          }
          n425 = while {
            tunnel: w1294 -> [w1430]
            tunnel: w1293 -> [w1429]
            tunnel: w1292 -> [w1428]
            tunnel: w1291 -> [w1427]
            tunnel: [w1422] -> w1290
            tunnel: [w1421] -> w1289
            tunnel: [w1420] -> w1288
            tunnel: [w1419] -> w1287
            i -> [w1424]
            stop <- w1423 stop-if-true
            w1441 = T11 0 items=["PercentOutput"=0, "Position"=1, "Velocity"=2, "Current"=3, "Follower"=5, "MotionProfile"=6, "MotionMagic"=7, "MotionProfileArc"=10, "Disabled"=15] ("Control Mode")
            w1442 = T11 0 items=["PercentOutput"=0, "Position"=1, "Velocity"=2, "Current"=3, "Follower"=5, "MotionProfile"=6, "MotionMagic"=7, "MotionProfileArc"=10, "Disabled"=15] ("Control Mode")
            # "-0.186"
            # "-0.944"
            # ".135"
            n426 = call "Drive_Vi.vi"("Middle Thumb"=FALSE, "Z"=0.0, "Y"=0.0, "X"=0.0) -> ()  [unwired: 8 in]
            n427 = call <vilib>:"CTRE_Phoenix_MotorControl_Set.vi"("error in (no error)"=w1429, "Output"=0.75, "Control Mode"=w1441, "PhoenixMotorControlDevRef"=w1430) -> ("error out"=w1421:errorcluster, "PhoenixMotorControlDevRef"=w1422:T7)  [unwired: 6 in]
            n428 = call <vilib>:"CTRE_Phoenix_MotorControl_Set.vi"("error in (no error)"=w1427, "Output"=-0.1, "Control Mode"=w1442, "PhoenixMotorControlDevRef"=w1428) -> ("error out"=w1419:errorcluster, "PhoenixMotorControlDevRef"=w1420:T7)  [unwired: 6 in]
            n429 = Greater?(x=w1424, y=20) -> (0:w1423:bool)
            n430 = Wait (ms)(milliseconds to wait=u32 100) -> ()  [unwired: 1 out]
            n431 = call-poly <vilib>:"NT Read Value.vi"("Default Value"=0.0, "Name"="/limelight-drtrain/ty") -> ("Numeric"=w1432:dbl)  [unwired: 8 in, 1 out]
            "Ty 39" <- w1432
            n432 = call "Shooter_Equation.vi"("Right Trigger"=0.0, "Ty"=w1432) -> ()  [unwired: 10 in]
          }
          n433 = while {
            tunnel: w1290 -> [w1406]
            tunnel: [w1399] -> _
            tunnel: w1288 -> [w1405]
            tunnel: w1287 -> [w1404]
            tunnel: w1289 -> [w1399]
            tunnel: [w1398] -> w1286
            tunnel: [w1397] -> w1285
            tunnel: [w1396] -> w1284
            tunnel: [w1395] -> w1283
            i -> [w1401]
            stop <- w1400 stop-if-true
            w1417 = T11 0 items=["PercentOutput"=0, "Position"=1, "Velocity"=2, "Current"=3, "Follower"=5, "MotionProfile"=6, "MotionMagic"=7, "MotionProfileArc"=10, "Disabled"=15] ("Control Mode")
            w1418 = T11 0 items=["PercentOutput"=0, "Position"=1, "Velocity"=2, "Current"=3, "Follower"=5, "MotionProfile"=6, "MotionMagic"=7, "MotionProfileArc"=10, "Disabled"=15] ("Control Mode")
            # "-0.186"
            # "-0.944"
            # ".135"
            n434 = call "Drive_Vi.vi"("Middle Thumb"=FALSE, "Z"=0.0, "Y"=0.0, "X"=0.0) -> ()  [unwired: 8 in]
            n435 = call <vilib>:"CTRE_Phoenix_MotorControl_Set.vi"("error in (no error)"=w1399, "Output"=0.0, "Control Mode"=w1417, "PhoenixMotorControlDevRef"=w1406) -> ("error out"=w1395:errorcluster, "PhoenixMotorControlDevRef"=w1396:T7)  [unwired: 6 in]
            n436 = call <vilib>:"CTRE_Phoenix_MotorControl_Set.vi"("error in (no error)"=w1404, "Output"=0.0, "Control Mode"=w1418, "PhoenixMotorControlDevRef"=w1405) -> ("error out"=w1398:errorcluster, "PhoenixMotorControlDevRef"=w1397:T7)  [unwired: 6 in]
            n437 = Greater?(x=w1401, y=10) -> (0:w1400:bool)
            n438 = Wait (ms)(milliseconds to wait=u32 100) -> ()  [unwired: 1 out]
            n439 = call-poly <vilib>:"NT Read Value.vi"("Default Value"=0.0, "Name"="/limelight-drtrain/ty") -> ("Numeric"=w1408:dbl)  [unwired: 8 in, 1 out]
            "Ty 38" <- w1408
            n440 = call "Shooter_Equation.vi"("Right Trigger"=0.0, "Ty"=w1408) -> ()  [unwired: 10 in]
          }
          n441 = while {
            tunnel: w1284 -> [w1382]
            tunnel: [w1375] -> _
            tunnel: w1285 -> [w1381]
            tunnel: w1286 -> [w1380]
            tunnel: w1283 -> [w1375]
            i -> [w1377]
            stop <- w1376 stop-if-true
            w1393 = T11 0 items=["PercentOutput"=0, "Position"=1, "Velocity"=2, "Current"=3, "Follower"=5, "MotionProfile"=6, "MotionMagic"=7, "MotionProfileArc"=10, "Disabled"=15] ("Control Mode")
            w1394 = T11 0 items=["PercentOutput"=0, "Position"=1, "Velocity"=2, "Current"=3, "Follower"=5, "MotionProfile"=6, "MotionMagic"=7, "MotionProfileArc"=10, "Disabled"=15] ("Control Mode")
            # "-0.186"
            # "-0.944"
            # ".135"
            n442 = call "Drive_Vi.vi"("Middle Thumb"=FALSE, "Z"=0.0, "Y"=0.0, "X"=0.0) -> ()  [unwired: 8 in]
            n443 = call <vilib>:"CTRE_Phoenix_MotorControl_Set.vi"("error in (no error)"=w1375, "Output"=0.0, "Control Mode"=w1393, "PhoenixMotorControlDevRef"=w1382) -> ()  [unwired: 6 in, 2 out]
            n444 = call <vilib>:"CTRE_Phoenix_MotorControl_Set.vi"("error in (no error)"=w1380, "Output"=0.0, "Control Mode"=w1394, "PhoenixMotorControlDevRef"=w1381) -> ()  [unwired: 6 in, 2 out]
            n445 = Greater?(x=w1377, y=20) -> (0:w1376:bool)
            n446 = Wait (ms)(milliseconds to wait=u32 100) -> ()  [unwired: 1 out]
            n447 = call-poly <vilib>:"NT Read Value.vi"("Default Value"=0.0, "Name"="/limelight-drtrain/ty") -> ("Numeric"=w1384:dbl)  [unwired: 8 in, 1 out]
            "Ty 37" <- w1384
            n448 = call "Shooter_Equation.vi"("Right Trigger"=0.0, "Ty"=w1384) -> ()  [unwired: 10 in]
          }
        }
        frame "4 Ball Pos 3" {
          # "Pigeon Set"
          n449 = while {
            i -> [w2073]
            stop <- w2074 stop-if-true
            n450 = Wait (ms)(milliseconds to wait=u32 20) -> ()  [unwired: 1 out]
            n451 = Greater?(x=w2073, y=2) -> (0:w2074:bool)
            n452 = call "Drive_Vi.vi"("Middle Thumb"=TRUE, "Z"=0.0, "Y"=0.0, "X"=0.0) -> ()  [unwired: 8 in]
          }
          n453 = call <vilib>:"WPI_SwitchRefNum Registry Get.vi"("refnum name"="Intake Sensor") -> ("error out"=w1726:errorcluster, "SwitchDevRef"=w1725:T4)  [unwired: 9 in]
          n454 = call <vilib>:"CTRE_Phoenix_MotorControl_RefNumRegistryGet.vi"("refnum name"="Intake") -> ("error out"=w1720:errorcluster, "PhoenixMotorControlDevRef"=w1719:T7)  [unwired: 9 in]
          n455 = call <vilib>:"CTRE_Phoenix_MotorControl_RefNumRegistryGet.vi"("refnum name"="Reject") -> ("error out"=w1722:errorcluster, "PhoenixMotorControlDevRef"=w1721:T7)  [unwired: 9 in]
          n456 = call "Limit_Switches.vi"() -> ()  [unwired: 10 in, 2 out]
          n457 = call <vilib>:"CTRE_Phoenix_MotorControl_RefNumRegistryGet.vi"("refnum name"="Elevate") -> ("error out"=w1724:errorcluster, "PhoenixMotorControlDevRef"=w1723:T7)  [unwired: 9 in]
          n458 = call <vilib>:"WPI_SwitchRefNum Registry Get.vi"("refnum name"="Elevate Sensor") -> ("error out"=w1728:errorcluster, "SwitchDevRef"=w1727:T4)  [unwired: 9 in]
          n459 = call <vilib>:"CTRE_Phoenix_MotorControl_RefNumRegistryGet.vi"("refnum name"="Shoot") -> ("error out"=w1708:errorcluster, "PhoenixMotorControlDevRef"=w1707:T7)  [unwired: 9 in]
          n460 = call <vilib>:"CTRE_Phoenix_MotorControl_RefNumRegistryGet.vi"("refnum name"="Intake Actuate") -> ("error out"=w1678:errorcluster, "PhoenixMotorControlDevRef"=w1679:T7)  [unwired: 9 in]
          n461 = while {
            tunnel: w1728 -> [w2032]
            tunnel: w1727 -> [w2031]
            tunnel: w1726 -> [w2030]
            tunnel: w1725 -> [w2029]
            tunnel: w1724 -> [w2026]
            tunnel: w1723 -> [w2025]
            tunnel: w1722 -> [w2024]
            tunnel: w1721 -> [w2023]
            tunnel: w1720 -> [w2022]
            tunnel: w1719 -> [w2021]
            tunnel: [w2010] -> w1712
            tunnel: [w2009] -> w1711
            tunnel: [w2008] -> w1710
            tunnel: [w2007] -> w1709
            tunnel: w1708 -> [w2006]
            tunnel: w1707 -> [w2005]
            tunnel: [w2002] -> w1706
            tunnel: [w2001] -> w1705
            i -> [w2035]
            stop <- w2036 stop-if-true
            w2004 = T11 0 items=["PercentOutput"=0, "Position"=1, "Velocity"=2, "Current"=3, "Follower"=5, "MotionProfile"=6, "MotionMagic"=7, "MotionProfileArc"=10, "Disabled"=15] ("Control Mode")
            w2015 = T11 0 items=["PercentOutput"=0, "Position"=1, "Velocity"=2, "Current"=3, "Follower"=5, "MotionProfile"=6, "MotionMagic"=7, "MotionProfileArc"=10, "Disabled"=15] ("Control Mode")
            w2016 = T11 0 items=["PercentOutput"=0, "Position"=1, "Velocity"=2, "Current"=3, "Follower"=5, "MotionProfile"=6, "MotionMagic"=7, "MotionProfileArc"=10, "Disabled"=15] ("Control Mode")
            w2017 = T11 0 items=["PercentOutput"=0, "Position"=1, "Velocity"=2, "Current"=3, "Follower"=5, "MotionProfile"=6, "MotionMagic"=7, "MotionProfileArc"=10, "Disabled"=15] ("Control Mode")
            n462 = call <vilib>:"WPI_SwitchGetLimitValue.vi"("error in (no error)"=w2030, "SwitchDevRef"=w2029) -> ("Switch Pressed"=w2033:bool)  [unwired: 7 in, 2 out]
            n463 = call <vilib>:"WPI_SwitchGetLimitValue.vi"("error in (no error)"=w2032, "SwitchDevRef"=w2031) -> ("Switch Pressed"=w2034:bool)  [unwired: 7 in, 2 out]
            n464 = Greater?(x=w2035, y=20) -> (0:w2036:bool)
            n465 = Not(x=w2033) -> (.not. x?=w2020:bool)
            "Intake 11" <- w2020
            n466 = Not(x=w2034) -> (.not. x?=w2028:bool)
            "Elevate 11" <- w2028
            n467 = Wait (ms)(milliseconds to wait=u32 100) -> ()  [unwired: 1 out]
            n468 = case shown="True" w2028 {
              tunnel: [0.75 ("Output") w2053] -> w2027
              tunnel: w2020 -> [_ w2050]
              tunnel: [0.75 ("Output") w2052] -> w2019
              tunnel: [-0.1 ("Output") w2051] -> w2018
              tunnel: [FALSE ("Middle Thumb") w2049] -> w2014
              tunnel: [0.0 ("Z") w2048] -> w2013
              tunnel: [0.0 ("Y") w2047] -> w2012
              tunnel: [0.0 ("X") w2046] -> w2011
              frame False {
                (unwired) WPI_SolenoidValue."Reverse" ("Value")
              }
              frame True {
                n469 = case shown="True" w2050 {
                  tunnel: [0.75 ("Output") 0.0 ("Output")] -> w2053
                  tunnel: [0.0 ("Output") 0.0 ("Output")] -> w2052
                  tunnel: [0.0 ("Output") 0.0 ("Output")] -> w2051
                  tunnel: [FALSE ("Middle Thumb") FALSE ("Middle Thumb")] -> w2049
                  tunnel: [0.0 ("Z") 0.0 ("Z")] -> w2048
                  tunnel: [-0.3 ("Y") 0.0 ("Y")] -> w2047
                  tunnel: [0.0 ("X") 0.0 ("X")] -> w2046
                  frame False {
                  }
                  frame True {
                  }
                }
              }
            }
            n470 = call <vilib>:"CTRE_Phoenix_MotorControl_Set.vi"("error in (no error)"=w2022, "Output"=w2027, "Control Mode"=w2015, "PhoenixMotorControlDevRef"=w2021) -> ("error out"=w2008:errorcluster, "PhoenixMotorControlDevRef"=w2007:T7)  [unwired: 6 in]
            n471 = call <vilib>:"CTRE_Phoenix_MotorControl_Set.vi"("error in (no error)"=w2024, "Output"=w2019, "Control Mode"=w2016, "PhoenixMotorControlDevRef"=w2023) -> ()  [unwired: 6 in, 2 out]
            n472 = call <vilib>:"CTRE_Phoenix_MotorControl_Set.vi"("error in (no error)"=w2026, "Output"=w2018, "Control Mode"=w2017, "PhoenixMotorControlDevRef"=w2025) -> ("error out"=w2010:errorcluster, "PhoenixMotorControlDevRef"=w2009:T7)  [unwired: 6 in]
            n473 = call <vilib>:"CTRE_Phoenix_MotorControl_Set.vi"("error in (no error)"=w2006, "Output"=-0.55, "Control Mode"=w2004, "PhoenixMotorControlDevRef"=w2005) -> ("error out"=w2002:errorcluster, "PhoenixMotorControlDevRef"=w2001:T7)  [unwired: 6 in]
            n474 = call "Drive_Vi.vi"("Middle Thumb"=w2014, "Z"=w2013, "Y"=w2012, "X"=w2011) -> ()  [unwired: 8 in]
          }
          n475 = while {
            tunnel: w1679 -> [w1768]
            tunnel: w1678 -> [w1767]
            i -> [w1760]
            stop <- w1759 stop-if-true
            n476 = for {
              N: 20 -> [_]
              tunnel: w1768 -> [w1780]
              tunnel: w1767 -> [w1779]
              tunnel: [w1778] -> w1766 mode=indexing
              tunnel: [w1777] -> w1765 mode=indexing
              w1775 = T11 0 items=["PercentOutput"=0, "Position"=1, "Velocity"=2, "Current"=3, "Follower"=5, "MotionProfile"=6, "MotionMagic"=7, "MotionProfileArc"=10, "Disabled"=15] ("Control Mode")
              n477 = call <vilib>:"CTRE_Phoenix_MotorControl_Set.vi"("error in (no error)"=w1779, "Output"=-0.1, "Control Mode"=w1775, "PhoenixMotorControlDevRef"=w1780) -> ("error out"=w1777:errorcluster, "PhoenixMotorControlDevRef"=w1778:T7)  [unwired: 6 in]
              n478 = Wait (ms)(milliseconds to wait=u32 35) -> ()  [unwired: 1 out]
            }
            n479 = for {
              N: 20 -> [_]
              tunnel: w1766 -> [w1773] mode=indexing
              tunnel: w1765 -> [w1772] mode=indexing
              w1770 = T11 0 items=["PercentOutput"=0, "Position"=1, "Velocity"=2, "Current"=3, "Follower"=5, "MotionProfile"=6, "MotionMagic"=7, "MotionProfileArc"=10, "Disabled"=15] ("Control Mode")
              n480 = Wait (ms)(milliseconds to wait=u32 50) -> ()  [unwired: 1 out]
              n481 = call <vilib>:"CTRE_Phoenix_MotorControl_Set.vi"("error in (no error)"=w1772, "Output"=0.0, "Control Mode"=w1770, "PhoenixMotorControlDevRef"=w1773) -> ()  [unwired: 6 in, 2 out]
            }
            n482 = Greater?(x=w1760, y=2) -> (0:w1759:bool)
            n483 = Wait (ms)(milliseconds to wait=u32 20) -> ()  [unwired: 1 out]
          }
          n484 = call <vilib>:"WPI_SwitchRefNum Registry Get.vi"("refnum name"="Orange Limit Switch") -> ("error out"=w1714:errorcluster, "SwitchDevRef"=w1713:T4)  [unwired: 9 in]
          n485 = call <vilib>:"WPI_SwitchRefNum Registry Get.vi"("refnum name"="Blue Limit Switch") -> ("error out"=w1716:errorcluster, "SwitchDevRef"=w1715:T4)  [unwired: 9 in]
          n486 = while {
            tunnel: w1706 -> [_]
            tunnel: w1705 -> [_]
            tunnel: w1716 -> [w1998]
            tunnel: w1715 -> [w1997]
            tunnel: w1714 -> [w1996]
            tunnel: w1713 -> [w1995]
            tunnel: w1712 -> [w1974]
            tunnel: w1711 -> [w1973]
            tunnel: w1710 -> [w1969]
            tunnel: w1709 -> [w1970]
            tunnel: [w1978] -> w1704
            tunnel: [w1977] -> w1703
            tunnel: [w1976] -> w1702
            tunnel: [w1975] -> w1701
            tunnel: [w1974] -> w1700
            tunnel: [w1973] -> w1699
            tunnel: [w1972] -> w1698
            tunnel: [w1971] -> w1697
            i -> [w1984]
            stop <- w1983 stop-if-true
            w1968 = T11 0 items=["PercentOutput"=0, "Position"=1, "Velocity"=2, "Current"=3, "Follower"=5, "MotionProfile"=6, "MotionMagic"=7, "MotionProfileArc"=10, "Disabled"=15] ("Control Mode")
            n487 = call <vilib>:"WPI_SwitchGetLimitValue.vi"("error in (no error)"=w1996, "SwitchDevRef"=w1995) -> ("error out"=w1975:errorcluster, "Switch Pressed"=w1994:bool, "SwitchDevRef"=w1976:T4)  [unwired: 7 in]
            "Orange Limit Pressed 22" <- w1994
            n488 = call <vilib>:"WPI_SwitchGetLimitValue.vi"("error in (no error)"=w1998, "SwitchDevRef"=w1997) -> ("error out"=w1977:errorcluster, "Switch Pressed"=w1993:bool, "SwitchDevRef"=w1978:T4)  [unwired: 7 in]
            "Blue Limit Pressed 22" <- w1993
            n489 = call-poly <vilib>:"NT Read Value.vi"("Default Value"=0.0, "Name"="/limelight-drtrain/ty") -> ("Numeric"=w1988:dbl)  [unwired: 8 in, 1 out]
            "Ty 52" <- w1988
            n490 = Greater?(x=w1984, y=5) -> (0:w1983:bool)
            n491 = call "Turret_Aim.vi"("View Button"=FALSE ("Driver Right Thumb"), "Left Trigger"=2.0, "Orange Limit Pressed"=w1993, "Blue Limit Pressed"=w1994, "Right Bumper"=FALSE, "Left Bumper"=FALSE) -> ()  [unwired: 6 in]
            n492 = call "Shooter_Equation.vi"("Right Trigger"=2.0, "Ty"=w1988) -> ()  [unwired: 10 in]
            n493 = Wait (ms)(milliseconds to wait=u32 100) -> ()  [unwired: 1 out]
            n494 = call "Drive_Vi.vi"("Middle Thumb"=FALSE, "Z"=0.0, "Y"=0.15, "X"=0.0) -> ()  [unwired: 8 in]
            n495 = call <vilib>:"CTRE_Phoenix_MotorControl_Set.vi"("error in (no error)"=w1969, "Output"=0.0, "Control Mode"=w1968, "PhoenixMotorControlDevRef"=w1970) -> ("error out"=w1971:errorcluster, "PhoenixMotorControlDevRef"=w1972:T7)  [unwired: 6 in]
          }
          n496 = while {
            tunnel: w1703 -> [w1964]
            tunnel: w1704 -> [w1963]
            tunnel: w1701 -> [w1962]
            tunnel: w1700 -> [w1951]
            tunnel: w1699 -> [w1950]
            tunnel: w1697 -> [w1949]
            tunnel: w1698 -> [w1948]
            tunnel: w1702 -> [w1939]
            tunnel: [w1938] -> w1696
            tunnel: [w1937] -> w1695
            tunnel: [w1936] -> w1694
            tunnel: [w1935] -> w1693
            tunnel: [w1934] -> w1661
            tunnel: [w1933] -> w1660
            i -> [w1953]
            stop <- w1952 stop-if-true
            w1946 = T11 0 items=["PercentOutput"=0, "Position"=1, "Velocity"=2, "Current"=3, "Follower"=5, "MotionProfile"=6, "MotionMagic"=7, "MotionProfileArc"=10, "Disabled"=15] ("Control Mode")
            w1947 = T11 0 items=["PercentOutput"=0, "Position"=1, "Velocity"=2, "Current"=3, "Follower"=5, "MotionProfile"=6, "MotionMagic"=7, "MotionProfileArc"=10, "Disabled"=15] ("Control Mode")
            # "40"
            n497 = call <vilib>:"WPI_SwitchGetLimitValue.vi"("error in (no error)"=w1962, "SwitchDevRef"=w1939) -> ("Switch Pressed"=w1934:bool)  [unwired: 7 in, 2 out]
            "Orange Limit Pressed 21" <- w1934
            n498 = call <vilib>:"WPI_SwitchGetLimitValue.vi"("error in (no error)"=w1964, "SwitchDevRef"=w1963) -> ("Switch Pressed"=w1933:bool)  [unwired: 7 in, 2 out]
            "Blue Limit Pressed 21" <- w1933
            n499 = call-poly <vilib>:"NT Read Value.vi"("Default Value"=0.0, "Name"="/limelight-drtrain/ty") -> ("Numeric"=w1957:dbl)  [unwired: 8 in, 1 out]
            "Ty 51" <- w1957
            n500 = Greater?(x=w1953, y=20) -> (0:w1952:bool)
            n501 = call "Turret_Aim.vi"("View Button"=FALSE ("Driver Right Thumb"), "Left Trigger"=2.0, "Orange Limit Pressed"=w1933, "Blue Limit Pressed"=w1934, "Right Bumper"=FALSE, "Left Bumper"=FALSE) -> ()  [unwired: 6 in]
            n502 = call "Shooter_Equation.vi"("Right Trigger"=2.0, "Ty"=w1957) -> ()  [unwired: 10 in]
            n503 = Wait (ms)(milliseconds to wait=u32 100) -> ()  [unwired: 1 out]
            n504 = call "Drive_Vi.vi"("Middle Thumb"=FALSE, "Z"=0.0, "Y"=0.15, "X"=0.0) -> ()  [unwired: 8 in]
            n505 = call <vilib>:"CTRE_Phoenix_MotorControl_Set.vi"("error in (no error)"=w1949, "Output"=0.35, "Control Mode"=w1946, "PhoenixMotorControlDevRef"=w1948) -> ("error out"=w1938:errorcluster, "PhoenixMotorControlDevRef"=w1937:T7)  [unwired: 6 in]
            n506 = call <vilib>:"CTRE_Phoenix_MotorControl_Set.vi"("error in (no error)"=w1951, "Output"=-0.35, "Control Mode"=w1947, "PhoenixMotorControlDevRef"=w1950) -> ("error out"=w1935:errorcluster, "PhoenixMotorControlDevRef"=w1936:T7)  [unwired: 6 in]
          }
          n507 = while {
            tunnel: w1696 -> [w1928]
            tunnel: w1695 -> [w1927]
            tunnel: w1694 -> [w1926]
            tunnel: w1693 -> [w1925]
            tunnel: [w1916] -> w1677
            tunnel: [w1915] -> w1675
            tunnel: [w1914] -> w1673
            tunnel: [w1913] -> w1671
            i -> [w1923]
            stop <- w1922 stop-if-true
            w1931 = T11 0 items=["PercentOutput"=0, "Position"=1, "Velocity"=2, "Current"=3, "Follower"=5, "MotionProfile"=6, "MotionMagic"=7, "MotionProfileArc"=10, "Disabled"=15] ("Control Mode")
            w1932 = T11 0 items=["PercentOutput"=0, "Position"=1, "Velocity"=2, "Current"=3, "Follower"=5, "MotionProfile"=6, "MotionMagic"=7, "MotionProfileArc"=10, "Disabled"=15] ("Control Mode")
            n508 = call <vilib>:"CTRE_Phoenix_MotorControl_Set.vi"("error in (no error)"=w1928, "Output"=0.0, "Control Mode"=w1931, "PhoenixMotorControlDevRef"=w1927) -> ("error out"=w1915:errorcluster, "PhoenixMotorControlDevRef"=w1916:T7)  [unwired: 6 in]
            n509 = call <vilib>:"CTRE_Phoenix_MotorControl_Set.vi"("error in (no error)"=w1925, "Output"=0.0, "Control Mode"=w1932, "PhoenixMotorControlDevRef"=w1926) -> ("error out"=w1913:errorcluster, "PhoenixMotorControlDevRef"=w1914:T7)  [unwired: 6 in]
            n510 = call "Drive_Vi.vi"("Middle Thumb"=FALSE, "Z"=0.22, "Y"=0.0, "X"=0.0) -> ()  [unwired: 8 in]
            n511 = Greater?(x=w1923, y=4) -> (0:w1922:bool)
            n512 = Wait (ms)(milliseconds to wait=u32 100) -> ()  [unwired: 1 out]
            n513 = call-poly <vilib>:"NT Read Value.vi"("Default Value"=0.0, "Name"="/limelight-drtrain/ty") -> ("Numeric"=w1918:dbl)  [unwired: 8 in, 1 out]
            "Ty 50" <- w1918
            n514 = call "Shooter_Equation.vi"("Right Trigger"=0.0, "Ty"=w1918) -> ()  [unwired: 10 in]
          }
          n515 = while {
            tunnel: [w1750] -> w1676
            tunnel: w1677 -> [w1750]
            tunnel: [w1749] -> w1674
            tunnel: w1675 -> [w1749]
            tunnel: [w1748] -> w1672
            tunnel: w1673 -> [w1748]
            tunnel: [w1747] -> w1670
            tunnel: w1671 -> [w1747]
            i -> [w1756]
            stop <- w1757 stop-if-true
            n516 = Wait (ms)(milliseconds to wait=u32 20) -> ()  [unwired: 1 out]
            n517 = Greater?(x=w1756, y=5) -> (0:w1757:bool)
            n518 = call "Drive_Vi.vi"("Middle Thumb"=TRUE, "Z"=0.0, "Y"=0.0, "X"=0.0) -> ()  [unwired: 8 in]
          }
          n519 = while {
            tunnel: w1676 -> [w1892]
            tunnel: w1674 -> [w1891]
            tunnel: w1672 -> [w1890]
            tunnel: w1670 -> [w1889]
            tunnel: [w1888] -> w1692
            tunnel: [w1887] -> w1691
            tunnel: [w1886] -> w1690
            tunnel: [w1885] -> w1689
            i -> [w1903]
            stop <- w1902 stop-if-true
            w1907 = T11 0 items=["PercentOutput"=0, "Position"=1, "Velocity"=2, "Current"=3, "Follower"=5, "MotionProfile"=6, "MotionMagic"=7, "MotionProfileArc"=10, "Disabled"=15] ("Control Mode")
            w1908 = T11 0 items=["PercentOutput"=0, "Position"=1, "Velocity"=2, "Current"=3, "Follower"=5, "MotionProfile"=6, "MotionMagic"=7, "MotionProfileArc"=10, "Disabled"=15] ("Control Mode")
            # "-0.186"
            # "-0.944"
            # ".135"
            n520 = call "Drive_Vi.vi"("Middle Thumb"=FALSE, "Z"=0.0, "Y"=-0.75, "X"=0.0) -> ()  [unwired: 8 in]
            n521 = call <vilib>:"CTRE_Phoenix_MotorControl_Set.vi"("error in (no error)"=w1891, "Output"=1.0, "Control Mode"=w1907, "PhoenixMotorControlDevRef"=w1892) -> ("error out"=w1887:errorcluster, "PhoenixMotorControlDevRef"=w1888:T7)  [unwired: 6 in]
            n522 = call <vilib>:"CTRE_Phoenix_MotorControl_Set.vi"("error in (no error)"=w1889, "Output"=0.0, "Control Mode"=w1908, "PhoenixMotorControlDevRef"=w1890) -> ("error out"=w1885:errorcluster, "PhoenixMotorControlDevRef"=w1886:T7)  [unwired: 6 in]
            n523 = Greater?(x=w1903, y=3) -> (0:w1902:bool)
            n524 = Wait (ms)(milliseconds to wait=u32 116) -> ()  [unwired: 1 out]
            n525 = call-poly <vilib>:"NT Read Value.vi"("Default Value"=0.0, "Name"="/limelight-drtrain/ty") -> ("Numeric"=w1894:dbl)  [unwired: 8 in, 1 out]
            "Ty 49" <- w1894
            n526 = call "Shooter_Equation.vi"("Right Trigger"=0.0, "Ty"=w1894) -> ()  [unwired: 10 in]
          }
          n527 = while {
            tunnel: w1692 -> [w1876]
            tunnel: w1691 -> [w1875]
            tunnel: w1690 -> [w1874]
            tunnel: w1689 -> [w1873]
            tunnel: [w1868] -> w1688
            tunnel: [w1867] -> w1687
            tunnel: [w1866] -> w1686
            tunnel: [w1865] -> w1685
            i -> [w1870]
            stop <- w1869 stop-if-true
            w1883 = T11 0 items=["PercentOutput"=0, "Position"=1, "Velocity"=2, "Current"=3, "Follower"=5, "MotionProfile"=6, "MotionMagic"=7, "MotionProfileArc"=10, "Disabled"=15] ("Control Mode")
            w1884 = T11 0 items=["PercentOutput"=0, "Position"=1, "Velocity"=2, "Current"=3, "Follower"=5, "MotionProfile"=6, "MotionMagic"=7, "MotionProfileArc"=10, "Disabled"=15] ("Control Mode")
            # "-0.186"
            # "-0.944"
            # ".135"
            n528 = call <vilib>:"CTRE_Phoenix_MotorControl_Set.vi"("error in (no error)"=w1875, "Output"=1.0, "Control Mode"=w1883, "PhoenixMotorControlDevRef"=w1876) -> ("error out"=w1867:errorcluster, "PhoenixMotorControlDevRef"=w1868:T7)  [unwired: 6 in]
            n529 = call <vilib>:"CTRE_Phoenix_MotorControl_Set.vi"("error in (no error)"=w1873, "Output"=0.0, "Control Mode"=w1884, "PhoenixMotorControlDevRef"=w1874) -> ("error out"=w1865:errorcluster, "PhoenixMotorControlDevRef"=w1866:T7)  [unwired: 6 in]
            n530 = call "Drive_Vi.vi"("Middle Thumb"=FALSE, "Z"=0.0, "Y"=0.0, "X"=0.0) -> ()  [unwired: 8 in]
            n531 = Greater?(x=w1870, y=35) -> (0:w1869:bool)
            n532 = call-poly <vilib>:"NT Read Value.vi"("Default Value"=0.0, "Name"="/limelight-drtrain/ty") -> ("Numeric"=w1878:dbl)  [unwired: 8 in, 1 out]
            "Ty 48" <- w1878
            n533 = Wait (ms)(milliseconds to wait=u32 100) -> ()  [unwired: 1 out]
            n534 = call "Shooter_Equation.vi"("Right Trigger"=0.0, "Ty"=w1878) -> ()  [unwired: 10 in]
          }
          n535 = while {
            tunnel: w1688 -> [w1848]
            tunnel: w1687 -> [w1847]
            tunnel: w1686 -> [w1846]
            tunnel: w1685 -> [w1845]
            tunnel: [w1840] -> w1684
            tunnel: [w1839] -> w1683
            tunnel: [w1838] -> w1682
            tunnel: [w1837] -> w1681
            tunnel: w1661 -> [w1831]
            tunnel: w1660 -> [w1832]
            tunnel: [w1832] -> w1659
            tunnel: [w1831] -> w1658
            i -> [w1842]
            stop <- w1841 stop-if-true
            w1859 = T11 0 items=["PercentOutput"=0, "Position"=1, "Velocity"=2, "Current"=3, "Follower"=5, "MotionProfile"=6, "MotionMagic"=7, "MotionProfileArc"=10, "Disabled"=15] ("Control Mode")
            w1860 = T11 0 items=["PercentOutput"=0, "Position"=1, "Velocity"=2, "Current"=3, "Follower"=5, "MotionProfile"=6, "MotionMagic"=7, "MotionProfileArc"=10, "Disabled"=15] ("Control Mode")
            # "-0.186"
            # "-0.944"
            # ".135"
            n536 = call "Turret_Aim.vi"("View Button"=FALSE, "Left Trigger"=0.0, "Orange Limit Pressed"=w1831, "Blue Limit Pressed"=w1832, "Right Bumper"=FALSE, "Left Bumper"=FALSE) -> ()  [unwired: 6 in]
            n537 = call "Drive_Vi.vi"("Middle Thumb"=FALSE, "Z"=0.0, "Y"=0.75, "X"=0.0) -> ()  [unwired: 8 in]
            n538 = call <vilib>:"CTRE_Phoenix_MotorControl_Set.vi"("error in (no error)"=w1847, "Output"=1.0, "Control Mode"=w1859, "PhoenixMotorControlDevRef"=w1848) -> ("error out"=w1839:errorcluster, "PhoenixMotorControlDevRef"=w1840:T7)  [unwired: 6 in]
            n539 = call <vilib>:"CTRE_Phoenix_MotorControl_Set.vi"("error in (no error)"=w1845, "Output"=-0.1, "Control Mode"=w1860, "PhoenixMotorControlDevRef"=w1846) -> ("error out"=w1837:errorcluster, "PhoenixMotorControlDevRef"=w1838:T7)  [unwired: 6 in]
            n540 = Greater?(x=w1842, y=5) -> (0:w1841:bool)
            n541 = Wait (ms)(milliseconds to wait=u32 50) -> ()  [unwired: 1 out]
            n542 = call-poly <vilib>:"NT Read Value.vi"("Default Value"=0.0, "Name"="/limelight-drtrain/ty") -> ("Numeric"=w1850:dbl)  [unwired: 8 in, 1 out]
            "Ty 47" <- w1850
            n543 = call "Shooter_Equation.vi"("Right Trigger"=0.0, "Ty"=w1850) -> ()  [unwired: 10 in]
          }
          n544 = while {
            tunnel: w1684 -> [w1818]
            tunnel: [w1811] -> _
            tunnel: w1682 -> [w1817]
            tunnel: w1681 -> [w1816]
            tunnel: w1683 -> [w1811]
            tunnel: [w1810] -> w1664
            tunnel: [w1809] -> w1663
            tunnel: [w1808] -> w1669
            tunnel: [w1807] -> w1667
            tunnel: w1659 -> [w1803]
            tunnel: w1658 -> [w1802]
            i -> [w1813]
            stop <- w1812 stop-if-true
            (unwired) FALSE ("Orange Limit Pressed")
            w1829 = T11 0 items=["PercentOutput"=0, "Position"=1, "Velocity"=2, "Current"=3, "Follower"=5, "MotionProfile"=6, "MotionMagic"=7, "MotionProfileArc"=10, "Disabled"=15] ("Control Mode")
            w1830 = T11 0 items=["PercentOutput"=0, "Position"=1, "Velocity"=2, "Current"=3, "Follower"=5, "MotionProfile"=6, "MotionMagic"=7, "MotionProfileArc"=10, "Disabled"=15] ("Control Mode")
            # "-0.186"
            # "-0.944"
            # ".135"
            n545 = call "Turret_Aim.vi"("View Button"=FALSE, "Left Trigger"=2.0, "Orange Limit Pressed"=w1802, "Blue Limit Pressed"=w1803, "Right Bumper"=FALSE, "Left Bumper"=FALSE) -> ()  [unwired: 6 in]
            n546 = call "Drive_Vi.vi"("Middle Thumb"=FALSE, "Z"=0.0, "Y"=-0.1, "X"=0.0) -> ()  [unwired: 8 in]
            n547 = call <vilib>:"CTRE_Phoenix_MotorControl_Set.vi"("error in (no error)"=w1811, "Output"=0.0, "Control Mode"=w1829, "PhoenixMotorControlDevRef"=w1818) -> ("error out"=w1807:errorcluster, "PhoenixMotorControlDevRef"=w1808:T7)  [unwired: 6 in]
            n548 = call <vilib>:"CTRE_Phoenix_MotorControl_Set.vi"("error in (no error)"=w1816, "Output"=-0.35, "Control Mode"=w1830, "PhoenixMotorControlDevRef"=w1817) -> ("error out"=w1810:errorcluster, "PhoenixMotorControlDevRef"=w1809:T7)  [unwired: 6 in]
            n549 = Greater?(x=w1813, y=10) -> (0:w1812:bool)
            n550 = Wait (ms)(milliseconds to wait=u32 100) -> ()  [unwired: 1 out]
            n551 = call-poly <vilib>:"NT Read Value.vi"("Default Value"=0.0, "Name"="/limelight-drtrain/ty") -> ("Numeric"=w1820:dbl)  [unwired: 8 in, 1 out]
            "Ty 46" <- w1820
            n552 = call "Shooter_Equation.vi"("Right Trigger"=2.0, "Ty"=w1820) -> ()  [unwired: 10 in]
          }
          n553 = while {
            tunnel: [w1746] -> w1668
            tunnel: w1669 -> [w1746]
            tunnel: [w1745] -> w1666
            tunnel: w1667 -> [w1745]
            tunnel: [w1744] -> w1665
            tunnel: w1664 -> [w1744]
            tunnel: [w1743] -> w1662
            tunnel: w1663 -> [w1743]
            i -> [w1736]
            stop <- w1735 stop-if-true
            n554 = Greater?(x=w1736, y=4) -> (0:w1735:bool)
            n555 = call "Drive_Vi.vi"("Middle Thumb"=TRUE, "Z"=0.15, "Y"=0.0, "X"=0.0) -> ()  [unwired: 8 in]
            n556 = Wait (ms)(milliseconds to wait=u32 100) -> ()  [unwired: 1 out]
          }
          n557 = while {
            tunnel: w1668 -> [w1788]
            tunnel: w1666 -> [w1781]
            tunnel: w1662 -> [w1787]
            tunnel: w1665 -> [w1786]
            i -> [w1783]
            stop <- w1782 stop-if-true
            w1799 = T11 0 items=["PercentOutput"=0, "Position"=1, "Velocity"=2, "Current"=3, "Follower"=5, "MotionProfile"=6, "MotionMagic"=7, "MotionProfileArc"=10, "Disabled"=15] ("Control Mode")
            w1800 = T11 0 items=["PercentOutput"=0, "Position"=1, "Velocity"=2, "Current"=3, "Follower"=5, "MotionProfile"=6, "MotionMagic"=7, "MotionProfileArc"=10, "Disabled"=15] ("Control Mode")
            # "-0.186"
            # "-0.944"
            # ".135"
            n558 = call "Drive_Vi.vi"("Middle Thumb"=FALSE, "Z"=0.0, "Y"=0.0, "X"=0.0) -> ()  [unwired: 8 in]
            n559 = call <vilib>:"CTRE_Phoenix_MotorControl_Set.vi"("error in (no error)"=w1781, "Output"=0.0, "Control Mode"=w1799, "PhoenixMotorControlDevRef"=w1788) -> ()  [unwired: 6 in, 2 out]
            n560 = call <vilib>:"CTRE_Phoenix_MotorControl_Set.vi"("error in (no error)"=w1786, "Output"=0.0, "Control Mode"=w1800, "PhoenixMotorControlDevRef"=w1787) -> ()  [unwired: 6 in, 2 out]
            n561 = Greater?(x=w1783, y=20) -> (0:w1782:bool)
            n562 = Wait (ms)(milliseconds to wait=u32 100) -> ()  [unwired: 1 out]
            n563 = call-poly <vilib>:"NT Read Value.vi"("Default Value"=0.0, "Name"="/limelight-drtrain/ty") -> ("Numeric"=w1790:dbl)  [unwired: 8 in, 1 out]
            "Ty 45" <- w1790
            n564 = call "Shooter_Equation.vi"("Right Trigger"=0.0, "Ty"=w1790) -> ()  [unwired: 10 in]
          }
        }
        frame "New VI Test" {
          # "Pigeon Set"
          n565 = flat-sequence {
            frame #0 {
              n566 = while {
                i -> [w2081]
                stop <- w2082 stop-if-true
                n567 = Wait (ms)(milliseconds to wait=u32 20) -> ()  [unwired: 1 out]
                n568 = Greater?(x=w2081, y=2) -> (0:w2082:bool)
                n569 = call "Drive_Vi.vi"("Middle Thumb"=TRUE, "Z"=0.0, "Y"=0.0, "X"=0.0) -> ()  [unwired: 8 in]
              }
            }
            frame #1 {
              n570 = while {
                i -> [w2110]
                stop <- w2084 stop-if-true
                n571 = call "Motor_Control.vi"("Output"=-0.55, "refnum"="Shoot") -> ()  [unwired: 10 in]
                n572 = call "Motor_Control.vi"("Output"=-0.2, "refnum"="Intake Actuate") -> ()  [unwired: 10 in]
                n573 = call <vilib>:"WPI_SwitchRefNum Registry Get.vi"("refnum name"="Intake Sensor") -> ("error out"=w2088:errorcluster, "SwitchDevRef"=w2087:T4)  [unwired: 9 in]
                n574 = call <vilib>:"WPI_SwitchRefNum Registry Get.vi"("refnum name"="Elevate Sensor") -> ("error out"=w2090:errorcluster, "SwitchDevRef"=w2089:T4)  [unwired: 9 in]
                n575 = Greater?(x=w2110, y=20) -> (0:w2084:bool)
                n576 = call <vilib>:"WPI_SwitchGetLimitValue.vi"("error in (no error)"=w2090, "SwitchDevRef"=w2089) -> ("Switch Pressed"=w2109:bool)  [unwired: 7 in, 2 out]
                n577 = call <vilib>:"WPI_SwitchGetLimitValue.vi"("error in (no error)"=w2088, "SwitchDevRef"=w2087) -> ("Switch Pressed"=w2108:bool)  [unwired: 7 in, 2 out]
                n578 = Not(x=w2109) -> (.not. x?=w2107:bool)
                "Elevate 12" <- w2107
                n579 = Not(x=w2108) -> (.not. x?=w2106:bool)
                "Intake 12" <- w2106
                n580 = global write "AutonBoolean.vi" "Boolean"(TRUE ("Boolean")) -> ()
                n581 = Wait (ms)(milliseconds to wait=u32 100) -> ()  [unwired: 1 out]
                n582 = case shown="True" w2107 {
                  tunnel: w2106 -> [_ w2126]
                  tunnel: [-0.1 ("Output") w2127] -> w2093
                  tunnel: [FALSE ("Middle Thumb") w2125] -> w2105
                  tunnel: [0.0 ("Z") w2124] -> w2104
                  tunnel: [0.0 ("Y") w2123] -> w2103
                  tunnel: [0.0 ("X") w2122] -> w2102
                  tunnel: [0.8 ("Output") w2121] -> w2097
                  tunnel: [0.75 ("Output") w2120] -> w2095
                  frame False {
                  }
                  frame True {
                    n583 = case shown="False" w2126 {
                      tunnel: [1.0 ("Output") 1.0 ("Output")] -> w2120
                      tunnel: [0.0 ("Output") 0.0 ("Output")] -> w2127
                      tunnel: [FALSE ("Middle Thumb") FALSE ("Middle Thumb")] -> w2125
                      tunnel: [0.0 ("Z") 0.0 ("Z")] -> w2124
                      tunnel: [-0.3 ("Y") 0.0 ("Y")] -> w2123
                      tunnel: [0.0 ("X") 0.0 ("X")] -> w2122
                      tunnel: [1.0 ("Output") 0.0 ("Output")] -> w2121
                      frame False {
                      }
                      frame True {
                      }
                    }
                  }
                }
                n584 = call "Drive_Vi.vi"("Middle Thumb"=w2105, "Z"=w2104, "Y"=w2103, "X"=w2102) -> ()  [unwired: 8 in]
                n585 = call "Motor_Control.vi"("Output"=w2097, "refnum"="Intake") -> ()  [unwired: 10 in]
                n586 = call "Motor_Control.vi"("Output"=w2093, "refnum"="Elevate") -> ()  [unwired: 10 in]
                n587 = call "Motor_Control.vi"("Output"=w2095, "refnum"="Reject") -> ()  [unwired: 10 in]
              }
            }
            frame #2 {
              n588 = while {
                i -> [w2158]
                stop <- w2157 stop-if-true
                n589 = call <vilib>:"WPI_SwitchRefNum Registry Get.vi"("refnum name"="Blue Limit Switch") -> ("error out"=w2145:errorcluster, "SwitchDevRef"=w2144:T4)  [unwired: 9 in]
                n590 = call <vilib>:"WPI_SwitchRefNum Registry Get.vi"("refnum name"="Orange Limit Switch") -> ("error out"=w2147:errorcluster, "SwitchDevRef"=w2146:T4)  [unwired: 9 in]
                n591 = Greater?(x=w2158, y=5) -> (0:w2157:bool)
                n592 = call <vilib>:"WPI_SwitchGetLimitValue.vi"("error in (no error)"=w2145, "SwitchDevRef"=w2144) -> ("Switch Pressed"=w2167:bool)  [unwired: 7 in, 2 out]
                "Blue Limit Pressed 23" <- w2167
                n593 = call <vilib>:"WPI_SwitchGetLimitValue.vi"("error in (no error)"=w2147, "SwitchDevRef"=w2146) -> ("Switch Pressed"=w2168:bool)  [unwired: 7 in, 2 out]
                "Orange Limit Pressed 23" <- w2168
                n594 = call "Motor_Control.vi"("Output"=0.0, "refnum"="Intake") -> ()  [unwired: 10 in]
                n595 = call-poly <vilib>:"NT Read Value.vi"("Default Value"=0.0, "Name"="/limelight-drtrain/ty") -> ("Numeric"=w2162:dbl)  [unwired: 8 in, 1 out]
                "Ty 53" <- w2162
                n596 = call "Shooter_Equation.vi"("Right Trigger"=2.0, "Ty"=w2162) -> ()  [unwired: 10 in]
                n597 = call "Turret_Aim.vi"("View Button"=FALSE ("Driver Right Thumb"), "Left Trigger"=2.0, "Orange Limit Pressed"=w2167, "Blue Limit Pressed"=w2168, "Right Bumper"=FALSE, "Left Bumper"=FALSE) -> ()  [unwired: 6 in]
                n598 = Wait (ms)(milliseconds to wait=u32 100) -> ()  [unwired: 1 out]
                n599 = call "Drive_Vi.vi"("Middle Thumb"=FALSE, "Z"=0.0, "Y"=0.15, "X"=0.0) -> ()  [unwired: 8 in]
                n600 = global write "AutonBoolean.vi" "Boolean"(FALSE ("Boolean")) -> ()
                n601 = call "Motor_Control.vi"("Output"=0.0, "refnum"="Intake Actuate") -> ()  [unwired: 10 in]
              }
            }
            frame #3 {
              n602 = while {
                i -> [w2186]
                stop <- w2185 stop-if-true
                n603 = Greater?(x=w2186, y=50) -> (0:w2185:bool)
                n604 = call <vilib>:"WPI_SwitchRefNum Registry Get.vi"("refnum name"="Orange Limit Switch") -> ("error out"=w2174:errorcluster, "SwitchDevRef"=w2175:T4)  [unwired: 9 in]
                n605 = call <vilib>:"WPI_SwitchGetLimitValue.vi"("error in (no error)"=w2174, "SwitchDevRef"=w2175) -> ("Switch Pressed"=w2196:bool)  [unwired: 7 in, 2 out]
                "Orange Limit Pressed 24" <- w2196
                n606 = call <vilib>:"WPI_SwitchRefNum Registry Get.vi"("refnum name"="Blue Limit Switch") -> ("error out"=w2171:errorcluster, "SwitchDevRef"=w2172:T4)  [unwired: 9 in]
                n607 = call <vilib>:"WPI_SwitchGetLimitValue.vi"("error in (no error)"=w2171, "SwitchDevRef"=w2172) -> ("Switch Pressed"=w2195:bool)  [unwired: 7 in, 2 out]
                "Blue Limit Pressed 24" <- w2195
                n608 = call "Turret_Aim.vi"("View Button"=FALSE ("Driver Right Thumb"), "Left Trigger"=2.0, "Orange Limit Pressed"=w2195, "Blue Limit Pressed"=w2196, "Right Bumper"=FALSE, "Left Bumper"=FALSE) -> ()  [unwired: 6 in]
                n609 = Wait (ms)(milliseconds to wait=u32 100) -> ()  [unwired: 1 out]
                n610 = call "Drive_Vi.vi"("Middle Thumb"=FALSE, "Z"=0.0, "Y"=0.15, "X"=0.0) -> ()  [unwired: 8 in]
                n611 = call "Motor_Control.vi"("Output"=0.35, "refnum"="Intake") -> ()  [unwired: 10 in]
                n612 = call "Motor_Control.vi"("Output"=-0.35, "refnum"="Elevate") -> ()  [unwired: 10 in]
                n613 = call-poly <vilib>:"NT Read Value.vi"("Default Value"=0.0, "Name"="/limelight-drtrain/ty") -> ("Numeric"=w2190:dbl)  [unwired: 8 in, 1 out]
                "Ty 54" <- w2190
                n614 = call "Shooter_Equation.vi"("Right Trigger"=2.0, "Ty"=w2190) -> ()  [unwired: 10 in]
              }
            }
            frame #4 {
              n615 = while {
                i -> [w2208]
                stop <- w2207 stop-if-true
                n616 = Wait (ms)(milliseconds to wait=u32 112) -> ()  [unwired: 1 out]
                n617 = call "Drive_Vi.vi"("Middle Thumb"=FALSE, "Z"=0.35, "Y"=0.0, "X"=0.0) -> ()  [unwired: 8 in]
                n618 = Greater?(x=w2208, y=10) -> (0:w2207:bool)
                n619 = call-poly <vilib>:"NT Read Value.vi"("Default Value"=0.0, "Name"="/limelight-drtrain/ty") -> ("Numeric"=w2212:dbl)  [unwired: 8 in, 1 out]
                "Ty 55" <- w2212
                n620 = call "Shooter_Equation.vi"("Right Trigger"=0.0, "Ty"=w2212) -> ()  [unwired: 10 in]
                n621 = call "Motor_Control.vi"("Output"=-0.35, "refnum"="Elevate") -> ()  [unwired: 10 in]
                n622 = call "Motor_Control.vi"("Output"=0.35, "refnum"="Intake") -> ()  [unwired: 10 in]
              }
            }
            frame #5 {
              n623 = while {
                i -> [w2224]
                stop <- w2223 stop-if-true
                n624 = Wait (ms)(milliseconds to wait=u32 20) -> ()  [unwired: 1 out]
                n625 = Greater?(x=w2224, y=2) -> (0:w2223:bool)
                n626 = call "Drive_Vi.vi"("Middle Thumb"=TRUE, "Z"=0.0, "Y"=0.0, "X"=0.0) -> ()  [unwired: 8 in]
                n627 = call-poly <vilib>:"NT Read Value.vi"("Default Value"=0.0, "Name"="/limelight-drtrain/ty") -> ("Numeric"=w2228:dbl)  [unwired: 8 in, 1 out]
                "Ty 56" <- w2228
                n628 = call "Shooter_Equation.vi"("Right Trigger"=0.0, "Ty"=w2228) -> ()  [unwired: 10 in]
                n629 = call "Motor_Control.vi"("Output"=0.35, "refnum"="Intake") -> ()  [unwired: 10 in]
                n630 = call "Motor_Control.vi"("Output"=-0.35, "refnum"="Elevate") -> ()  [unwired: 10 in]
              }
            }
            frame #6 {
              n631 = while {
                i -> [w2241]
                stop <- w2240 stop-if-true
                n632 = Wait (ms)(milliseconds to wait=u32 100) -> ()  [unwired: 1 out]
                n633 = call "Motor_Control.vi"("Output"=0.0, "refnum"="Elevate") -> ()  [unwired: 10 in]
                n634 = call "Motor_Control.vi"("Output"=0.0, "refnum"="Intake") -> ()  [unwired: 10 in]
                n635 = Greater?(x=w2241, y=50) -> (0:w2240:bool)
                n636 = call "Drive_Vi.vi"("Middle Thumb"=FALSE, "Z"=0.0, "Y"=0.0, "X"=0.0) -> ()  [unwired: 8 in]
              }
            }
          }
        }
      }
      n637 = for {
        N: 20 -> [_]
        (unwired) FALSE ("Middle Thumb")
        (unwired) 0.0 ("Z")
        (unwired) -0.1 ("Y")
        (unwired) 0.0 ("X")
        n638 = Wait (ms)(milliseconds to wait=u32 100) -> ()  [unwired: 1 out]
        n639 = call "Drive_Vi.vi"() -> ()  [unwired: 12 in]
      }
    }
    frame "Taxi + Shoot 1" {
      # "Pigeon Set"
      n640 = call <vilib>:"WPI_SwitchRefNum Registry Get.vi"("refnum name"="Intake Sensor") -> ("error out"=w2251:errorcluster, "SwitchDevRef"=w2253:T4)  [unwired: 9 in]
      n641 = call <vilib>:"WPI_SolenoidRefNum Registry Get.vi"("refnum name"="Intake Solenoid") -> ("error out"=w2270:errorcluster, "SolenoidDevRef"=w2272:T12)  [unwired: 9 in]
      n642 = call <vilib>:"CTRE_Phoenix_MotorControl_RefNumRegistryGet.vi"("refnum name"="Intake") -> ("error out"=w2265:errorcluster, "PhoenixMotorControlDevRef"=w2267:T7)  [unwired: 9 in]
      n643 = call <vilib>:"CTRE_Phoenix_MotorControl_RefNumRegistryGet.vi"("refnum name"="Reject") -> ("error out"=w2301:errorcluster, "PhoenixMotorControlDevRef"=w2263:T7)  [unwired: 9 in]
      n644 = call "Limit_Switches.vi"() -> ()  [unwired: 10 in, 2 out]
      n645 = call <vilib>:"CTRE_Phoenix_MotorControl_RefNumRegistryGet.vi"("refnum name"="Elevate") -> ("error out"=w2259:errorcluster, "PhoenixMotorControlDevRef"=w2261:T7)  [unwired: 9 in]
      n646 = call <vilib>:"WPI_SwitchRefNum Registry Get.vi"("refnum name"="Elevate Sensor") -> ("error out"=w2255:errorcluster, "SwitchDevRef"=w2257:T4)  [unwired: 9 in]
      n647 = call <vilib>:"CTRE_Phoenix_MotorControl_RefNumRegistryGet.vi"("refnum name"="Shoot") -> ("error out"=w2247:errorcluster, "PhoenixMotorControlDevRef"=w2250:T7)  [unwired: 9 in]
      n648 = while {
        tunnel: [w2325] -> w2271
        tunnel: w2272 -> [w2325]
        tunnel: [w2324] -> w2269
        tunnel: w2270 -> [w2324]
        tunnel: [w2323] -> w2268
        tunnel: w2267 -> [w2323]
        tunnel: [w2322] -> w2266
        tunnel: w2265 -> [w2322]
        tunnel: [w2321] -> w2264
        tunnel: w2263 -> [w2321]
        tunnel: [w2320] -> w2262
        tunnel: w2261 -> [w2320]
        tunnel: [w2319] -> w2260
        tunnel: w2259 -> [w2319]
        tunnel: [w2318] -> w2258
        tunnel: w2257 -> [w2318]
        tunnel: [w2317] -> w2256
        tunnel: w2255 -> [w2317]
        tunnel: [w2316] -> w2254
        tunnel: w2253 -> [w2316]
        tunnel: [w2315] -> w2252
        tunnel: w2251 -> [w2315]
        tunnel: [w2314] -> w2249
        tunnel: w2250 -> [w2314]
        tunnel: [w2313] -> w2248
        tunnel: w2247 -> [w2313]
        i -> [w2309]
        stop <- w2311 stop-if-true
        n649 = Wait (ms)(milliseconds to wait=u32 100) -> ()  [unwired: 1 out]
        n650 = call "Drive_Vi.vi"("Middle Thumb"=FALSE, "Z"=0.0, "Y"=0.0, "X"=0.0) -> ()  [unwired: 8 in]
        n651 = Greater?(x=w2309, y=100) -> (0:w2311:bool)
      }
      n652 = while {
        i -> [w2499]
        stop <- w2500 stop-if-true
        n653 = Wait (ms)(milliseconds to wait=u32 20) -> ()  [unwired: 1 out]
        n654 = Greater?(x=w2499, y=2) -> (0:w2500:bool)
        n655 = call "Drive_Vi.vi"("Middle Thumb"=TRUE, "Z"=0.0, "Y"=0.0, "X"=0.0) -> ()  [unwired: 8 in]
      }
      n656 = while {
        tunnel: w2256 -> [w2454]
        tunnel: w2258 -> [w2453]
        tunnel: w2252 -> [w2452]
        tunnel: w2254 -> [w2451]
        tunnel: w2269 -> [w2450]
        tunnel: w2271 -> [w2449]
        tunnel: w2260 -> [w2446]
        tunnel: w2262 -> [w2445]
        tunnel: w2301 -> [w2444]
        tunnel: w2264 -> [w2443]
        tunnel: w2266 -> [w2442]
        tunnel: w2268 -> [w2441]
        tunnel: [w2429] -> w2294
        tunnel: [w2428] -> w2293
        tunnel: [w2427] -> w2292
        tunnel: [w2426] -> w2291
        tunnel: w2248 -> [w2425]
        tunnel: w2249 -> [w2424]
        tunnel: [w2421] -> w2290
        tunnel: [w2420] -> w2289
        tunnel: [w2419] -> w2282
        tunnel: [w2418] -> w2281
        i -> [w2457]
        stop <- w2458 stop-if-true
        w2423 = T11 0 items=["PercentOutput"=0, "Position"=1, "Velocity"=2, "Current"=3, "Follower"=5, "MotionProfile"=6, "MotionMagic"=7, "MotionProfileArc"=10, "Disabled"=15] ("Control Mode")
        w2435 = T11 0 items=["PercentOutput"=0, "Position"=1, "Velocity"=2, "Current"=3, "Follower"=5, "MotionProfile"=6, "MotionMagic"=7, "MotionProfileArc"=10, "Disabled"=15] ("Control Mode")
        w2436 = T11 0 items=["PercentOutput"=0, "Position"=1, "Velocity"=2, "Current"=3, "Follower"=5, "MotionProfile"=6, "MotionMagic"=7, "MotionProfileArc"=10, "Disabled"=15] ("Control Mode")
        w2437 = T11 0 items=["PercentOutput"=0, "Position"=1, "Velocity"=2, "Current"=3, "Follower"=5, "MotionProfile"=6, "MotionMagic"=7, "MotionProfileArc"=10, "Disabled"=15] ("Control Mode")
        n657 = call <vilib>:"WPI_SwitchGetLimitValue.vi"("error in (no error)"=w2452, "SwitchDevRef"=w2451) -> ("Switch Pressed"=w2455:bool)  [unwired: 7 in, 2 out]
        n658 = call <vilib>:"WPI_SwitchGetLimitValue.vi"("error in (no error)"=w2454, "SwitchDevRef"=w2453) -> ("Switch Pressed"=w2456:bool)  [unwired: 7 in, 2 out]
        n659 = Greater?(x=w2457, y=20) -> (0:w2458:bool)
        n660 = Not(x=w2455) -> (.not. x?=w2440:bool)
        "Intake 4" <- w2440
        n661 = Not(x=w2456) -> (.not. x?=w2448:bool)
        "Elevate 4" <- w2448
        n662 = Wait (ms)(milliseconds to wait=u32 100) -> ()  [unwired: 1 out]
        n663 = case shown="True" w2448 {
          tunnel: [0.75 ("Output") w2477] -> w2447
          tunnel: w2440 -> [_ w2474]
          tunnel: [0.75 ("Output") w2476] -> w2439
          tunnel: [-0.1 ("Output") w2475] -> w2438
          tunnel: [FALSE ("Middle Thumb") w2473] -> w2434
          tunnel: [0.0 ("Z") w2472] -> w2433
          tunnel: [0.0 ("Y") w2471] -> w2432
          tunnel: [0.0 ("X") w2470] -> w2431
          tunnel: [WPI_SolenoidValue."Reverse" ("Value") w2469] -> w2430
          frame False {
          }
          frame True {
            n664 = case shown="False" w2474 {
              tunnel: [0.75 ("Output") 0.0 ("Output")] -> w2477
              tunnel: [0.0 ("Output") 0.0 ("Output")] -> w2476
              tunnel: [0.0 ("Output") 0.0 ("Output")] -> w2475
              tunnel: [FALSE ("Middle Thumb") FALSE ("Middle Thumb")] -> w2473
              tunnel: [0.0 ("Z") 0.0 ("Z")] -> w2472
              tunnel: [-0.3 ("Y") 0.0 ("Y")] -> w2471
              tunnel: [0.0 ("X") 0.0 ("X")] -> w2470
              tunnel: [WPI_SolenoidValue."Forward" ("Value") WPI_SolenoidValue."Forward" ("Value")] -> w2469
              frame False {
              }
              frame True {
              }
            }
          }
        }
        n665 = call-poly <vilib>:"WPI_SolenoidSet.vi"("error in (no error)"=w2450, "Value"=w2430, "SolenoidDevRef"=w2449) -> ("error out"=w2418:errorcluster, "SolenoidDevRef"=w2419:T12)  [unwired: 7 in]
        n666 = call <vilib>:"CTRE_Phoenix_MotorControl_Set.vi"("error in (no error)"=w2442, "Output"=w2447, "Control Mode"=w2435, "PhoenixMotorControlDevRef"=w2441) -> ("error out"=w2427:errorcluster, "PhoenixMotorControlDevRef"=w2426:T7)  [unwired: 6 in]
        n667 = call <vilib>:"CTRE_Phoenix_MotorControl_Set.vi"("error in (no error)"=w2444, "Output"=w2439, "Control Mode"=w2436, "PhoenixMotorControlDevRef"=w2443) -> ()  [unwired: 6 in, 2 out]
        n668 = call <vilib>:"CTRE_Phoenix_MotorControl_Set.vi"("error in (no error)"=w2446, "Output"=w2438, "Control Mode"=w2437, "PhoenixMotorControlDevRef"=w2445) -> ("error out"=w2429:errorcluster, "PhoenixMotorControlDevRef"=w2428:T7)  [unwired: 6 in]
        n669 = call <vilib>:"CTRE_Phoenix_MotorControl_Set.vi"("error in (no error)"=w2425, "Output"=-0.55, "Control Mode"=w2423, "PhoenixMotorControlDevRef"=w2424) -> ("error out"=w2421:errorcluster, "PhoenixMotorControlDevRef"=w2420:T7)  [unwired: 6 in]
        n670 = call "Drive_Vi.vi"("Middle Thumb"=w2434, "Z"=w2433, "Y"=w2432, "X"=w2431) -> ()  [unwired: 8 in]
      }
      n671 = call <vilib>:"WPI_SwitchRefNum Registry Get.vi"("refnum name"="Orange Limit Switch") -> ("error out"=w2296:errorcluster, "SwitchDevRef"=w2295:T4)  [unwired: 9 in]
      n672 = call <vilib>:"WPI_SwitchRefNum Registry Get.vi"("refnum name"="Blue Limit Switch") -> ("error out"=w2298:errorcluster, "SwitchDevRef"=w2297:T4)  [unwired: 9 in]
      n673 = while {
        tunnel: w2290 -> [_]
        tunnel: w2289 -> [_]
        tunnel: w2298 -> [w2415]
        tunnel: w2297 -> [w2414]
        tunnel: w2296 -> [w2413]
        tunnel: w2295 -> [w2412]
        tunnel: w2294 -> [w2391]
        tunnel: w2293 -> [w2390]
        tunnel: w2292 -> [w2381]
        tunnel: w2291 -> [w2382]
        tunnel: [w2395] -> w2288
        tunnel: [w2394] -> w2287
        tunnel: [w2393] -> w2286
        tunnel: [w2392] -> w2285
        tunnel: [w2391] -> w2284
        tunnel: [w2390] -> w2283
        tunnel: w2282 -> [w2389]
        tunnel: w2281 -> [w2388]
        tunnel: [w2386] -> w2280
        tunnel: [w2385] -> w2279
        tunnel: [w2384] -> w2278
        tunnel: [w2383] -> w2277
        i -> [w2401]
        stop <- w2400 stop-if-true
        w2380 = T11 0 items=["PercentOutput"=0, "Position"=1, "Velocity"=2, "Current"=3, "Follower"=5, "MotionProfile"=6, "MotionMagic"=7, "MotionProfileArc"=10, "Disabled"=15] ("Control Mode")
        n674 = call-poly <vilib>:"WPI_SolenoidSet.vi"("error in (no error)"=w2388, "Value"=WPI_SolenoidValue."Forward", "SolenoidDevRef"=w2389) -> ("error out"=w2385:errorcluster, "SolenoidDevRef"=w2386:T12)  [unwired: 7 in]
        n675 = call <vilib>:"WPI_SwitchGetLimitValue.vi"("error in (no error)"=w2413, "SwitchDevRef"=w2412) -> ("error out"=w2392:errorcluster, "Switch Pressed"=w2411:bool, "SwitchDevRef"=w2393:T4)  [unwired: 7 in]
        "Orange Limit Pressed 7" <- w2411
        n676 = call <vilib>:"WPI_SwitchGetLimitValue.vi"("error in (no error)"=w2415, "SwitchDevRef"=w2414) -> ("error out"=w2394:errorcluster, "Switch Pressed"=w2410:bool, "SwitchDevRef"=w2395:T4)  [unwired: 7 in]
        "Blue Limit Pressed 7" <- w2410
        n677 = call-poly <vilib>:"NT Read Value.vi"("Default Value"=0.0, "Name"="/limelight-drtrain/ty") -> ("Numeric"=w2405:dbl)  [unwired: 8 in, 1 out]
        "Ty 7" <- w2405
        n678 = Greater?(x=w2401, y=5) -> (0:w2400:bool)
        n679 = call "Turret_Aim.vi"("View Button"=FALSE ("Driver Right Thumb"), "Left Trigger"=2.0, "Orange Limit Pressed"=w2410, "Blue Limit Pressed"=w2411, "Right Bumper"=FALSE, "Left Bumper"=FALSE) -> ()  [unwired: 6 in]
        n680 = call "Shooter_Equation.vi"("Right Trigger"=2.0, "Ty"=w2405) -> ()  [unwired: 10 in]
        n681 = Wait (ms)(milliseconds to wait=u32 100) -> ()  [unwired: 1 out]
        n682 = call "Drive_Vi.vi"("Middle Thumb"=FALSE, "Z"=0.0, "Y"=0.15, "X"=0.0) -> ()  [unwired: 8 in]
        n683 = call <vilib>:"CTRE_Phoenix_MotorControl_Set.vi"("error in (no error)"=w2381, "Output"=0.0, "Control Mode"=w2380, "PhoenixMotorControlDevRef"=w2382) -> ("error out"=w2383:errorcluster, "PhoenixMotorControlDevRef"=w2384:T7)  [unwired: 6 in]
      }
      n684 = while {
        tunnel: w2287 -> [w2376]
        tunnel: w2288 -> [w2375]
        tunnel: w2285 -> [w2374]
        tunnel: w2284 -> [w2361]
        tunnel: w2283 -> [w2360]
        tunnel: w2277 -> [w2359]
        tunnel: w2278 -> [w2358]
        tunnel: w2286 -> [w2349]
        tunnel: w2280 -> [w2348]
        tunnel: w2279 -> [w2347]
        tunnel: [w2345] -> w2276
        tunnel: [w2344] -> w2275
        tunnel: [w2343] -> w2274
        tunnel: [w2342] -> w2273
        i -> [w2363]
        stop <- w2362 stop-if-true
        w2356 = T11 0 items=["PercentOutput"=0, "Position"=1, "Velocity"=2, "Current"=3, "Follower"=5, "MotionProfile"=6, "MotionMagic"=7, "MotionProfileArc"=10, "Disabled"=15] ("Control Mode")
        w2357 = T11 0 items=["PercentOutput"=0, "Position"=1, "Velocity"=2, "Current"=3, "Follower"=5, "MotionProfile"=6, "MotionMagic"=7, "MotionProfileArc"=10, "Disabled"=15] ("Control Mode")
        n685 = call-poly <vilib>:"WPI_SolenoidSet.vi"("error in (no error)"=w2347, "Value"=WPI_SolenoidValue."Off", "SolenoidDevRef"=w2348) -> ()  [unwired: 7 in, 2 out]
        n686 = call <vilib>:"WPI_SwitchGetLimitValue.vi"("error in (no error)"=w2374, "SwitchDevRef"=w2349) -> ("Switch Pressed"=w2373:bool)  [unwired: 7 in, 2 out]
        "Orange Limit Pressed 8" <- w2373
        n687 = call <vilib>:"WPI_SwitchGetLimitValue.vi"("error in (no error)"=w2376, "SwitchDevRef"=w2375) -> ("Switch Pressed"=w2372:bool)  [unwired: 7 in, 2 out]
        "Blue Limit Pressed 8" <- w2372
        n688 = call-poly <vilib>:"NT Read Value.vi"("Default Value"=0.0, "Name"="/limelight-drtrain/ty") -> ("Numeric"=w2367:dbl)  [unwired: 8 in, 1 out]
        "Ty 8" <- w2367
        n689 = Greater?(x=w2363, y=50) -> (0:w2362:bool)
        n690 = call "Turret_Aim.vi"("View Button"=FALSE ("Driver Right Thumb"), "Left Trigger"=2.0, "Orange Limit Pressed"=w2372, "Blue Limit Pressed"=w2373, "Right Bumper"=FALSE, "Left Bumper"=FALSE) -> ()  [unwired: 6 in]
        n691 = call "Shooter_Equation.vi"("Right Trigger"=2.0, "Ty"=w2367) -> ()  [unwired: 10 in]
        n692 = Wait (ms)(milliseconds to wait=u32 100) -> ()  [unwired: 1 out]
        n693 = call "Drive_Vi.vi"("Middle Thumb"=FALSE, "Z"=0.0, "Y"=0.15, "X"=0.0) -> ()  [unwired: 8 in]
        n694 = call <vilib>:"CTRE_Phoenix_MotorControl_Set.vi"("error in (no error)"=w2359, "Output"=0.35, "Control Mode"=w2356, "PhoenixMotorControlDevRef"=w2358) -> ("error out"=w2345:errorcluster, "PhoenixMotorControlDevRef"=w2344:T7)  [unwired: 6 in]
        n695 = call <vilib>:"CTRE_Phoenix_MotorControl_Set.vi"("error in (no error)"=w2361, "Output"=-0.35, "Control Mode"=w2357, "PhoenixMotorControlDevRef"=w2360) -> ("error out"=w2342:errorcluster, "PhoenixMotorControlDevRef"=w2343:T7)  [unwired: 6 in]
      }
      n696 = while {
        tunnel: w2276 -> [w2337]
        tunnel: w2275 -> [w2336]
        tunnel: w2274 -> [w2335]
        tunnel: w2273 -> [w2334]
        i -> [w2332]
        stop <- w2331 stop-if-true
        w2340 = T11 0 items=["PercentOutput"=0, "Position"=1, "Velocity"=2, "Current"=3, "Follower"=5, "MotionProfile"=6, "MotionMagic"=7, "MotionProfileArc"=10, "Disabled"=15] ("Control Mode")
        w2341 = T11 0 items=["PercentOutput"=0, "Position"=1, "Velocity"=2, "Current"=3, "Follower"=5, "MotionProfile"=6, "MotionMagic"=7, "MotionProfileArc"=10, "Disabled"=15] ("Control Mode")
        n697 = call <vilib>:"CTRE_Phoenix_MotorControl_Set.vi"("error in (no error)"=w2337, "Output"=0.0, "Control Mode"=w2340, "PhoenixMotorControlDevRef"=w2336) -> ()  [unwired: 6 in, 2 out]
        n698 = call <vilib>:"CTRE_Phoenix_MotorControl_Set.vi"("error in (no error)"=w2334, "Output"=0.0, "Control Mode"=w2341, "PhoenixMotorControlDevRef"=w2335) -> ()  [unwired: 6 in, 2 out]
        n699 = Greater?(x=w2332, y=50) -> (0:w2331:bool)
        n700 = Wait (ms)(milliseconds to wait=u32 100) -> ()  [unwired: 1 out]
      }
    }
    frame "1 Ball + Reject" {
      # "Pigeon Set"
      n701 = while {
        i -> [w2720]
        stop <- w2721 stop-if-true
        n702 = Wait (ms)(milliseconds to wait=u32 20) -> ()  [unwired: 1 out]
        n703 = Greater?(x=w2720, y=2) -> (0:w2721:bool)
        n704 = call "Drive_Vi.vi"("Middle Thumb"=TRUE, "Z"=0.0, "Y"=0.0, "X"=0.0) -> ()  [unwired: 8 in]
      }
      n705 = call <vilib>:"WPI_SwitchRefNum Registry Get.vi"("refnum name"="Intake Sensor") -> ("error out"=w2541:errorcluster, "SwitchDevRef"=w2540:T4)  [unwired: 9 in]
      n706 = call <vilib>:"WPI_SolenoidRefNum Registry Get.vi"("refnum name"="Intake Solenoid") -> ("error out"=w2539:errorcluster, "SolenoidDevRef"=w2538:T12)  [unwired: 9 in]
      n707 = call <vilib>:"CTRE_Phoenix_MotorControl_RefNumRegistryGet.vi"("refnum name"="Intake") -> ("error out"=w2533:errorcluster, "PhoenixMotorControlDevRef"=w2532:T7)  [unwired: 9 in]
      n708 = call <vilib>:"CTRE_Phoenix_MotorControl_RefNumRegistryGet.vi"("refnum name"="Reject") -> ("error out"=w2535:errorcluster, "PhoenixMotorControlDevRef"=w2534:T7)  [unwired: 9 in]
      n709 = call "Limit_Switches.vi"() -> ()  [unwired: 10 in, 2 out]
      n710 = call <vilib>:"CTRE_Phoenix_MotorControl_RefNumRegistryGet.vi"("refnum name"="Elevate") -> ("error out"=w2537:errorcluster, "PhoenixMotorControlDevRef"=w2536:T7)  [unwired: 9 in]
      n711 = call <vilib>:"WPI_SwitchRefNum Registry Get.vi"("refnum name"="Elevate Sensor") -> ("error out"=w2543:errorcluster, "SwitchDevRef"=w2542:T4)  [unwired: 9 in]
      n712 = call <vilib>:"CTRE_Phoenix_MotorControl_RefNumRegistryGet.vi"("refnum name"="Shoot") -> ("error out"=w2521:errorcluster, "PhoenixMotorControlDevRef"=w2520:T7)  [unwired: 9 in]
      n713 = while {
        tunnel: w2543 -> [w2675]
        tunnel: w2542 -> [w2674]
        tunnel: w2541 -> [w2673]
        tunnel: w2540 -> [w2672]
        tunnel: w2539 -> [w2671]
        tunnel: w2538 -> [w2670]
        tunnel: w2537 -> [w2667]
        tunnel: w2536 -> [w2666]
        tunnel: w2535 -> [w2665]
        tunnel: w2534 -> [w2664]
        tunnel: w2533 -> [w2663]
        tunnel: w2532 -> [w2662]
        tunnel: [w2650] -> w2525
        tunnel: [w2649] -> w2524
        tunnel: [w2648] -> w2523
        tunnel: [w2647] -> w2522
        tunnel: w2521 -> [w2646]
        tunnel: w2520 -> [w2645]
        tunnel: [w2642] -> w2519
        tunnel: [w2641] -> w2518
        tunnel: [w2640] -> w2511
        tunnel: [w2639] -> w2510
        i -> [w2678]
        stop <- w2679 stop-if-true
        w2644 = T11 0 items=["PercentOutput"=0, "Position"=1, "Velocity"=2, "Current"=3, "Follower"=5, "MotionProfile"=6, "MotionMagic"=7, "MotionProfileArc"=10, "Disabled"=15] ("Control Mode")
        w2656 = T11 0 items=["PercentOutput"=0, "Position"=1, "Velocity"=2, "Current"=3, "Follower"=5, "MotionProfile"=6, "MotionMagic"=7, "MotionProfileArc"=10, "Disabled"=15] ("Control Mode")
        w2657 = T11 0 items=["PercentOutput"=0, "Position"=1, "Velocity"=2, "Current"=3, "Follower"=5, "MotionProfile"=6, "MotionMagic"=7, "MotionProfileArc"=10, "Disabled"=15] ("Control Mode")
        w2658 = T11 0 items=["PercentOutput"=0, "Position"=1, "Velocity"=2, "Current"=3, "Follower"=5, "MotionProfile"=6, "MotionMagic"=7, "MotionProfileArc"=10, "Disabled"=15] ("Control Mode")
        n714 = call <vilib>:"WPI_SwitchGetLimitValue.vi"("error in (no error)"=w2673, "SwitchDevRef"=w2672) -> ("Switch Pressed"=w2676:bool)  [unwired: 7 in, 2 out]
        n715 = call <vilib>:"WPI_SwitchGetLimitValue.vi"("error in (no error)"=w2675, "SwitchDevRef"=w2674) -> ("Switch Pressed"=w2677:bool)  [unwired: 7 in, 2 out]
        n716 = Greater?(x=w2678, y=20) -> (0:w2679:bool)
        n717 = Not(x=w2676) -> (.not. x?=w2661:bool)
        "Intake 3" <- w2661
        n718 = Not(x=w2677) -> (.not. x?=w2669:bool)
        "Elevate 3" <- w2669
        n719 = Wait (ms)(milliseconds to wait=u32 100) -> ()  [unwired: 1 out]
        n720 = case shown="True" w2669 {
          tunnel: [0.75 ("Output") w2698] -> w2668
          tunnel: w2661 -> [_ w2695]
          tunnel: [0.75 ("Output") w2697] -> w2660
          tunnel: [-0.1 ("Output") w2696] -> w2659
          tunnel: [FALSE ("Middle Thumb") w2694] -> w2655
          tunnel: [0.0 ("Z") w2693] -> w2654
          tunnel: [0.0 ("Y") w2692] -> w2653
          tunnel: [0.0 ("X") w2691] -> w2652
          tunnel: [WPI_SolenoidValue."Reverse" ("Value") w2690] -> w2651
          frame False {
          }
          frame True {
            n721 = case shown="False" w2695 {
              tunnel: [0.75 ("Output") 0.0 ("Output")] -> w2698
              tunnel: [0.75 ("Output") -0.75 ("Output")] -> w2697
              tunnel: [0.0 ("Output") 0.0 ("Output")] -> w2696
              tunnel: [FALSE ("Middle Thumb") FALSE ("Middle Thumb")] -> w2694
              tunnel: [0.0 ("Z") 0.0 ("Z")] -> w2693
              tunnel: [-0.3 ("Y") 0.0 ("Y")] -> w2692
              tunnel: [0.0 ("X") 0.0 ("X")] -> w2691
              tunnel: [WPI_SolenoidValue."Reverse" ("Value") WPI_SolenoidValue."Forward" ("Value")] -> w2690
              frame False {
              }
              frame True {
              }
            }
          }
        }
        n722 = call-poly <vilib>:"WPI_SolenoidSet.vi"("error in (no error)"=w2671, "Value"=w2651, "SolenoidDevRef"=w2670) -> ("error out"=w2639:errorcluster, "SolenoidDevRef"=w2640:T12)  [unwired: 7 in]
        n723 = call <vilib>:"CTRE_Phoenix_MotorControl_Set.vi"("error in (no error)"=w2663, "Output"=w2668, "Control Mode"=w2656, "PhoenixMotorControlDevRef"=w2662) -> ("error out"=w2648:errorcluster, "PhoenixMotorControlDevRef"=w2647:T7)  [unwired: 6 in]
        n724 = call <vilib>:"CTRE_Phoenix_MotorControl_Set.vi"("error in (no error)"=w2665, "Output"=w2660, "Control Mode"=w2657, "PhoenixMotorControlDevRef"=w2664) -> ()  [unwired: 6 in, 2 out]
        n725 = call <vilib>:"CTRE_Phoenix_MotorControl_Set.vi"("error in (no error)"=w2667, "Output"=w2659, "Control Mode"=w2658, "PhoenixMotorControlDevRef"=w2666) -> ("error out"=w2650:errorcluster, "PhoenixMotorControlDevRef"=w2649:T7)  [unwired: 6 in]
        n726 = call <vilib>:"CTRE_Phoenix_MotorControl_Set.vi"("error in (no error)"=w2646, "Output"=-0.55, "Control Mode"=w2644, "PhoenixMotorControlDevRef"=w2645) -> ("error out"=w2642:errorcluster, "PhoenixMotorControlDevRef"=w2641:T7)  [unwired: 6 in]
        n727 = call "Drive_Vi.vi"("Middle Thumb"=w2655, "Z"=w2654, "Y"=w2653, "X"=w2652) -> ()  [unwired: 8 in]
      }
      n728 = call <vilib>:"WPI_SwitchRefNum Registry Get.vi"("refnum name"="Orange Limit Switch") -> ("error out"=w2527:errorcluster, "SwitchDevRef"=w2526:T4)  [unwired: 9 in]
      n729 = call <vilib>:"WPI_SwitchRefNum Registry Get.vi"("refnum name"="Blue Limit Switch") -> ("error out"=w2529:errorcluster, "SwitchDevRef"=w2528:T4)  [unwired: 9 in]
      n730 = while {
        tunnel: w2519 -> [_]
        tunnel: w2518 -> [_]
        tunnel: w2529 -> [w2636]
        tunnel: w2528 -> [w2635]
        tunnel: w2527 -> [w2634]
        tunnel: w2526 -> [w2633]
        tunnel: w2525 -> [w2612]
        tunnel: w2524 -> [w2611]
        tunnel: w2523 -> [w2602]
        tunnel: w2522 -> [w2603]
        tunnel: [w2616] -> w2517
        tunnel: [w2615] -> w2516
        tunnel: [w2614] -> w2515
        tunnel: [w2613] -> w2514
        tunnel: [w2612] -> w2513
        tunnel: [w2611] -> w2512
        tunnel: w2511 -> [w2610]
        tunnel: w2510 -> [w2609]
        tunnel: [w2607] -> w2509
        tunnel: [w2606] -> w2508
        tunnel: [w2605] -> w2507
        tunnel: [w2604] -> w2506
        i -> [w2622]
        stop <- w2621 stop-if-true
        w2601 = T11 0 items=["PercentOutput"=0, "Position"=1, "Velocity"=2, "Current"=3, "Follower"=5, "MotionProfile"=6, "MotionMagic"=7, "MotionProfileArc"=10, "Disabled"=15] ("Control Mode")
        n731 = call-poly <vilib>:"WPI_SolenoidSet.vi"("error in (no error)"=w2609, "Value"=WPI_SolenoidValue."Forward", "SolenoidDevRef"=w2610) -> ("error out"=w2606:errorcluster, "SolenoidDevRef"=w2607:T12)  [unwired: 7 in]
        n732 = call <vilib>:"WPI_SwitchGetLimitValue.vi"("error in (no error)"=w2634, "SwitchDevRef"=w2633) -> ("error out"=w2613:errorcluster, "Switch Pressed"=w2632:bool, "SwitchDevRef"=w2614:T4)  [unwired: 7 in]
        "Orange Limit Pressed 5" <- w2632
        n733 = call <vilib>:"WPI_SwitchGetLimitValue.vi"("error in (no error)"=w2636, "SwitchDevRef"=w2635) -> ("error out"=w2615:errorcluster, "Switch Pressed"=w2631:bool, "SwitchDevRef"=w2616:T4)  [unwired: 7 in]
        "Blue Limit Pressed 5" <- w2631
        n734 = call-poly <vilib>:"NT Read Value.vi"("Default Value"=0.0, "Name"="/limelight-drtrain/ty") -> ("Numeric"=w2626:dbl)  [unwired: 8 in, 1 out]
        "Ty 5" <- w2626
        n735 = Greater?(x=w2622, y=5) -> (0:w2621:bool)
        n736 = call "Turret_Aim.vi"("View Button"=FALSE ("Driver Right Thumb"), "Left Trigger"=2.0, "Orange Limit Pressed"=w2631, "Blue Limit Pressed"=w2632, "Right Bumper"=FALSE, "Left Bumper"=FALSE) -> ()  [unwired: 6 in]
        n737 = call "Shooter_Equation.vi"("Right Trigger"=2.0, "Ty"=w2626) -> ()  [unwired: 10 in]
        n738 = Wait (ms)(milliseconds to wait=u32 100) -> ()  [unwired: 1 out]
        n739 = call "Drive_Vi.vi"("Middle Thumb"=FALSE, "Z"=0.0, "Y"=0.15, "X"=0.0) -> ()  [unwired: 8 in]
        n740 = call <vilib>:"CTRE_Phoenix_MotorControl_Set.vi"("error in (no error)"=w2602, "Output"=0.0, "Control Mode"=w2601, "PhoenixMotorControlDevRef"=w2603) -> ("error out"=w2604:errorcluster, "PhoenixMotorControlDevRef"=w2605:T7)  [unwired: 6 in]
      }
      n741 = while {
        tunnel: w2516 -> [w2597]
        tunnel: w2517 -> [w2596]
        tunnel: w2514 -> [w2595]
        tunnel: w2513 -> [w2582]
        tunnel: w2512 -> [w2581]
        tunnel: w2506 -> [w2580]
        tunnel: w2507 -> [w2579]
        tunnel: w2515 -> [w2570]
        tunnel: w2509 -> [w2569]
        tunnel: w2508 -> [w2568]
        tunnel: [w2566] -> w2505
        tunnel: [w2565] -> w2504
        tunnel: [w2564] -> w2503
        tunnel: [w2563] -> w2502
        i -> [w2584]
        stop <- w2583 stop-if-true
        w2577 = T11 0 items=["PercentOutput"=0, "Position"=1, "Velocity"=2, "Current"=3, "Follower"=5, "MotionProfile"=6, "MotionMagic"=7, "MotionProfileArc"=10, "Disabled"=15] ("Control Mode")
        w2578 = T11 0 items=["PercentOutput"=0, "Position"=1, "Velocity"=2, "Current"=3, "Follower"=5, "MotionProfile"=6, "MotionMagic"=7, "MotionProfileArc"=10, "Disabled"=15] ("Control Mode")
        n742 = call-poly <vilib>:"WPI_SolenoidSet.vi"("error in (no error)"=w2568, "Value"=WPI_SolenoidValue."Off", "SolenoidDevRef"=w2569) -> ()  [unwired: 7 in, 2 out]
        n743 = call <vilib>:"WPI_SwitchGetLimitValue.vi"("error in (no error)"=w2595, "SwitchDevRef"=w2570) -> ("Switch Pressed"=w2594:bool)  [unwired: 7 in, 2 out]
        "Orange Limit Pressed 6" <- w2594
        n744 = call <vilib>:"WPI_SwitchGetLimitValue.vi"("error in (no error)"=w2597, "SwitchDevRef"=w2596) -> ("Switch Pressed"=w2593:bool)  [unwired: 7 in, 2 out]
        "Blue Limit Pressed 6" <- w2593
        n745 = call-poly <vilib>:"NT Read Value.vi"("Default Value"=0.0, "Name"="/limelight-drtrain/ty") -> ("Numeric"=w2588:dbl)  [unwired: 8 in, 1 out]
        "Ty 6" <- w2588
        n746 = Greater?(x=w2584, y=50) -> (0:w2583:bool)
        n747 = call "Turret_Aim.vi"("View Button"=FALSE ("Driver Right Thumb"), "Left Trigger"=2.0, "Orange Limit Pressed"=w2593, "Blue Limit Pressed"=w2594, "Right Bumper"=FALSE, "Left Bumper"=FALSE) -> ()  [unwired: 6 in]
        n748 = call "Shooter_Equation.vi"("Right Trigger"=2.0, "Ty"=w2588) -> ()  [unwired: 10 in]
        n749 = Wait (ms)(milliseconds to wait=u32 100) -> ()  [unwired: 1 out]
        n750 = call "Drive_Vi.vi"("Middle Thumb"=FALSE, "Z"=0.0, "Y"=0.15, "X"=0.0) -> ()  [unwired: 8 in]
        n751 = call <vilib>:"CTRE_Phoenix_MotorControl_Set.vi"("error in (no error)"=w2580, "Output"=0.35, "Control Mode"=w2577, "PhoenixMotorControlDevRef"=w2579) -> ("error out"=w2566:errorcluster, "PhoenixMotorControlDevRef"=w2565:T7)  [unwired: 6 in]
        n752 = call <vilib>:"CTRE_Phoenix_MotorControl_Set.vi"("error in (no error)"=w2582, "Output"=-0.35, "Control Mode"=w2578, "PhoenixMotorControlDevRef"=w2581) -> ("error out"=w2563:errorcluster, "PhoenixMotorControlDevRef"=w2564:T7)  [unwired: 6 in]
      }
      n753 = while {
        tunnel: w2505 -> [w2558]
        tunnel: w2504 -> [w2557]
        tunnel: w2503 -> [w2556]
        tunnel: w2502 -> [w2555]
        i -> [w2553]
        stop <- w2552 stop-if-true
        w2561 = T11 0 items=["PercentOutput"=0, "Position"=1, "Velocity"=2, "Current"=3, "Follower"=5, "MotionProfile"=6, "MotionMagic"=7, "MotionProfileArc"=10, "Disabled"=15] ("Control Mode")
        w2562 = T11 0 items=["PercentOutput"=0, "Position"=1, "Velocity"=2, "Current"=3, "Follower"=5, "MotionProfile"=6, "MotionMagic"=7, "MotionProfileArc"=10, "Disabled"=15] ("Control Mode")
        n754 = call <vilib>:"CTRE_Phoenix_MotorControl_Set.vi"("error in (no error)"=w2558, "Output"=0.0, "Control Mode"=w2561, "PhoenixMotorControlDevRef"=w2557) -> ()  [unwired: 6 in, 2 out]
        n755 = call <vilib>:"CTRE_Phoenix_MotorControl_Set.vi"("error in (no error)"=w2555, "Output"=0.0, "Control Mode"=w2562, "PhoenixMotorControlDevRef"=w2556) -> ()  [unwired: 6 in, 2 out]
        n756 = Greater?(x=w2553, y=50) -> (0:w2552:bool)
        n757 = Wait (ms)(milliseconds to wait=u32 100) -> ()  [unwired: 1 out]
      }
    }
    frame "Human Player" {
      # "Pigeon Set"
      n758 = while {
        i -> [w2990]
        stop <- w2991 stop-if-true
        n759 = Wait (ms)(milliseconds to wait=u32 20) -> ()  [unwired: 1 out]
        n760 = Greater?(x=w2990, y=2) -> (0:w2991:bool)
        n761 = call "Drive_Vi.vi"("Middle Thumb"=TRUE, "Z"=0.0, "Y"=0.0, "X"=0.0) -> ()  [unwired: 8 in]
      }
      n762 = call <vilib>:"WPI_SwitchRefNum Registry Get.vi"("refnum name"="Intake Sensor") -> ("error out"=w2769:errorcluster, "SwitchDevRef"=w2768:T4)  [unwired: 9 in]
      n763 = call <vilib>:"CTRE_Phoenix_MotorControl_RefNumRegistryGet.vi"("refnum name"="Intake") -> ("error out"=w2763:errorcluster, "PhoenixMotorControlDevRef"=w2762:T7)  [unwired: 9 in]
      n764 = call <vilib>:"CTRE_Phoenix_MotorControl_RefNumRegistryGet.vi"("refnum name"="Intake Actuate") -> ("error out"=w2738:errorcluster, "PhoenixMotorControlDevRef"=w2737:T7)  [unwired: 9 in]
      n765 = call <vilib>:"CTRE_Phoenix_MotorControl_RefNumRegistryGet.vi"("refnum name"="Reject") -> ("error out"=w2765:errorcluster, "PhoenixMotorControlDevRef"=w2764:T7)  [unwired: 9 in]
      n766 = call "Limit_Switches.vi"() -> ()  [unwired: 10 in, 2 out]
      n767 = call <vilib>:"CTRE_Phoenix_MotorControl_RefNumRegistryGet.vi"("refnum name"="Elevate") -> ("error out"=w2767:errorcluster, "PhoenixMotorControlDevRef"=w2766:T7)  [unwired: 9 in]
      n768 = call <vilib>:"WPI_SwitchRefNum Registry Get.vi"("refnum name"="Elevate Sensor") -> ("error out"=w2771:errorcluster, "SwitchDevRef"=w2770:T4)  [unwired: 9 in]
      n769 = call <vilib>:"CTRE_Phoenix_MotorControl_RefNumRegistryGet.vi"("refnum name"="Shoot") -> ("error out"=w2751:errorcluster, "PhoenixMotorControlDevRef"=w2750:T7)  [unwired: 9 in]
      n770 = while {
        tunnel: w2771 -> [w2949]
        tunnel: w2770 -> [w2948]
        tunnel: w2769 -> [w2947]
        tunnel: w2768 -> [w2946]
        tunnel: w2767 -> [w2943]
        tunnel: w2766 -> [w2942]
        tunnel: w2765 -> [w2941]
        tunnel: w2764 -> [w2940]
        tunnel: w2763 -> [w2939]
        tunnel: w2762 -> [w2938]
        tunnel: [w2927] -> w2755
        tunnel: [w2926] -> w2754
        tunnel: [w2925] -> w2753
        tunnel: [w2924] -> w2752
        tunnel: w2751 -> [w2923]
        tunnel: w2750 -> [w2922]
        tunnel: [w2919] -> w2749
        tunnel: [w2918] -> w2748
        tunnel: w2738 -> [w2917]
        tunnel: w2737 -> [w2916]
        tunnel: [w2913] -> w2736
        tunnel: [w2912] -> w2735
        i -> [w2952]
        stop <- w2953 stop-if-true
        w2915 = T11 0 items=["PercentOutput"=0, "Position"=1, "Velocity"=2, "Current"=3, "Follower"=5, "MotionProfile"=6, "MotionMagic"=7, "MotionProfileArc"=10, "Disabled"=15] ("Control Mode")
        w2921 = T11 0 items=["PercentOutput"=0, "Position"=1, "Velocity"=2, "Current"=3, "Follower"=5, "MotionProfile"=6, "MotionMagic"=7, "MotionProfileArc"=10, "Disabled"=15] ("Control Mode")
        w2932 = T11 0 items=["PercentOutput"=0, "Position"=1, "Velocity"=2, "Current"=3, "Follower"=5, "MotionProfile"=6, "MotionMagic"=7, "MotionProfileArc"=10, "Disabled"=15] ("Control Mode")
        w2933 = T11 0 items=["PercentOutput"=0, "Position"=1, "Velocity"=2, "Current"=3, "Follower"=5, "MotionProfile"=6, "MotionMagic"=7, "MotionProfileArc"=10, "Disabled"=15] ("Control Mode")
        w2934 = T11 0 items=["PercentOutput"=0, "Position"=1, "Velocity"=2, "Current"=3, "Follower"=5, "MotionProfile"=6, "MotionMagic"=7, "MotionProfileArc"=10, "Disabled"=15] ("Control Mode")
        n771 = call <vilib>:"CTRE_Phoenix_MotorControl_Set.vi"("error in (no error)"=w2917, "Output"=-0.2, "Control Mode"=w2915, "PhoenixMotorControlDevRef"=w2916) -> ("error out"=w2912:errorcluster, "PhoenixMotorControlDevRef"=w2913:T7)  [unwired: 6 in]
        n772 = global write "AutonBoolean.vi" "Boolean"(TRUE ("Boolean")) -> ()
        n773 = call <vilib>:"WPI_SwitchGetLimitValue.vi"("error in (no error)"=w2947, "SwitchDevRef"=w2946) -> ("Switch Pressed"=w2950:bool)  [unwired: 7 in, 2 out]
        n774 = call <vilib>:"WPI_SwitchGetLimitValue.vi"("error in (no error)"=w2949, "SwitchDevRef"=w2948) -> ("Switch Pressed"=w2951:bool)  [unwired: 7 in, 2 out]
        n775 = Greater?(x=w2952, y=20) -> (0:w2953:bool)
        n776 = Not(x=w2950) -> (.not. x?=w2937:bool)
        "Intake 13" <- w2937
        n777 = Not(x=w2951) -> (.not. x?=w2945:bool)
        "Elevate 13" <- w2945
        n778 = Wait (ms)(milliseconds to wait=u32 100) -> ()  [unwired: 1 out]
        n779 = case shown="True" w2945 {
          tunnel: [0.8 ("Output") w2970] -> w2944
          tunnel: w2937 -> [_ w2967]
          tunnel: [0.75 ("Output") w2969] -> w2936
          tunnel: [-0.1 ("Output") w2968] -> w2935
          tunnel: [FALSE ("Middle Thumb") w2966] -> w2931
          tunnel: [0.0 ("Z") w2965] -> w2930
          tunnel: [0.0 ("Y") w2964] -> w2929
          tunnel: [0.0 ("X") w2963] -> w2928
          frame False {
          }
          frame True {
            n780 = case shown="False" w2967 {
              tunnel: [1.0 ("Output") 0.0 ("Output")] -> w2970
              tunnel: [0.0 ("Output") 0.0 ("Output")] -> w2969
              tunnel: [0.0 ("Output") 0.0 ("Output")] -> w2968
              tunnel: [FALSE ("Middle Thumb") FALSE ("Middle Thumb")] -> w2966
              tunnel: [0.0 ("Z") 0.0 ("Z")] -> w2965
              tunnel: [-0.3 ("Y") 0.0 ("Y")] -> w2964
              tunnel: [0.0 ("X") 0.0 ("X")] -> w2963
              frame False {
              }
              frame True {
              }
            }
          }
        }
        n781 = call <vilib>:"CTRE_Phoenix_MotorControl_Set.vi"("error in (no error)"=w2939, "Output"=w2944, "Control Mode"=w2932, "PhoenixMotorControlDevRef"=w2938) -> ("error out"=w2925:errorcluster, "PhoenixMotorControlDevRef"=w2924:T7)  [unwired: 6 in]
        n782 = call <vilib>:"CTRE_Phoenix_MotorControl_Set.vi"("error in (no error)"=w2941, "Output"=w2936, "Control Mode"=w2933, "PhoenixMotorControlDevRef"=w2940) -> ()  [unwired: 6 in, 2 out]
        n783 = call <vilib>:"CTRE_Phoenix_MotorControl_Set.vi"("error in (no error)"=w2943, "Output"=w2935, "Control Mode"=w2934, "PhoenixMotorControlDevRef"=w2942) -> ("error out"=w2927:errorcluster, "PhoenixMotorControlDevRef"=w2926:T7)  [unwired: 6 in]
        n784 = call <vilib>:"CTRE_Phoenix_MotorControl_Set.vi"("error in (no error)"=w2923, "Output"=0.0, "Control Mode"=w2921, "PhoenixMotorControlDevRef"=w2922) -> ("error out"=w2919:errorcluster, "PhoenixMotorControlDevRef"=w2918:T7)  [unwired: 6 in]
        n785 = call "Drive_Vi.vi"("Middle Thumb"=w2931, "Z"=w2930, "Y"=w2929, "X"=w2928) -> ()  [unwired: 8 in]
      }
      n786 = call <vilib>:"WPI_SwitchRefNum Registry Get.vi"("refnum name"="Orange Limit Switch") -> ("error out"=w2757:errorcluster, "SwitchDevRef"=w2756:T4)  [unwired: 9 in]
      n787 = call <vilib>:"WPI_SwitchRefNum Registry Get.vi"("refnum name"="Blue Limit Switch") -> ("error out"=w2759:errorcluster, "SwitchDevRef"=w2758:T4)  [unwired: 9 in]
      n788 = while {
        tunnel: w2749 -> [_]
        tunnel: w2748 -> [_]
        tunnel: w2759 -> [w2908]
        tunnel: w2758 -> [w2907]
        tunnel: w2757 -> [w2906]
        tunnel: w2756 -> [w2905]
        tunnel: w2755 -> [w2885]
        tunnel: w2754 -> [w2884]
        tunnel: w2753 -> [w2880]
        tunnel: w2752 -> [w2881]
        tunnel: [w2889] -> w2747
        tunnel: [w2888] -> w2746
        tunnel: [w2887] -> w2745
        tunnel: [w2886] -> w2744
        tunnel: [w2885] -> w2743
        tunnel: [w2884] -> w2742
        tunnel: [w2883] -> w2741
        tunnel: [w2882] -> w2740
        tunnel: w2736 -> [w2875]
        tunnel: w2735 -> [w2874]
        i -> [w2895]
        stop <- w2894 stop-if-true
        w2877 = T11 0 items=["PercentOutput"=0, "Position"=1, "Velocity"=2, "Current"=3, "Follower"=5, "MotionProfile"=6, "MotionMagic"=7, "MotionProfileArc"=10, "Disabled"=15] ("Control Mode")
        w2879 = T11 0 items=["PercentOutput"=0, "Position"=1, "Velocity"=2, "Current"=3, "Follower"=5, "MotionProfile"=6, "MotionMagic"=7, "MotionProfileArc"=10, "Disabled"=15] ("Control Mode")
        n789 = call <vilib>:"CTRE_Phoenix_MotorControl_Set.vi"("error in (no error)"=w2874, "Output"=0.0, "Control Mode"=w2877, "PhoenixMotorControlDevRef"=w2875) -> ()  [unwired: 6 in, 2 out]
        n790 = call <vilib>:"WPI_SwitchGetLimitValue.vi"("error in (no error)"=w2906, "SwitchDevRef"=w2905) -> ("error out"=w2886:errorcluster, "Switch Pressed"=w2904:bool, "SwitchDevRef"=w2887:T4)  [unwired: 7 in]
        "Orange Limit Pressed 25" <- w2904
        n791 = call <vilib>:"WPI_SwitchGetLimitValue.vi"("error in (no error)"=w2908, "SwitchDevRef"=w2907) -> ("error out"=w2888:errorcluster, "Switch Pressed"=w2903:bool, "SwitchDevRef"=w2889:T4)  [unwired: 7 in]
        "Blue Limit Pressed 25" <- w2903
        n792 = call-poly <vilib>:"NT Read Value.vi"("Default Value"=0.0, "Name"="/limelight-drtrain/ty") -> ("Numeric"=→"Ty 57":dbl)  [unwired: 8 in, 1 out]
        n793 = global write "AutonBoolean.vi" "Boolean"(FALSE ("Boolean")) -> ()
        n794 = Greater?(x=w2895, y=5) -> (0:w2894:bool)
        n795 = call "Turret_Aim.vi"("View Button"=FALSE ("Driver Right Thumb"), "Left Trigger"=2.0, "Orange Limit Pressed"=w2903, "Blue Limit Pressed"=w2904, "Right Bumper"=FALSE, "Left Bumper"=FALSE) -> ()  [unwired: 6 in]
        n796 = Wait (ms)(milliseconds to wait=u32 100) -> ()  [unwired: 1 out]
        n797 = call "Drive_Vi.vi"("Middle Thumb"=FALSE, "Z"=0.0, "Y"=0.15, "X"=0.0) -> ()  [unwired: 8 in]
        n798 = call <vilib>:"CTRE_Phoenix_MotorControl_Set.vi"("error in (no error)"=w2880, "Output"=0.0, "Control Mode"=w2879, "PhoenixMotorControlDevRef"=w2881) -> ("error out"=w2882:errorcluster, "PhoenixMotorControlDevRef"=w2883:T7)  [unwired: 6 in]
      }
      n799 = while {
        tunnel: w2746 -> [w2870]
        tunnel: w2747 -> [w2869]
        tunnel: w2744 -> [w2868]
        tunnel: w2743 -> [w2856]
        tunnel: w2742 -> [w2855]
        tunnel: w2740 -> [w2854]
        tunnel: w2741 -> [w2853]
        tunnel: w2745 -> [w2844]
        tunnel: [w2843] -> w2733
        tunnel: [w2842] -> w2734
        tunnel: [w2841] -> w2732
        tunnel: [w2840] -> w2731
        i -> [w2858]
        stop <- w2857 stop-if-true
        w2851 = T11 0 items=["PercentOutput"=0, "Position"=1, "Velocity"=2, "Current"=3, "Follower"=5, "MotionProfile"=6, "MotionMagic"=7, "MotionProfileArc"=10, "Disabled"=15] ("Control Mode")
        w2852 = T11 0 items=["PercentOutput"=0, "Position"=1, "Velocity"=2, "Current"=3, "Follower"=5, "MotionProfile"=6, "MotionMagic"=7, "MotionProfileArc"=10, "Disabled"=15] ("Control Mode")
        (unwired) 2.0 ("Right Trigger")
        n800 = call <vilib>:"WPI_SwitchGetLimitValue.vi"("error in (no error)"=w2868, "SwitchDevRef"=w2844) -> ("Switch Pressed"=w2867:bool)  [unwired: 7 in, 2 out]
        "Orange Limit Pressed 26" <- w2867
        n801 = call <vilib>:"WPI_SwitchGetLimitValue.vi"("error in (no error)"=w2870, "SwitchDevRef"=w2869) -> ("Switch Pressed"=w2866:bool)  [unwired: 7 in, 2 out]
        "Blue Limit Pressed 26" <- w2866
        n802 = call-poly <vilib>:"NT Read Value.vi"("Default Value"=0.0, "Name"="/limelight-drtrain/ty") -> ("Numeric"=→"Ty 58":dbl)  [unwired: 8 in, 1 out]
        n803 = Greater?(x=w2858, y=50) -> (0:w2857:bool)
        n804 = call "Turret_Aim.vi"("View Button"=FALSE ("Driver Right Thumb"), "Left Trigger"=2.0, "Orange Limit Pressed"=w2866, "Blue Limit Pressed"=w2867, "Right Bumper"=FALSE, "Left Bumper"=FALSE) -> ()  [unwired: 6 in]
        n805 = Wait (ms)(milliseconds to wait=u32 100) -> ()  [unwired: 1 out]
        n806 = call "Drive_Vi.vi"("Middle Thumb"=FALSE, "Z"=0.0, "Y"=0.15, "X"=0.0) -> ()  [unwired: 8 in]
        n807 = call <vilib>:"CTRE_Phoenix_MotorControl_Set.vi"("error in (no error)"=w2854, "Output"=0.35, "Control Mode"=w2851, "PhoenixMotorControlDevRef"=w2853) -> ("error out"=w2843:errorcluster, "PhoenixMotorControlDevRef"=w2842:T7)  [unwired: 6 in]
        n808 = call <vilib>:"CTRE_Phoenix_MotorControl_Set.vi"("error in (no error)"=w2856, "Output"=-0.35, "Control Mode"=w2852, "PhoenixMotorControlDevRef"=w2855) -> ("error out"=w2840:errorcluster, "PhoenixMotorControlDevRef"=w2841:T7)  [unwired: 6 in]
      }
      n809 = while {
        tunnel: w2731 -> [w2816]
        tunnel: w2732 -> [w2815]
        tunnel: w2733 -> [w2814]
        tunnel: w2734 -> [w2813]
        tunnel: [w2804] -> w2729
        tunnel: [w2803] -> w2730
        tunnel: [w2802] -> w2728
        tunnel: [w2801] -> w2727
        i -> [w2818]
        stop <- w2817 stop-if-true
        w2811 = T11 0 items=["PercentOutput"=0, "Position"=1, "Velocity"=2, "Current"=3, "Follower"=5, "MotionProfile"=6, "MotionMagic"=7, "MotionProfileArc"=10, "Disabled"=15] ("Control Mode")
        w2812 = T11 0 items=["PercentOutput"=0, "Position"=1, "Velocity"=2, "Current"=3, "Follower"=5, "MotionProfile"=6, "MotionMagic"=7, "MotionProfileArc"=10, "Disabled"=15] ("Control Mode")
        (unwired) 0.0 ("Right Trigger")
        n810 = call-poly <vilib>:"NT Read Value.vi"("Default Value"=0.0, "Name"="/limelight-drtrain/ty") -> ("Numeric"=→"Ty 59":dbl)  [unwired: 8 in, 1 out]
        n811 = Greater?(x=w2818, y=10) -> (0:w2817:bool)
        n812 = Wait (ms)(milliseconds to wait=u32 112) -> ()  [unwired: 1 out]
        n813 = call "Drive_Vi.vi"("Middle Thumb"=FALSE, "Z"=0.35, "Y"=0.0, "X"=0.0) -> ()  [unwired: 8 in]
        n814 = call <vilib>:"CTRE_Phoenix_MotorControl_Set.vi"("error in (no error)"=w2814, "Output"=0.0, "Control Mode"=w2811, "PhoenixMotorControlDevRef"=w2813) -> ("error out"=w2804:errorcluster, "PhoenixMotorControlDevRef"=w2803:T7)  [unwired: 6 in]
        n815 = call <vilib>:"CTRE_Phoenix_MotorControl_Set.vi"("error in (no error)"=w2816, "Output"=0.0, "Control Mode"=w2812, "PhoenixMotorControlDevRef"=w2815) -> ("error out"=w2801:errorcluster, "PhoenixMotorControlDevRef"=w2802:T7)  [unwired: 6 in]
      }
      n816 = while {
        tunnel: w2727 -> [w2793]
        tunnel: w2728 -> [w2792]
        tunnel: w2729 -> [w2791]
        tunnel: w2730 -> [w2790]
        tunnel: [w2781] -> w2724
        tunnel: [w2780] -> w2726
        tunnel: [w2779] -> w2725
        tunnel: [w2778] -> w2723
        i -> [w2795]
        stop <- w2794 stop-if-true
        w2788 = T11 0 items=["PercentOutput"=0, "Position"=1, "Velocity"=2, "Current"=3, "Follower"=5, "MotionProfile"=6, "MotionMagic"=7, "MotionProfileArc"=10, "Disabled"=15] ("Control Mode")
        w2789 = T11 0 items=["PercentOutput"=0, "Position"=1, "Velocity"=2, "Current"=3, "Follower"=5, "MotionProfile"=6, "MotionMagic"=7, "MotionProfileArc"=10, "Disabled"=15] ("Control Mode")
        (unwired) 0.0 ("Right Trigger")
        n817 = call-poly <vilib>:"NT Read Value.vi"("Default Value"=0.0, "Name"="/limelight-drtrain/ty") -> ("Numeric"=→"Ty 60":dbl)  [unwired: 8 in, 1 out]
        n818 = Greater?(x=w2795, y=2) -> (0:w2794:bool)
        n819 = Wait (ms)(milliseconds to wait=u32 20) -> ()  [unwired: 1 out]
        n820 = call "Drive_Vi.vi"("Middle Thumb"=TRUE, "Z"=0.0, "Y"=0.0, "X"=0.0) -> ()  [unwired: 8 in]
        n821 = call <vilib>:"CTRE_Phoenix_MotorControl_Set.vi"("error in (no error)"=w2791, "Output"=0.0, "Control Mode"=w2788, "PhoenixMotorControlDevRef"=w2790) -> ("error out"=w2781:errorcluster, "PhoenixMotorControlDevRef"=w2780:T7)  [unwired: 6 in]
        n822 = call <vilib>:"CTRE_Phoenix_MotorControl_Set.vi"("error in (no error)"=w2793, "Output"=0.0, "Control Mode"=w2789, "PhoenixMotorControlDevRef"=w2792) -> ("error out"=w2778:errorcluster, "PhoenixMotorControlDevRef"=w2779:T7)  [unwired: 6 in]
      }
      n823 = while {
        tunnel: w2724 -> [w2835]
        tunnel: w2726 -> [w2834]
        tunnel: w2725 -> [w2833]
        tunnel: w2723 -> [w2832]
        i -> [w2830]
        stop <- w2829 stop-if-true
        w2838 = T11 0 items=["PercentOutput"=0, "Position"=1, "Velocity"=2, "Current"=3, "Follower"=5, "MotionProfile"=6, "MotionMagic"=7, "MotionProfileArc"=10, "Disabled"=15] ("Control Mode")
        w2839 = T11 0 items=["PercentOutput"=0, "Position"=1, "Velocity"=2, "Current"=3, "Follower"=5, "MotionProfile"=6, "MotionMagic"=7, "MotionProfileArc"=10, "Disabled"=15] ("Control Mode")
        n824 = call <vilib>:"CTRE_Phoenix_MotorControl_Set.vi"("error in (no error)"=w2835, "Output"=0.0, "Control Mode"=w2838, "PhoenixMotorControlDevRef"=w2834) -> ()  [unwired: 6 in, 2 out]
        n825 = call <vilib>:"CTRE_Phoenix_MotorControl_Set.vi"("error in (no error)"=w2832, "Output"=0.0, "Control Mode"=w2839, "PhoenixMotorControlDevRef"=w2833) -> ()  [unwired: 6 in, 2 out]
        n826 = call "Drive_Vi.vi"("Middle Thumb"=FALSE, "Z"=0.0, "Y"=0.0, "X"=0.0) -> ()  [unwired: 8 in]
        n827 = Greater?(x=w2830, y=50) -> (0:w2829:bool)
        n828 = Wait (ms)(milliseconds to wait=u32 100) -> ()  [unwired: 1 out]
      }
    }
    frame "2 Ball" {
      # "Pigeon Set"
      n829 = while {
        i -> [w3264]
        stop <- w3265 stop-if-true
        n830 = Wait (ms)(milliseconds to wait=u32 20) -> ()  [unwired: 1 out]
        n831 = Greater?(x=w3264, y=2) -> (0:w3265:bool)
        n832 = call "Drive_Vi.vi"("Middle Thumb"=TRUE, "Z"=0.0, "Y"=0.0, "X"=0.0) -> ()  [unwired: 8 in]
      }
      n833 = call <vilib>:"WPI_SwitchRefNum Registry Get.vi"("refnum name"="Intake Sensor") -> ("error out"=w3039:errorcluster, "SwitchDevRef"=w3038:T4)  [unwired: 9 in]
      n834 = call <vilib>:"CTRE_Phoenix_MotorControl_RefNumRegistryGet.vi"("refnum name"="Intake") -> ("error out"=w3033:errorcluster, "PhoenixMotorControlDevRef"=w3032:T7)  [unwired: 9 in]
      n835 = call <vilib>:"CTRE_Phoenix_MotorControl_RefNumRegistryGet.vi"("refnum name"="Intake Actuate") -> ("error out"=w3008:errorcluster, "PhoenixMotorControlDevRef"=w3007:T7)  [unwired: 9 in]
      n836 = call <vilib>:"CTRE_Phoenix_MotorControl_RefNumRegistryGet.vi"("refnum name"="Reject") -> ("error out"=w3035:errorcluster, "PhoenixMotorControlDevRef"=w3034:T7)  [unwired: 9 in]
      n837 = call "Limit_Switches.vi"() -> ()  [unwired: 10 in, 2 out]
      n838 = call <vilib>:"CTRE_Phoenix_MotorControl_RefNumRegistryGet.vi"("refnum name"="Elevate") -> ("error out"=w3037:errorcluster, "PhoenixMotorControlDevRef"=w3036:T7)  [unwired: 9 in]
      n839 = call <vilib>:"WPI_SwitchRefNum Registry Get.vi"("refnum name"="Elevate Sensor") -> ("error out"=w3041:errorcluster, "SwitchDevRef"=w3040:T4)  [unwired: 9 in]
      n840 = call <vilib>:"CTRE_Phoenix_MotorControl_RefNumRegistryGet.vi"("refnum name"="Shoot") -> ("error out"=w3021:errorcluster, "PhoenixMotorControlDevRef"=w3020:T7)  [unwired: 9 in]
      n841 = while {
        tunnel: w3041 -> [w3223]
        tunnel: w3040 -> [w3222]
        tunnel: w3039 -> [w3221]
        tunnel: w3038 -> [w3220]
        tunnel: w3037 -> [w3217]
        tunnel: w3036 -> [w3216]
        tunnel: w3035 -> [w3215]
        tunnel: w3034 -> [w3214]
        tunnel: w3033 -> [w3213]
        tunnel: w3032 -> [w3212]
        tunnel: [w3201] -> w3025
        tunnel: [w3200] -> w3024
        tunnel: [w3199] -> w3023
        tunnel: [w3198] -> w3022
        tunnel: w3021 -> [w3197]
        tunnel: w3020 -> [w3196]
        tunnel: [w3193] -> w3019
        tunnel: [w3192] -> w3018
        tunnel: w3008 -> [w3191]
        tunnel: w3007 -> [w3190]
        tunnel: [w3187] -> w3006
        tunnel: [w3186] -> w3005
        i -> [w3226]
        stop <- w3227 stop-if-true
        w3189 = T11 0 items=["PercentOutput"=0, "Position"=1, "Velocity"=2, "Current"=3, "Follower"=5, "MotionProfile"=6, "MotionMagic"=7, "MotionProfileArc"=10, "Disabled"=15] ("Control Mode")
        w3195 = T11 0 items=["PercentOutput"=0, "Position"=1, "Velocity"=2, "Current"=3, "Follower"=5, "MotionProfile"=6, "MotionMagic"=7, "MotionProfileArc"=10, "Disabled"=15] ("Control Mode")
        w3206 = T11 0 items=["PercentOutput"=0, "Position"=1, "Velocity"=2, "Current"=3, "Follower"=5, "MotionProfile"=6, "MotionMagic"=7, "MotionProfileArc"=10, "Disabled"=15] ("Control Mode")
        w3207 = T11 0 items=["PercentOutput"=0, "Position"=1, "Velocity"=2, "Current"=3, "Follower"=5, "MotionProfile"=6, "MotionMagic"=7, "MotionProfileArc"=10, "Disabled"=15] ("Control Mode")
        w3208 = T11 0 items=["PercentOutput"=0, "Position"=1, "Velocity"=2, "Current"=3, "Follower"=5, "MotionProfile"=6, "MotionMagic"=7, "MotionProfileArc"=10, "Disabled"=15] ("Control Mode")
        n842 = call <vilib>:"CTRE_Phoenix_MotorControl_Set.vi"("error in (no error)"=w3191, "Output"=-0.2, "Control Mode"=w3189, "PhoenixMotorControlDevRef"=w3190) -> ("error out"=w3186:errorcluster, "PhoenixMotorControlDevRef"=w3187:T7)  [unwired: 6 in]
        n843 = global write "AutonBoolean.vi" "Boolean"(TRUE ("Boolean")) -> ()
        n844 = call <vilib>:"WPI_SwitchGetLimitValue.vi"("error in (no error)"=w3221, "SwitchDevRef"=w3220) -> ("Switch Pressed"=w3224:bool)  [unwired: 7 in, 2 out]
        n845 = call <vilib>:"WPI_SwitchGetLimitValue.vi"("error in (no error)"=w3223, "SwitchDevRef"=w3222) -> ("Switch Pressed"=w3225:bool)  [unwired: 7 in, 2 out]
        n846 = Greater?(x=w3226, y=20) -> (0:w3227:bool)
        n847 = Not(x=w3224) -> (.not. x?=w3211:bool)
        "Intake" <- w3211
        n848 = Not(x=w3225) -> (.not. x?=w3219:bool)
        "Elevate" <- w3219
        n849 = Wait (ms)(milliseconds to wait=u32 100) -> ()  [unwired: 1 out]
        n850 = case shown="True" w3219 {
          tunnel: [0.8 ("Output") w3244] -> w3218
          tunnel: w3211 -> [_ w3241]
          tunnel: [0.75 ("Output") w3243] -> w3210
          tunnel: [-0.1 ("Output") w3242] -> w3209
          tunnel: [FALSE ("Middle Thumb") w3240] -> w3205
          tunnel: [0.0 ("Z") w3239] -> w3204
          tunnel: [0.0 ("Y") w3238] -> w3203
          tunnel: [0.0 ("X") w3237] -> w3202
          frame False {
          }
          frame True {
            n851 = case shown="False" w3241 {
              tunnel: [1.0 ("Output") 0.0 ("Output")] -> w3244
              tunnel: [0.0 ("Output") 0.0 ("Output")] -> w3243
              tunnel: [0.0 ("Output") 0.0 ("Output")] -> w3242
              tunnel: [FALSE ("Middle Thumb") FALSE ("Middle Thumb")] -> w3240
              tunnel: [0.0 ("Z") 0.0 ("Z")] -> w3239
              tunnel: [-0.3 ("Y") 0.0 ("Y")] -> w3238
              tunnel: [0.0 ("X") 0.0 ("X")] -> w3237
              frame False {
              }
              frame True {
              }
            }
          }
        }
        n852 = call <vilib>:"CTRE_Phoenix_MotorControl_Set.vi"("error in (no error)"=w3213, "Output"=w3218, "Control Mode"=w3206, "PhoenixMotorControlDevRef"=w3212) -> ("error out"=w3199:errorcluster, "PhoenixMotorControlDevRef"=w3198:T7)  [unwired: 6 in]
        n853 = call <vilib>:"CTRE_Phoenix_MotorControl_Set.vi"("error in (no error)"=w3215, "Output"=w3210, "Control Mode"=w3207, "PhoenixMotorControlDevRef"=w3214) -> ()  [unwired: 6 in, 2 out]
        n854 = call <vilib>:"CTRE_Phoenix_MotorControl_Set.vi"("error in (no error)"=w3217, "Output"=w3209, "Control Mode"=w3208, "PhoenixMotorControlDevRef"=w3216) -> ("error out"=w3201:errorcluster, "PhoenixMotorControlDevRef"=w3200:T7)  [unwired: 6 in]
        n855 = call <vilib>:"CTRE_Phoenix_MotorControl_Set.vi"("error in (no error)"=w3197, "Output"=-0.55, "Control Mode"=w3195, "PhoenixMotorControlDevRef"=w3196) -> ("error out"=w3193:errorcluster, "PhoenixMotorControlDevRef"=w3192:T7)  [unwired: 6 in]
        n856 = call "Drive_Vi.vi"("Middle Thumb"=w3205, "Z"=w3204, "Y"=w3203, "X"=w3202) -> ()  [unwired: 8 in]
      }
      n857 = call <vilib>:"WPI_SwitchRefNum Registry Get.vi"("refnum name"="Orange Limit Switch") -> ("error out"=w3027:errorcluster, "SwitchDevRef"=w3026:T4)  [unwired: 9 in]
      n858 = call <vilib>:"WPI_SwitchRefNum Registry Get.vi"("refnum name"="Blue Limit Switch") -> ("error out"=w3029:errorcluster, "SwitchDevRef"=w3028:T4)  [unwired: 9 in]
      n859 = while {
        tunnel: w3019 -> [_]
        tunnel: w3018 -> [_]
        tunnel: w3029 -> [w3182]
        tunnel: w3028 -> [w3181]
        tunnel: w3027 -> [w3180]
        tunnel: w3026 -> [w3179]
        tunnel: w3025 -> [w3158]
        tunnel: w3024 -> [w3157]
        tunnel: w3023 -> [w3153]
        tunnel: w3022 -> [w3154]
        tunnel: [w3162] -> w3017
        tunnel: [w3161] -> w3016
        tunnel: [w3160] -> w3015
        tunnel: [w3159] -> w3014
        tunnel: [w3158] -> w3013
        tunnel: [w3157] -> w3012
        tunnel: [w3156] -> w3011
        tunnel: [w3155] -> w3010
        tunnel: w3006 -> [w3148]
        tunnel: w3005 -> [w3147]
        i -> [w3168]
        stop <- w3167 stop-if-true
        w3150 = T11 0 items=["PercentOutput"=0, "Position"=1, "Velocity"=2, "Current"=3, "Follower"=5, "MotionProfile"=6, "MotionMagic"=7, "MotionProfileArc"=10, "Disabled"=15] ("Control Mode")
        w3152 = T11 0 items=["PercentOutput"=0, "Position"=1, "Velocity"=2, "Current"=3, "Follower"=5, "MotionProfile"=6, "MotionMagic"=7, "MotionProfileArc"=10, "Disabled"=15] ("Control Mode")
        n860 = call <vilib>:"CTRE_Phoenix_MotorControl_Set.vi"("error in (no error)"=w3147, "Output"=0.0, "Control Mode"=w3150, "PhoenixMotorControlDevRef"=w3148) -> ()  [unwired: 6 in, 2 out]
        n861 = call <vilib>:"WPI_SwitchGetLimitValue.vi"("error in (no error)"=w3180, "SwitchDevRef"=w3179) -> ("error out"=w3159:errorcluster, "Switch Pressed"=w3178:bool, "SwitchDevRef"=w3160:T4)  [unwired: 7 in]
        "Orange Limit Pressed" <- w3178
        n862 = call <vilib>:"WPI_SwitchGetLimitValue.vi"("error in (no error)"=w3182, "SwitchDevRef"=w3181) -> ("error out"=w3161:errorcluster, "Switch Pressed"=w3177:bool, "SwitchDevRef"=w3162:T4)  [unwired: 7 in]
        "Blue Limit Pressed" <- w3177
        n863 = call-poly <vilib>:"NT Read Value.vi"("Default Value"=0.0, "Name"="/limelight-drtrain/ty") -> ("Numeric"=w3172:dbl)  [unwired: 8 in, 1 out]
        "Ty" <- w3172
        n864 = global write "AutonBoolean.vi" "Boolean"(FALSE ("Boolean")) -> ()
        n865 = Greater?(x=w3168, y=5) -> (0:w3167:bool)
        n866 = call "Turret_Aim.vi"("View Button"=FALSE ("Driver Right Thumb"), "Left Trigger"=2.0, "Orange Limit Pressed"=w3177, "Blue Limit Pressed"=w3178, "Right Bumper"=FALSE, "Left Bumper"=FALSE) -> ()  [unwired: 6 in]
        n867 = call "Shooter_Equation.vi"("Right Trigger"=2.0, "Ty"=w3172) -> ()  [unwired: 10 in]
        n868 = Wait (ms)(milliseconds to wait=u32 100) -> ()  [unwired: 1 out]
        n869 = call "Drive_Vi.vi"("Middle Thumb"=FALSE, "Z"=0.0, "Y"=0.15, "X"=0.0) -> ()  [unwired: 8 in]
        n870 = call <vilib>:"CTRE_Phoenix_MotorControl_Set.vi"("error in (no error)"=w3153, "Output"=0.0, "Control Mode"=w3152, "PhoenixMotorControlDevRef"=w3154) -> ("error out"=w3155:errorcluster, "PhoenixMotorControlDevRef"=w3156:T7)  [unwired: 6 in]
      }
      n871 = while {
        tunnel: w3016 -> [w3143]
        tunnel: w3017 -> [w3142]
        tunnel: w3014 -> [w3141]
        tunnel: w3013 -> [w3128]
        tunnel: w3012 -> [w3127]
        tunnel: w3010 -> [w3126]
        tunnel: w3011 -> [w3125]
        tunnel: w3015 -> [w3116]
        tunnel: [w3115] -> w3003
        tunnel: [w3114] -> w3004
        tunnel: [w3113] -> w3002
        tunnel: [w3112] -> w3001
        i -> [w3130]
        stop <- w3129 stop-if-true
        w3123 = T11 0 items=["PercentOutput"=0, "Position"=1, "Velocity"=2, "Current"=3, "Follower"=5, "MotionProfile"=6, "MotionMagic"=7, "MotionProfileArc"=10, "Disabled"=15] ("Control Mode")
        w3124 = T11 0 items=["PercentOutput"=0, "Position"=1, "Velocity"=2, "Current"=3, "Follower"=5, "MotionProfile"=6, "MotionMagic"=7, "MotionProfileArc"=10, "Disabled"=15] ("Control Mode")
        n872 = call <vilib>:"WPI_SwitchGetLimitValue.vi"("error in (no error)"=w3141, "SwitchDevRef"=w3116) -> ("Switch Pressed"=w3140:bool)  [unwired: 7 in, 2 out]
        "Orange Limit Pressed 2" <- w3140
        n873 = call <vilib>:"WPI_SwitchGetLimitValue.vi"("error in (no error)"=w3143, "SwitchDevRef"=w3142) -> ("Switch Pressed"=w3139:bool)  [unwired: 7 in, 2 out]
        "Blue Limit Pressed 2" <- w3139
        n874 = call-poly <vilib>:"NT Read Value.vi"("Default Value"=0.0, "Name"="/limelight-drtrain/ty") -> ("Numeric"=w3134:dbl)  [unwired: 8 in, 1 out]
        "Ty 2" <- w3134
        n875 = Greater?(x=w3130, y=50) -> (0:w3129:bool)
        n876 = call "Turret_Aim.vi"("View Button"=FALSE ("Driver Right Thumb"), "Left Trigger"=2.0, "Orange Limit Pressed"=w3139, "Blue Limit Pressed"=w3140, "Right Bumper"=FALSE, "Left Bumper"=FALSE) -> ()  [unwired: 6 in]
        n877 = call "Shooter_Equation.vi"("Right Trigger"=2.0, "Ty"=w3134) -> ()  [unwired: 10 in]
        n878 = Wait (ms)(milliseconds to wait=u32 100) -> ()  [unwired: 1 out]
        n879 = call "Drive_Vi.vi"("Middle Thumb"=FALSE, "Z"=0.0, "Y"=0.15, "X"=0.0) -> ()  [unwired: 8 in]
        n880 = call <vilib>:"CTRE_Phoenix_MotorControl_Set.vi"("error in (no error)"=w3126, "Output"=0.35, "Control Mode"=w3123, "PhoenixMotorControlDevRef"=w3125) -> ("error out"=w3115:errorcluster, "PhoenixMotorControlDevRef"=w3114:T7)  [unwired: 6 in]
        n881 = call <vilib>:"CTRE_Phoenix_MotorControl_Set.vi"("error in (no error)"=w3128, "Output"=-0.35, "Control Mode"=w3124, "PhoenixMotorControlDevRef"=w3127) -> ("error out"=w3112:errorcluster, "PhoenixMotorControlDevRef"=w3113:T7)  [unwired: 6 in]
      }
      n882 = while {
        tunnel: w3001 -> [w3087]
        tunnel: w3002 -> [w3086]
        tunnel: w3003 -> [w3085]
        tunnel: w3004 -> [w3084]
        tunnel: [w3075] -> w2999
        tunnel: [w3074] -> w3000
        tunnel: [w3073] -> w2998
        tunnel: [w3072] -> w2997
        i -> [w3089]
        stop <- w3088 stop-if-true
        w3082 = T11 0 items=["PercentOutput"=0, "Position"=1, "Velocity"=2, "Current"=3, "Follower"=5, "MotionProfile"=6, "MotionMagic"=7, "MotionProfileArc"=10, "Disabled"=15] ("Control Mode")
        w3083 = T11 0 items=["PercentOutput"=0, "Position"=1, "Velocity"=2, "Current"=3, "Follower"=5, "MotionProfile"=6, "MotionMagic"=7, "MotionProfileArc"=10, "Disabled"=15] ("Control Mode")
        n883 = call-poly <vilib>:"NT Read Value.vi"("Default Value"=0.0, "Name"="/limelight-drtrain/ty") -> ("Numeric"=w3093:dbl)  [unwired: 8 in, 1 out]
        "Ty 23" <- w3093
        n884 = Greater?(x=w3089, y=10) -> (0:w3088:bool)
        n885 = call "Shooter_Equation.vi"("Right Trigger"=0.0, "Ty"=w3093) -> ()  [unwired: 10 in]
        n886 = Wait (ms)(milliseconds to wait=u32 112) -> ()  [unwired: 1 out]
        n887 = call "Drive_Vi.vi"("Middle Thumb"=FALSE, "Z"=0.35, "Y"=0.0, "X"=0.0) -> ()  [unwired: 8 in]
        n888 = call <vilib>:"CTRE_Phoenix_MotorControl_Set.vi"("error in (no error)"=w3085, "Output"=0.35, "Control Mode"=w3082, "PhoenixMotorControlDevRef"=w3084) -> ("error out"=w3075:errorcluster, "PhoenixMotorControlDevRef"=w3074:T7)  [unwired: 6 in]
        n889 = call <vilib>:"CTRE_Phoenix_MotorControl_Set.vi"("error in (no error)"=w3087, "Output"=-0.35, "Control Mode"=w3083, "PhoenixMotorControlDevRef"=w3086) -> ("error out"=w3072:errorcluster, "PhoenixMotorControlDevRef"=w3073:T7)  [unwired: 6 in]
      }
      n890 = while {
        tunnel: w2997 -> [w3063]
        tunnel: w2998 -> [w3062]
        tunnel: w2999 -> [w3061]
        tunnel: w3000 -> [w3060]
        tunnel: [w3051] -> w2994
        tunnel: [w3050] -> w2996
        tunnel: [w3049] -> w2995
        tunnel: [w3048] -> w2993
        i -> [w3065]
        stop <- w3064 stop-if-true
        w3058 = T11 0 items=["PercentOutput"=0, "Position"=1, "Velocity"=2, "Current"=3, "Follower"=5, "MotionProfile"=6, "MotionMagic"=7, "MotionProfileArc"=10, "Disabled"=15] ("Control Mode")
        w3059 = T11 0 items=["PercentOutput"=0, "Position"=1, "Velocity"=2, "Current"=3, "Follower"=5, "MotionProfile"=6, "MotionMagic"=7, "MotionProfileArc"=10, "Disabled"=15] ("Control Mode")
        n891 = call-poly <vilib>:"NT Read Value.vi"("Default Value"=0.0, "Name"="/limelight-drtrain/ty") -> ("Numeric"=w3069:dbl)  [unwired: 8 in, 1 out]
        "Ty 24" <- w3069
        n892 = Greater?(x=w3065, y=2) -> (0:w3064:bool)
        n893 = call "Shooter_Equation.vi"("Right Trigger"=0.0, "Ty"=w3069) -> ()  [unwired: 10 in]
        n894 = Wait (ms)(milliseconds to wait=u32 20) -> ()  [unwired: 1 out]
        n895 = call "Drive_Vi.vi"("Middle Thumb"=TRUE, "Z"=0.0, "Y"=0.0, "X"=0.0) -> ()  [unwired: 8 in]
        n896 = call <vilib>:"CTRE_Phoenix_MotorControl_Set.vi"("error in (no error)"=w3061, "Output"=0.35, "Control Mode"=w3058, "PhoenixMotorControlDevRef"=w3060) -> ("error out"=w3051:errorcluster, "PhoenixMotorControlDevRef"=w3050:T7)  [unwired: 6 in]
        n897 = call <vilib>:"CTRE_Phoenix_MotorControl_Set.vi"("error in (no error)"=w3063, "Output"=-0.35, "Control Mode"=w3059, "PhoenixMotorControlDevRef"=w3062) -> ("error out"=w3048:errorcluster, "PhoenixMotorControlDevRef"=w3049:T7)  [unwired: 6 in]
      }
      n898 = while {
        tunnel: w2994 -> [w3107]
        tunnel: w2996 -> [w3106]
        tunnel: w2995 -> [w3105]
        tunnel: w2993 -> [w3104]
        i -> [w3102]
        stop <- w3101 stop-if-true
        w3110 = T11 0 items=["PercentOutput"=0, "Position"=1, "Velocity"=2, "Current"=3, "Follower"=5, "MotionProfile"=6, "MotionMagic"=7, "MotionProfileArc"=10, "Disabled"=15] ("Control Mode")
        w3111 = T11 0 items=["PercentOutput"=0, "Position"=1, "Velocity"=2, "Current"=3, "Follower"=5, "MotionProfile"=6, "MotionMagic"=7, "MotionProfileArc"=10, "Disabled"=15] ("Control Mode")
        n899 = call <vilib>:"CTRE_Phoenix_MotorControl_Set.vi"("error in (no error)"=w3107, "Output"=0.0, "Control Mode"=w3110, "PhoenixMotorControlDevRef"=w3106) -> ()  [unwired: 6 in, 2 out]
        n900 = call <vilib>:"CTRE_Phoenix_MotorControl_Set.vi"("error in (no error)"=w3104, "Output"=0.0, "Control Mode"=w3111, "PhoenixMotorControlDevRef"=w3105) -> ()  [unwired: 6 in, 2 out]
        n901 = call "Drive_Vi.vi"("Middle Thumb"=FALSE, "Z"=0.0, "Y"=0.0, "X"=0.0) -> ()  [unwired: 8 in]
        n902 = Greater?(x=w3102, y=50) -> (0:w3101:bool)
        n903 = Wait (ms)(milliseconds to wait=u32 100) -> ()  [unwired: 1 out]
      }
    }
    frame "Drive Test" {
      # "Get limelight position and shooter started up"
      # "Driving backwards, put arms down and running intake to get ball"
      n904 = call <vilib>:"CTRE_Phoenix_MotorControl_RefNumRegistryGet.vi"("refnum name"="Intake") -> ("error out"=w3268:errorcluster, "PhoenixMotorControlDevRef"=w3270:T7)  [unwired: 9 in]
      n905 = while {
        tunnel: [w3277] -> w3269
        tunnel: w3270 -> [w3277]
        tunnel: [w3276] -> w3267
        tunnel: w3268 -> [w3276]
        i -> [w3283]
        stop <- w3284 stop-if-true
        n906 = Wait (ms)(milliseconds to wait=u32 20) -> ()  [unwired: 1 out]
        n907 = Greater?(x=w3283, y=2) -> (0:w3284:bool)
        n908 = call "Drive_Vi.vi"("Middle Thumb"=TRUE, "Z"=0.0, "Y"=0.0, "X"=0.0) -> ()  [unwired: 8 in]
      }
      n909 = while {
        tunnel: w3269 -> [w3317]
        tunnel: w3267 -> [w3316]
        tunnel: [w3315] -> w3274
        tunnel: [w3314] -> w3273
        i -> [w3324]
        stop <- w3323 stop-if-true
        w3313 = T11 0 items=["PercentOutput"=0, "Position"=1, "Velocity"=2, "Current"=3, "Follower"=5, "MotionProfile"=6, "MotionMagic"=7, "MotionProfileArc"=10, "Disabled"=15] ("Control Mode")
        # "-0.186"
        # "-0.944"
        # ".135"
        n910 = call "Drive_Vi.vi"("Middle Thumb"=FALSE, "Z"=0.0, "Y"=-0.5, "X"=0.0) -> ()  [unwired: 8 in]
        n911 = call <vilib>:"CTRE_Phoenix_MotorControl_Set.vi"("error in (no error)"=w3316, "Output"=0.0, "Control Mode"=w3313, "PhoenixMotorControlDevRef"=w3317) -> ("error out"=w3314:errorcluster, "PhoenixMotorControlDevRef"=w3315:T7)  [unwired: 6 in]
        n912 = Greater?(x=w3324, y=20) -> (0:w3323:bool)
        n913 = Wait (ms)(milliseconds to wait=u32 100) -> ()  [unwired: 1 out]
      }
      n914 = while {
        tunnel: w3274 -> [w3303]
        tunnel: w3273 -> [w3302]
        tunnel: [w3301] -> w3272
        tunnel: [w3300] -> w3271
        i -> [w3310]
        stop <- w3309 stop-if-true
        w3299 = T11 0 items=["PercentOutput"=0, "Position"=1, "Velocity"=2, "Current"=3, "Follower"=5, "MotionProfile"=6, "MotionMagic"=7, "MotionProfileArc"=10, "Disabled"=15] ("Control Mode")
        # "-0.186"
        # "-0.944"
        # ".135"
        n915 = call "Drive_Vi.vi"("Middle Thumb"=FALSE, "Z"=0.0, "Y"=0.15, "X"=0.0) -> ()  [unwired: 8 in]
        n916 = Greater?(x=w3310, y=5) -> (0:w3309:bool)
        n917 = call <vilib>:"CTRE_Phoenix_MotorControl_Set.vi"("error in (no error)"=w3302, "Output"=0.0, "Control Mode"=w3299, "PhoenixMotorControlDevRef"=w3303) -> ("error out"=w3300:errorcluster, "PhoenixMotorControlDevRef"=w3301:T7)  [unwired: 6 in]
        n918 = Wait (ms)(milliseconds to wait=u32 100) -> ()  [unwired: 1 out]
      }
      n919 = while {
        tunnel: w3272 -> [w3289]
        tunnel: w3271 -> [w3288]
        i -> [w3296]
        stop <- w3295 stop-if-true
        w3287 = T11 0 items=["PercentOutput"=0, "Position"=1, "Velocity"=2, "Current"=3, "Follower"=5, "MotionProfile"=6, "MotionMagic"=7, "MotionProfileArc"=10, "Disabled"=15] ("Control Mode")
        # "-0.186"
        # "-0.944"
        # ".135"
        n920 = call "Drive_Vi.vi"("Middle Thumb"=FALSE, "Z"=0.0, "Y"=0.0, "X"=0.0) -> ()  [unwired: 8 in]
        n921 = Greater?(x=w3296, y=20) -> (0:w3295:bool)
        n922 = call <vilib>:"CTRE_Phoenix_MotorControl_Set.vi"("error in (no error)"=w3288, "Output"=0.0, "Control Mode"=w3287, "PhoenixMotorControlDevRef"=w3289) -> ()  [unwired: 6 in, 2 out]
        n923 = Wait (ms)(milliseconds to wait=u32 100) -> ()  [unwired: 1 out]
      }
    }
    frame "4 Ball" {
      # "Pigeon Set"
      n924 = while {
        i -> [w3709]
        stop <- w3710 stop-if-true
        n925 = Wait (ms)(milliseconds to wait=u32 20) -> ()  [unwired: 1 out]
        n926 = Greater?(x=w3709, y=2) -> (0:w3710:bool)
        n927 = call "Drive_Vi.vi"("Middle Thumb"=TRUE, "Z"=0.0, "Y"=0.0, "X"=0.0) -> ()  [unwired: 8 in]
      }
      n928 = call <vilib>:"WPI_SwitchRefNum Registry Get.vi"("refnum name"="Intake Sensor") -> ("error out"=w3386:errorcluster, "SwitchDevRef"=w3385:T4)  [unwired: 9 in]
      n929 = call <vilib>:"CTRE_Phoenix_MotorControl_RefNumRegistryGet.vi"("refnum name"="Intake") -> ("error out"=w3380:errorcluster, "PhoenixMotorControlDevRef"=w3379:T7)  [unwired: 9 in]
      n930 = call <vilib>:"CTRE_Phoenix_MotorControl_RefNumRegistryGet.vi"("refnum name"="Reject") -> ("error out"=w3382:errorcluster, "PhoenixMotorControlDevRef"=w3381:T7)  [unwired: 9 in]
      n931 = call "Limit_Switches.vi"() -> ()  [unwired: 10 in, 2 out]
      n932 = call <vilib>:"CTRE_Phoenix_MotorControl_RefNumRegistryGet.vi"("refnum name"="Elevate") -> ("error out"=w3384:errorcluster, "PhoenixMotorControlDevRef"=w3383:T7)  [unwired: 9 in]
      n933 = call <vilib>:"WPI_SwitchRefNum Registry Get.vi"("refnum name"="Elevate Sensor") -> ("error out"=w3388:errorcluster, "SwitchDevRef"=w3387:T4)  [unwired: 9 in]
      n934 = call <vilib>:"CTRE_Phoenix_MotorControl_RefNumRegistryGet.vi"("refnum name"="Shoot") -> ("error out"=w3368:errorcluster, "PhoenixMotorControlDevRef"=w3367:T7)  [unwired: 9 in]
      n935 = call <vilib>:"CTRE_Phoenix_MotorControl_RefNumRegistryGet.vi"("refnum name"="Intake Actuate") -> ("error out"=w3334:errorcluster, "PhoenixMotorControlDevRef"=w3335:T7)  [unwired: 9 in]
      n936 = while {
        tunnel: w3388 -> [w3668]
        tunnel: w3387 -> [w3667]
        tunnel: w3386 -> [w3666]
        tunnel: w3385 -> [w3665]
        tunnel: w3384 -> [w3662]
        tunnel: w3383 -> [w3661]
        tunnel: w3382 -> [w3660]
        tunnel: w3381 -> [w3659]
        tunnel: w3380 -> [w3658]
        tunnel: w3379 -> [w3657]
        tunnel: [w3646] -> w3372
        tunnel: [w3645] -> w3371
        tunnel: [w3644] -> w3370
        tunnel: [w3643] -> w3369
        tunnel: w3368 -> [w3642]
        tunnel: w3367 -> [w3641]
        tunnel: [w3638] -> w3366
        tunnel: [w3637] -> w3365
        i -> [w3671]
        stop <- w3672 stop-if-true
        w3640 = T11 0 items=["PercentOutput"=0, "Position"=1, "Velocity"=2, "Current"=3, "Follower"=5, "MotionProfile"=6, "MotionMagic"=7, "MotionProfileArc"=10, "Disabled"=15] ("Control Mode")
        w3651 = T11 0 items=["PercentOutput"=0, "Position"=1, "Velocity"=2, "Current"=3, "Follower"=5, "MotionProfile"=6, "MotionMagic"=7, "MotionProfileArc"=10, "Disabled"=15] ("Control Mode")
        w3652 = T11 0 items=["PercentOutput"=0, "Position"=1, "Velocity"=2, "Current"=3, "Follower"=5, "MotionProfile"=6, "MotionMagic"=7, "MotionProfileArc"=10, "Disabled"=15] ("Control Mode")
        w3653 = T11 0 items=["PercentOutput"=0, "Position"=1, "Velocity"=2, "Current"=3, "Follower"=5, "MotionProfile"=6, "MotionMagic"=7, "MotionProfileArc"=10, "Disabled"=15] ("Control Mode")
        n937 = call <vilib>:"WPI_SwitchGetLimitValue.vi"("error in (no error)"=w3666, "SwitchDevRef"=w3665) -> ("Switch Pressed"=w3669:bool)  [unwired: 7 in, 2 out]
        n938 = call <vilib>:"WPI_SwitchGetLimitValue.vi"("error in (no error)"=w3668, "SwitchDevRef"=w3667) -> ("Switch Pressed"=w3670:bool)  [unwired: 7 in, 2 out]
        n939 = Greater?(x=w3671, y=20) -> (0:w3672:bool)
        n940 = Not(x=w3669) -> (.not. x?=w3656:bool)
        "Intake 2" <- w3656
        n941 = Not(x=w3670) -> (.not. x?=w3664:bool)
        "Elevate 2" <- w3664
        n942 = Wait (ms)(milliseconds to wait=u32 100) -> ()  [unwired: 1 out]
        n943 = case shown="True" w3664 {
          tunnel: [0.75 ("Output") w3689] -> w3663
          tunnel: w3656 -> [_ w3686]
          tunnel: [0.75 ("Output") w3688] -> w3655
          tunnel: [-0.1 ("Output") w3687] -> w3654
          tunnel: [FALSE ("Middle Thumb") w3685] -> w3650
          tunnel: [0.0 ("Z") w3684] -> w3649
          tunnel: [0.0 ("Y") w3683] -> w3648
          tunnel: [0.0 ("X") w3682] -> w3647
          frame False {
            (unwired) WPI_SolenoidValue."Reverse" ("Value")
          }
          frame True {
            n944 = case shown="False" w3686 {
              tunnel: [0.75 ("Output") 0.0 ("Output")] -> w3689
              tunnel: [0.0 ("Output") 0.0 ("Output")] -> w3688
              tunnel: [0.0 ("Output") 0.0 ("Output")] -> w3687
              tunnel: [FALSE ("Middle Thumb") FALSE ("Middle Thumb")] -> w3685
              tunnel: [0.0 ("Z") 0.0 ("Z")] -> w3684
              tunnel: [-0.3 ("Y") 0.0 ("Y")] -> w3683
              tunnel: [0.0 ("X") 0.0 ("X")] -> w3682
              frame False {
              }
              frame True {
                (unwired) WPI_SolenoidValue."Forward" ("Value")
              }
            }
          }
        }
        n945 = call <vilib>:"CTRE_Phoenix_MotorControl_Set.vi"("error in (no error)"=w3658, "Output"=w3663, "Control Mode"=w3651, "PhoenixMotorControlDevRef"=w3657) -> ("error out"=w3644:errorcluster, "PhoenixMotorControlDevRef"=w3643:T7)  [unwired: 6 in]
        n946 = call <vilib>:"CTRE_Phoenix_MotorControl_Set.vi"("error in (no error)"=w3660, "Output"=w3655, "Control Mode"=w3652, "PhoenixMotorControlDevRef"=w3659) -> ()  [unwired: 6 in, 2 out]
        n947 = call <vilib>:"CTRE_Phoenix_MotorControl_Set.vi"("error in (no error)"=w3662, "Output"=w3654, "Control Mode"=w3653, "PhoenixMotorControlDevRef"=w3661) -> ("error out"=w3646:errorcluster, "PhoenixMotorControlDevRef"=w3645:T7)  [unwired: 6 in]
        n948 = call <vilib>:"CTRE_Phoenix_MotorControl_Set.vi"("error in (no error)"=w3642, "Output"=-0.55, "Control Mode"=w3640, "PhoenixMotorControlDevRef"=w3641) -> ("error out"=w3638:errorcluster, "PhoenixMotorControlDevRef"=w3637:T7)  [unwired: 6 in]
        n949 = call "Drive_Vi.vi"("Middle Thumb"=w3650, "Z"=w3649, "Y"=w3648, "X"=w3647) -> ()  [unwired: 8 in]
      }
      n950 = while {
        tunnel: w3335 -> [w3416]
        tunnel: w3334 -> [w3415]
        i -> [w3408]
        stop <- w3407 stop-if-true
        n951 = for {
          N: 20 -> [_]
          tunnel: w3416 -> [w3428]
          tunnel: w3415 -> [w3427]
          tunnel: [w3426] -> w3414 mode=indexing
          tunnel: [w3425] -> w3413 mode=indexing
          w3423 = T11 0 items=["PercentOutput"=0, "Position"=1, "Velocity"=2, "Current"=3, "Follower"=5, "MotionProfile"=6, "MotionMagic"=7, "MotionProfileArc"=10, "Disabled"=15] ("Control Mode")
          n952 = call <vilib>:"CTRE_Phoenix_MotorControl_Set.vi"("error in (no error)"=w3427, "Output"=-0.1, "Control Mode"=w3423, "PhoenixMotorControlDevRef"=w3428) -> ("error out"=w3425:errorcluster, "PhoenixMotorControlDevRef"=w3426:T7)  [unwired: 6 in]
          n953 = Wait (ms)(milliseconds to wait=u32 35) -> ()  [unwired: 1 out]
        }
        n954 = for {
          N: 20 -> [_]
          tunnel: w3414 -> [w3421] mode=indexing
          tunnel: w3413 -> [w3420] mode=indexing
          w3418 = T11 0 items=["PercentOutput"=0, "Position"=1, "Velocity"=2, "Current"=3, "Follower"=5, "MotionProfile"=6, "MotionMagic"=7, "MotionProfileArc"=10, "Disabled"=15] ("Control Mode")
          n955 = Wait (ms)(milliseconds to wait=u32 50) -> ()  [unwired: 1 out]
          n956 = call <vilib>:"CTRE_Phoenix_MotorControl_Set.vi"("error in (no error)"=w3420, "Output"=0.0, "Control Mode"=w3418, "PhoenixMotorControlDevRef"=w3421) -> ()  [unwired: 6 in, 2 out]
        }
        n957 = Greater?(x=w3408, y=2) -> (0:w3407:bool)
        n958 = Wait (ms)(milliseconds to wait=u32 20) -> ()  [unwired: 1 out]
      }
      n959 = call <vilib>:"WPI_SwitchRefNum Registry Get.vi"("refnum name"="Orange Limit Switch") -> ("error out"=w3374:errorcluster, "SwitchDevRef"=w3373:T4)  [unwired: 9 in]
      n960 = call <vilib>:"WPI_SwitchRefNum Registry Get.vi"("refnum name"="Blue Limit Switch") -> ("error out"=w3376:errorcluster, "SwitchDevRef"=w3375:T4)  [unwired: 9 in]
      n961 = while {
        tunnel: w3366 -> [_]
        tunnel: w3365 -> [_]
        tunnel: w3376 -> [w3634]
        tunnel: w3375 -> [w3633]
        tunnel: w3374 -> [w3632]
        tunnel: w3373 -> [w3631]
        tunnel: w3372 -> [w3610]
        tunnel: w3371 -> [w3609]
        tunnel: w3370 -> [w3605]
        tunnel: w3369 -> [w3606]
        tunnel: [w3614] -> w3364
        tunnel: [w3613] -> w3363
        tunnel: [w3612] -> w3362
        tunnel: [w3611] -> w3361
        tunnel: [w3610] -> w3360
        tunnel: [w3609] -> w3359
        tunnel: [w3608] -> w3358
        tunnel: [w3607] -> w3357
        i -> [w3620]
        stop <- w3619 stop-if-true
        w3604 = T11 0 items=["PercentOutput"=0, "Position"=1, "Velocity"=2, "Current"=3, "Follower"=5, "MotionProfile"=6, "MotionMagic"=7, "MotionProfileArc"=10, "Disabled"=15] ("Control Mode")
        n962 = call <vilib>:"WPI_SwitchGetLimitValue.vi"("error in (no error)"=w3632, "SwitchDevRef"=w3631) -> ("error out"=w3611:errorcluster, "Switch Pressed"=w3630:bool, "SwitchDevRef"=w3612:T4)  [unwired: 7 in]
        "Orange Limit Pressed 3" <- w3630
        n963 = call <vilib>:"WPI_SwitchGetLimitValue.vi"("error in (no error)"=w3634, "SwitchDevRef"=w3633) -> ("error out"=w3613:errorcluster, "Switch Pressed"=w3629:bool, "SwitchDevRef"=w3614:T4)  [unwired: 7 in]
        "Blue Limit Pressed 3" <- w3629
        n964 = call-poly <vilib>:"NT Read Value.vi"("Default Value"=0.0, "Name"="/limelight-drtrain/ty") -> ("Numeric"=w3624:dbl)  [unwired: 8 in, 1 out]
        "Ty 3" <- w3624
        n965 = Greater?(x=w3620, y=5) -> (0:w3619:bool)
        n966 = call "Turret_Aim.vi"("View Button"=FALSE ("Driver Right Thumb"), "Left Trigger"=2.0, "Orange Limit Pressed"=w3629, "Blue Limit Pressed"=w3630, "Right Bumper"=FALSE, "Left Bumper"=FALSE) -> ()  [unwired: 6 in]
        n967 = call "Shooter_Equation.vi"("Right Trigger"=2.0, "Ty"=w3624) -> ()  [unwired: 10 in]
        n968 = Wait (ms)(milliseconds to wait=u32 100) -> ()  [unwired: 1 out]
        n969 = call "Drive_Vi.vi"("Middle Thumb"=FALSE, "Z"=0.0, "Y"=0.15, "X"=0.0) -> ()  [unwired: 8 in]
        n970 = call <vilib>:"CTRE_Phoenix_MotorControl_Set.vi"("error in (no error)"=w3605, "Output"=0.0, "Control Mode"=w3604, "PhoenixMotorControlDevRef"=w3606) -> ("error out"=w3607:errorcluster, "PhoenixMotorControlDevRef"=w3608:T7)  [unwired: 6 in]
      }
      n971 = while {
        tunnel: w3363 -> [w3600]
        tunnel: w3364 -> [w3599]
        tunnel: w3361 -> [w3598]
        tunnel: w3360 -> [w3585]
        tunnel: w3359 -> [w3584]
        tunnel: w3357 -> [w3583]
        tunnel: w3358 -> [w3582]
        tunnel: w3362 -> [w3573]
        tunnel: [w3572] -> w3356
        tunnel: [w3571] -> w3355
        tunnel: [w3570] -> w3354
        tunnel: [w3569] -> w3353
        i -> [w3587]
        stop <- w3586 stop-if-true
        w3580 = T11 0 items=["PercentOutput"=0, "Position"=1, "Velocity"=2, "Current"=3, "Follower"=5, "MotionProfile"=6, "MotionMagic"=7, "MotionProfileArc"=10, "Disabled"=15] ("Control Mode")
        w3581 = T11 0 items=["PercentOutput"=0, "Position"=1, "Velocity"=2, "Current"=3, "Follower"=5, "MotionProfile"=6, "MotionMagic"=7, "MotionProfileArc"=10, "Disabled"=15] ("Control Mode")
        # "40"
        n972 = call <vilib>:"WPI_SwitchGetLimitValue.vi"("error in (no error)"=w3598, "SwitchDevRef"=w3573) -> ("Switch Pressed"=w3597:bool)  [unwired: 7 in, 2 out]
        "Orange Limit Pressed 4" <- w3597
        n973 = call <vilib>:"WPI_SwitchGetLimitValue.vi"("error in (no error)"=w3600, "SwitchDevRef"=w3599) -> ("Switch Pressed"=w3596:bool)  [unwired: 7 in, 2 out]
        "Blue Limit Pressed 4" <- w3596
        n974 = call-poly <vilib>:"NT Read Value.vi"("Default Value"=0.0, "Name"="/limelight-drtrain/ty") -> ("Numeric"=w3591:dbl)  [unwired: 8 in, 1 out]
        "Ty 4" <- w3591
        n975 = Greater?(x=w3587, y=20) -> (0:w3586:bool)
        n976 = call "Turret_Aim.vi"("View Button"=FALSE ("Driver Right Thumb"), "Left Trigger"=2.0, "Orange Limit Pressed"=w3596, "Blue Limit Pressed"=w3597, "Right Bumper"=FALSE, "Left Bumper"=FALSE) -> ()  [unwired: 6 in]
        n977 = call "Shooter_Equation.vi"("Right Trigger"=2.0, "Ty"=w3591) -> ()  [unwired: 10 in]
        n978 = Wait (ms)(milliseconds to wait=u32 100) -> ()  [unwired: 1 out]
        n979 = call "Drive_Vi.vi"("Middle Thumb"=FALSE, "Z"=0.0, "Y"=0.15, "X"=0.0) -> ()  [unwired: 8 in]
        n980 = call <vilib>:"CTRE_Phoenix_MotorControl_Set.vi"("error in (no error)"=w3583, "Output"=0.35, "Control Mode"=w3580, "PhoenixMotorControlDevRef"=w3582) -> ("error out"=w3572:errorcluster, "PhoenixMotorControlDevRef"=w3571:T7)  [unwired: 6 in]
        n981 = call <vilib>:"CTRE_Phoenix_MotorControl_Set.vi"("error in (no error)"=w3585, "Output"=-0.35, "Control Mode"=w3581, "PhoenixMotorControlDevRef"=w3584) -> ("error out"=w3569:errorcluster, "PhoenixMotorControlDevRef"=w3570:T7)  [unwired: 6 in]
      }
      n982 = while {
        tunnel: w3356 -> [w3564]
        tunnel: w3355 -> [w3563]
        tunnel: w3354 -> [w3562]
        tunnel: w3353 -> [w3561]
        tunnel: [w3552] -> w3333
        tunnel: [w3551] -> w3331
        tunnel: [w3550] -> w3329
        tunnel: [w3549] -> w3327
        i -> [w3559]
        stop <- w3558 stop-if-true
        w3567 = T11 0 items=["PercentOutput"=0, "Position"=1, "Velocity"=2, "Current"=3, "Follower"=5, "MotionProfile"=6, "MotionMagic"=7, "MotionProfileArc"=10, "Disabled"=15] ("Control Mode")
        w3568 = T11 0 items=["PercentOutput"=0, "Position"=1, "Velocity"=2, "Current"=3, "Follower"=5, "MotionProfile"=6, "MotionMagic"=7, "MotionProfileArc"=10, "Disabled"=15] ("Control Mode")
        n983 = call <vilib>:"CTRE_Phoenix_MotorControl_Set.vi"("error in (no error)"=w3564, "Output"=0.0, "Control Mode"=w3567, "PhoenixMotorControlDevRef"=w3563) -> ("error out"=w3551:errorcluster, "PhoenixMotorControlDevRef"=w3552:T7)  [unwired: 6 in]
        n984 = call <vilib>:"CTRE_Phoenix_MotorControl_Set.vi"("error in (no error)"=w3561, "Output"=0.0, "Control Mode"=w3568, "PhoenixMotorControlDevRef"=w3562) -> ("error out"=w3549:errorcluster, "PhoenixMotorControlDevRef"=w3550:T7)  [unwired: 6 in]
        n985 = call "Drive_Vi.vi"("Middle Thumb"=FALSE, "Z"=-0.35, "Y"=0.0, "X"=0.0) -> ()  [unwired: 8 in]
        n986 = Greater?(x=w3559, y=5) -> (0:w3558:bool)
        n987 = Wait (ms)(milliseconds to wait=u32 100) -> ()  [unwired: 1 out]
        n988 = call-poly <vilib>:"NT Read Value.vi"("Default Value"=0.0, "Name"="/limelight-drtrain/ty") -> ("Numeric"=w3554:dbl)  [unwired: 8 in, 1 out]
        "Ty 9" <- w3554
        n989 = call "Shooter_Equation.vi"("Right Trigger"=0.0, "Ty"=w3554) -> ()  [unwired: 10 in]
      }
      n990 = while {
        tunnel: [w3398] -> w3332
        tunnel: w3333 -> [w3398]
        tunnel: [w3397] -> w3330
        tunnel: w3331 -> [w3397]
        tunnel: [w3396] -> w3328
        tunnel: w3329 -> [w3396]
        tunnel: [w3395] -> w3326
        tunnel: w3327 -> [w3395]
        i -> [w3404]
        stop <- w3405 stop-if-true
        n991 = Wait (ms)(milliseconds to wait=u32 20) -> ()  [unwired: 1 out]
        n992 = Greater?(x=w3404, y=5) -> (0:w3405:bool)
        n993 = call "Drive_Vi.vi"("Middle Thumb"=TRUE, "Z"=0.0, "Y"=0.0, "X"=0.0) -> ()  [unwired: 8 in]
      }
      n994 = while {
        tunnel: w3332 -> [w3528]
        tunnel: w3330 -> [w3527]
        tunnel: w3328 -> [w3526]
        tunnel: w3326 -> [w3525]
        tunnel: [w3524] -> w3352
        tunnel: [w3523] -> w3351
        tunnel: [w3522] -> w3350
        tunnel: [w3521] -> w3349
        i -> [w3539]
        stop <- w3538 stop-if-true
        w3543 = T11 0 items=["PercentOutput"=0, "Position"=1, "Velocity"=2, "Current"=3, "Follower"=5, "MotionProfile"=6, "MotionMagic"=7, "MotionProfileArc"=10, "Disabled"=15] ("Control Mode")
        w3544 = T11 0 items=["PercentOutput"=0, "Position"=1, "Velocity"=2, "Current"=3, "Follower"=5, "MotionProfile"=6, "MotionMagic"=7, "MotionProfileArc"=10, "Disabled"=15] ("Control Mode")
        # "-0.186"
        # "-0.944"
        # ".135"
        n995 = call "Drive_Vi.vi"("Middle Thumb"=FALSE, "Z"=0.0, "Y"=-0.8, "X"=0.0) -> ()  [unwired: 8 in]
        n996 = call <vilib>:"CTRE_Phoenix_MotorControl_Set.vi"("error in (no error)"=w3527, "Output"=0.0, "Control Mode"=w3543, "PhoenixMotorControlDevRef"=w3528) -> ("error out"=w3523:errorcluster, "PhoenixMotorControlDevRef"=w3524:T7)  [unwired: 6 in]
        n997 = call <vilib>:"CTRE_Phoenix_MotorControl_Set.vi"("error in (no error)"=w3525, "Output"=0.0, "Control Mode"=w3544, "PhoenixMotorControlDevRef"=w3526) -> ("error out"=w3521:errorcluster, "PhoenixMotorControlDevRef"=w3522:T7)  [unwired: 6 in]
        n998 = Greater?(x=w3539, y=8) -> (0:w3538:bool)
        n999 = Wait (ms)(milliseconds to wait=u32 100) -> ()  [unwired: 1 out]
        n1000 = call-poly <vilib>:"NT Read Value.vi"("Default Value"=0.0, "Name"="/limelight-drtrain/ty") -> ("Numeric"=w3530:dbl)  [unwired: 8 in, 1 out]
        "Ty 10" <- w3530
        n1001 = call "Shooter_Equation.vi"("Right Trigger"=0.0, "Ty"=w3530) -> ()  [unwired: 10 in]
      }
      n1002 = while {
        tunnel: w3352 -> [w3512]
        tunnel: w3351 -> [w3511]
        tunnel: w3350 -> [w3510]
        tunnel: w3349 -> [w3509]
        tunnel: [w3504] -> w3348
        tunnel: [w3503] -> w3347
        tunnel: [w3502] -> w3346
        tunnel: [w3501] -> w3345
        i -> [w3506]
        stop <- w3505 stop-if-true
        w3519 = T11 0 items=["PercentOutput"=0, "Position"=1, "Velocity"=2, "Current"=3, "Follower"=5, "MotionProfile"=6, "MotionMagic"=7, "MotionProfileArc"=10, "Disabled"=15] ("Control Mode")
        w3520 = T11 0 items=["PercentOutput"=0, "Position"=1, "Velocity"=2, "Current"=3, "Follower"=5, "MotionProfile"=6, "MotionMagic"=7, "MotionProfileArc"=10, "Disabled"=15] ("Control Mode")
        # "-0.186"
        # "-0.944"
        # ".135"
        n1003 = call <vilib>:"CTRE_Phoenix_MotorControl_Set.vi"("error in (no error)"=w3511, "Output"=0.0, "Control Mode"=w3519, "PhoenixMotorControlDevRef"=w3512) -> ("error out"=w3503:errorcluster, "PhoenixMotorControlDevRef"=w3504:T7)  [unwired: 6 in]
        n1004 = call <vilib>:"CTRE_Phoenix_MotorControl_Set.vi"("error in (no error)"=w3509, "Output"=0.0, "Control Mode"=w3520, "PhoenixMotorControlDevRef"=w3510) -> ("error out"=w3501:errorcluster, "PhoenixMotorControlDevRef"=w3502:T7)  [unwired: 6 in]
        n1005 = call "Drive_Vi.vi"("Middle Thumb"=FALSE, "Z"=0.0, "Y"=0.0, "X"=0.0) -> ()  [unwired: 8 in]
        n1006 = Greater?(x=w3506, y=5) -> (0:w3505:bool)
        n1007 = call-poly <vilib>:"NT Read Value.vi"("Default Value"=0.0, "Name"="/limelight-drtrain/ty") -> ("Numeric"=w3514:dbl)  [unwired: 8 in, 1 out]
        "Ty 11" <- w3514
        n1008 = Wait (ms)(milliseconds to wait=u32 100) -> ()  [unwired: 1 out]
        n1009 = call "Shooter_Equation.vi"("Right Trigger"=0.0, "Ty"=w3514) -> ()  [unwired: 10 in]
      }
      n1010 = while {
        tunnel: w3348 -> [w3484]
        tunnel: w3347 -> [w3483]
        tunnel: w3346 -> [w3482]
        tunnel: w3345 -> [w3481]
        tunnel: [w3476] -> w3344
        tunnel: [w3475] -> w3343
        tunnel: [w3474] -> w3342
        tunnel: [w3473] -> w3341
        i -> [w3478]
        stop <- w3477 stop-if-true
        w3495 = T11 0 items=["PercentOutput"=0, "Position"=1, "Velocity"=2, "Current"=3, "Follower"=5, "MotionProfile"=6, "MotionMagic"=7, "MotionProfileArc"=10, "Disabled"=15] ("Control Mode")
        w3496 = T11 0 items=["PercentOutput"=0, "Position"=1, "Velocity"=2, "Current"=3, "Follower"=5, "MotionProfile"=6, "MotionMagic"=7, "MotionProfileArc"=10, "Disabled"=15] ("Control Mode")
        # "-0.186"
        # "-0.944"
        # ".135"
        n1011 = call "Drive_Vi.vi"("Middle Thumb"=FALSE, "Z"=0.0, "Y"=0.0, "X"=0.0) -> ()  [unwired: 8 in]
        n1012 = call <vilib>:"CTRE_Phoenix_MotorControl_Set.vi"("error in (no error)"=w3483, "Output"=0.75, "Control Mode"=w3495, "PhoenixMotorControlDevRef"=w3484) -> ("error out"=w3475:errorcluster, "PhoenixMotorControlDevRef"=w3476:T7)  [unwired: 6 in]
        n1013 = call <vilib>:"CTRE_Phoenix_MotorControl_Set.vi"("error in (no error)"=w3481, "Output"=-0.1, "Control Mode"=w3496, "PhoenixMotorControlDevRef"=w3482) -> ("error out"=w3473:errorcluster, "PhoenixMotorControlDevRef"=w3474:T7)  [unwired: 6 in]
        n1014 = Greater?(x=w3478, y=20) -> (0:w3477:bool)
        n1015 = Wait (ms)(milliseconds to wait=u32 100) -> ()  [unwired: 1 out]
        n1016 = call-poly <vilib>:"NT Read Value.vi"("Default Value"=0.0, "Name"="/limelight-drtrain/ty") -> ("Numeric"=w3486:dbl)  [unwired: 8 in, 1 out]
        "Ty 12" <- w3486
        n1017 = call "Shooter_Equation.vi"("Right Trigger"=0.0, "Ty"=w3486) -> ()  [unwired: 10 in]
      }
      n1018 = while {
        tunnel: w3344 -> [w3460]
        tunnel: [w3453] -> _
        tunnel: w3342 -> [w3459]
        tunnel: w3341 -> [w3458]
        tunnel: w3343 -> [w3453]
        tunnel: [w3452] -> w3340
        tunnel: [w3451] -> w3339
        tunnel: [w3450] -> w3338
        tunnel: [w3449] -> w3337
        i -> [w3455]
        stop <- w3454 stop-if-true
        w3471 = T11 0 items=["PercentOutput"=0, "Position"=1, "Velocity"=2, "Current"=3, "Follower"=5, "MotionProfile"=6, "MotionMagic"=7, "MotionProfileArc"=10, "Disabled"=15] ("Control Mode")
        w3472 = T11 0 items=["PercentOutput"=0, "Position"=1, "Velocity"=2, "Current"=3, "Follower"=5, "MotionProfile"=6, "MotionMagic"=7, "MotionProfileArc"=10, "Disabled"=15] ("Control Mode")
        # "-0.186"
        # "-0.944"
        # ".135"
        n1019 = call "Drive_Vi.vi"("Middle Thumb"=FALSE, "Z"=0.0, "Y"=0.0, "X"=0.0) -> ()  [unwired: 8 in]
        n1020 = call <vilib>:"CTRE_Phoenix_MotorControl_Set.vi"("error in (no error)"=w3453, "Output"=0.0, "Control Mode"=w3471, "PhoenixMotorControlDevRef"=w3460) -> ("error out"=w3449:errorcluster, "PhoenixMotorControlDevRef"=w3450:T7)  [unwired: 6 in]
        n1021 = call <vilib>:"CTRE_Phoenix_MotorControl_Set.vi"("error in (no error)"=w3458, "Output"=0.0, "Control Mode"=w3472, "PhoenixMotorControlDevRef"=w3459) -> ("error out"=w3452:errorcluster, "PhoenixMotorControlDevRef"=w3451:T7)  [unwired: 6 in]
        n1022 = Greater?(x=w3455, y=10) -> (0:w3454:bool)
        n1023 = Wait (ms)(milliseconds to wait=u32 100) -> ()  [unwired: 1 out]
        n1024 = call-poly <vilib>:"NT Read Value.vi"("Default Value"=0.0, "Name"="/limelight-drtrain/ty") -> ("Numeric"=w3462:dbl)  [unwired: 8 in, 1 out]
        "Ty 13" <- w3462
        n1025 = call "Shooter_Equation.vi"("Right Trigger"=0.0, "Ty"=w3462) -> ()  [unwired: 10 in]
      }
      n1026 = while {
        tunnel: w3338 -> [w3436]
        tunnel: [w3429] -> _
        tunnel: w3339 -> [w3435]
        tunnel: w3340 -> [w3434]
        tunnel: w3337 -> [w3429]
        i -> [w3431]
        stop <- w3430 stop-if-true
        w3447 = T11 0 items=["PercentOutput"=0, "Position"=1, "Velocity"=2, "Current"=3, "Follower"=5, "MotionProfile"=6, "MotionMagic"=7, "MotionProfileArc"=10, "Disabled"=15] ("Control Mode")
        w3448 = T11 0 items=["PercentOutput"=0, "Position"=1, "Velocity"=2, "Current"=3, "Follower"=5, "MotionProfile"=6, "MotionMagic"=7, "MotionProfileArc"=10, "Disabled"=15] ("Control Mode")
        # "-0.186"
        # "-0.944"
        # ".135"
        n1027 = call "Drive_Vi.vi"("Middle Thumb"=FALSE, "Z"=0.0, "Y"=0.0, "X"=0.0) -> ()  [unwired: 8 in]
        n1028 = call <vilib>:"CTRE_Phoenix_MotorControl_Set.vi"("error in (no error)"=w3429, "Output"=0.0, "Control Mode"=w3447, "PhoenixMotorControlDevRef"=w3436) -> ()  [unwired: 6 in, 2 out]
        n1029 = call <vilib>:"CTRE_Phoenix_MotorControl_Set.vi"("error in (no error)"=w3434, "Output"=0.0, "Control Mode"=w3448, "PhoenixMotorControlDevRef"=w3435) -> ()  [unwired: 6 in, 2 out]
        n1030 = Greater?(x=w3431, y=20) -> (0:w3430:bool)
        n1031 = Wait (ms)(milliseconds to wait=u32 100) -> ()  [unwired: 1 out]
        n1032 = call-poly <vilib>:"NT Read Value.vi"("Default Value"=0.0, "Name"="/limelight-drtrain/ty") -> ("Numeric"=w3438:dbl)  [unwired: 8 in, 1 out]
        "Ty 14" <- w3438
        n1033 = call "Shooter_Equation.vi"("Right Trigger"=0.0, "Ty"=w3438) -> ()  [unwired: 10 in]
      }
    }
    frame "4 Ball Pos 3" {
      # "Pigeon Set"
      n1034 = while {
        i -> [w4127]
        stop <- w4128 stop-if-true
        n1035 = Wait (ms)(milliseconds to wait=u32 20) -> ()  [unwired: 1 out]
        n1036 = Greater?(x=w4127, y=2) -> (0:w4128:bool)
        n1037 = call "Drive_Vi.vi"("Middle Thumb"=TRUE, "Z"=0.0, "Y"=0.0, "X"=0.0) -> ()  [unwired: 8 in]
      }
      n1038 = call <vilib>:"WPI_SwitchRefNum Registry Get.vi"("refnum name"="Intake Sensor") -> ("error out"=w3780:errorcluster, "SwitchDevRef"=w3779:T4)  [unwired: 9 in]
      n1039 = call <vilib>:"CTRE_Phoenix_MotorControl_RefNumRegistryGet.vi"("refnum name"="Intake") -> ("error out"=w3774:errorcluster, "PhoenixMotorControlDevRef"=w3773:T7)  [unwired: 9 in]
      n1040 = call <vilib>:"CTRE_Phoenix_MotorControl_RefNumRegistryGet.vi"("refnum name"="Reject") -> ("error out"=w3776:errorcluster, "PhoenixMotorControlDevRef"=w3775:T7)  [unwired: 9 in]
      n1041 = call "Limit_Switches.vi"() -> ()  [unwired: 10 in, 2 out]
      n1042 = call <vilib>:"CTRE_Phoenix_MotorControl_RefNumRegistryGet.vi"("refnum name"="Elevate") -> ("error out"=w3778:errorcluster, "PhoenixMotorControlDevRef"=w3777:T7)  [unwired: 9 in]
      n1043 = call <vilib>:"WPI_SwitchRefNum Registry Get.vi"("refnum name"="Elevate Sensor") -> ("error out"=w3782:errorcluster, "SwitchDevRef"=w3781:T4)  [unwired: 9 in]
      n1044 = call <vilib>:"CTRE_Phoenix_MotorControl_RefNumRegistryGet.vi"("refnum name"="Shoot") -> ("error out"=w3762:errorcluster, "PhoenixMotorControlDevRef"=w3761:T7)  [unwired: 9 in]
      n1045 = call <vilib>:"CTRE_Phoenix_MotorControl_RefNumRegistryGet.vi"("refnum name"="Intake Actuate") -> ("error out"=w3732:errorcluster, "PhoenixMotorControlDevRef"=w3733:T7)  [unwired: 9 in]
      n1046 = while {
        tunnel: w3782 -> [w4086]
        tunnel: w3781 -> [w4085]
        tunnel: w3780 -> [w4084]
        tunnel: w3779 -> [w4083]
        tunnel: w3778 -> [w4080]
        tunnel: w3777 -> [w4079]
        tunnel: w3776 -> [w4078]
        tunnel: w3775 -> [w4077]
        tunnel: w3774 -> [w4076]
        tunnel: w3773 -> [w4075]
        tunnel: [w4064] -> w3766
        tunnel: [w4063] -> w3765
        tunnel: [w4062] -> w3764
        tunnel: [w4061] -> w3763
        tunnel: w3762 -> [w4060]
        tunnel: w3761 -> [w4059]
        tunnel: [w4056] -> w3760
        tunnel: [w4055] -> w3759
        i -> [w4089]
        stop <- w4090 stop-if-true
        w4058 = T11 0 items=["PercentOutput"=0, "Position"=1, "Velocity"=2, "Current"=3, "Follower"=5, "MotionProfile"=6, "MotionMagic"=7, "MotionProfileArc"=10, "Disabled"=15] ("Control Mode")
        w4069 = T11 0 items=["PercentOutput"=0, "Position"=1, "Velocity"=2, "Current"=3, "Follower"=5, "MotionProfile"=6, "MotionMagic"=7, "MotionProfileArc"=10, "Disabled"=15] ("Control Mode")
        w4070 = T11 0 items=["PercentOutput"=0, "Position"=1, "Velocity"=2, "Current"=3, "Follower"=5, "MotionProfile"=6, "MotionMagic"=7, "MotionProfileArc"=10, "Disabled"=15] ("Control Mode")
        w4071 = T11 0 items=["PercentOutput"=0, "Position"=1, "Velocity"=2, "Current"=3, "Follower"=5, "MotionProfile"=6, "MotionMagic"=7, "MotionProfileArc"=10, "Disabled"=15] ("Control Mode")
        n1047 = call <vilib>:"WPI_SwitchGetLimitValue.vi"("error in (no error)"=w4084, "SwitchDevRef"=w4083) -> ("Switch Pressed"=w4087:bool)  [unwired: 7 in, 2 out]
        n1048 = call <vilib>:"WPI_SwitchGetLimitValue.vi"("error in (no error)"=w4086, "SwitchDevRef"=w4085) -> ("Switch Pressed"=w4088:bool)  [unwired: 7 in, 2 out]
        n1049 = Greater?(x=w4089, y=20) -> (0:w4090:bool)
        n1050 = Not(x=w4087) -> (.not. x?=w4074:bool)
        "Intake 5" <- w4074
        n1051 = Not(x=w4088) -> (.not. x?=w4082:bool)
        "Elevate 5" <- w4082
        n1052 = Wait (ms)(milliseconds to wait=u32 100) -> ()  [unwired: 1 out]
        n1053 = case shown="True" w4082 {
          tunnel: [0.75 ("Output") w4107] -> w4081
          tunnel: w4074 -> [_ w4104]
          tunnel: [0.75 ("Output") w4106] -> w4073
          tunnel: [-0.1 ("Output") w4105] -> w4072
          tunnel: [FALSE ("Middle Thumb") w4103] -> w4068
          tunnel: [0.0 ("Z") w4102] -> w4067
          tunnel: [0.0 ("Y") w4101] -> w4066
          tunnel: [0.0 ("X") w4100] -> w4065
          frame False {
            (unwired) WPI_SolenoidValue."Reverse" ("Value")
          }
          frame True {
            n1054 = case shown="True" w4104 {
              tunnel: [0.75 ("Output") 0.0 ("Output")] -> w4107
              tunnel: [0.0 ("Output") 0.0 ("Output")] -> w4106
              tunnel: [0.0 ("Output") 0.0 ("Output")] -> w4105
              tunnel: [FALSE ("Middle Thumb") FALSE ("Middle Thumb")] -> w4103
              tunnel: [0.0 ("Z") 0.0 ("Z")] -> w4102
              tunnel: [-0.3 ("Y") 0.0 ("Y")] -> w4101
              tunnel: [0.0 ("X") 0.0 ("X")] -> w4100
              frame False {
              }
              frame True {
              }
            }
          }
        }
        n1055 = call <vilib>:"CTRE_Phoenix_MotorControl_Set.vi"("error in (no error)"=w4076, "Output"=w4081, "Control Mode"=w4069, "PhoenixMotorControlDevRef"=w4075) -> ("error out"=w4062:errorcluster, "PhoenixMotorControlDevRef"=w4061:T7)  [unwired: 6 in]
        n1056 = call <vilib>:"CTRE_Phoenix_MotorControl_Set.vi"("error in (no error)"=w4078, "Output"=w4073, "Control Mode"=w4070, "PhoenixMotorControlDevRef"=w4077) -> ()  [unwired: 6 in, 2 out]
        n1057 = call <vilib>:"CTRE_Phoenix_MotorControl_Set.vi"("error in (no error)"=w4080, "Output"=w4072, "Control Mode"=w4071, "PhoenixMotorControlDevRef"=w4079) -> ("error out"=w4064:errorcluster, "PhoenixMotorControlDevRef"=w4063:T7)  [unwired: 6 in]
        n1058 = call <vilib>:"CTRE_Phoenix_MotorControl_Set.vi"("error in (no error)"=w4060, "Output"=-0.55, "Control Mode"=w4058, "PhoenixMotorControlDevRef"=w4059) -> ("error out"=w4056:errorcluster, "PhoenixMotorControlDevRef"=w4055:T7)  [unwired: 6 in]
        n1059 = call "Drive_Vi.vi"("Middle Thumb"=w4068, "Z"=w4067, "Y"=w4066, "X"=w4065) -> ()  [unwired: 8 in]
      }
      n1060 = while {
        tunnel: w3733 -> [w3822]
        tunnel: w3732 -> [w3821]
        i -> [w3814]
        stop <- w3813 stop-if-true
        n1061 = for {
          N: 20 -> [_]
          tunnel: w3822 -> [w3834]
          tunnel: w3821 -> [w3833]
          tunnel: [w3832] -> w3820 mode=indexing
          tunnel: [w3831] -> w3819 mode=indexing
          w3829 = T11 0 items=["PercentOutput"=0, "Position"=1, "Velocity"=2, "Current"=3, "Follower"=5, "MotionProfile"=6, "MotionMagic"=7, "MotionProfileArc"=10, "Disabled"=15] ("Control Mode")
          n1062 = call <vilib>:"CTRE_Phoenix_MotorControl_Set.vi"("error in (no error)"=w3833, "Output"=-0.1, "Control Mode"=w3829, "PhoenixMotorControlDevRef"=w3834) -> ("error out"=w3831:errorcluster, "PhoenixMotorControlDevRef"=w3832:T7)  [unwired: 6 in]
          n1063 = Wait (ms)(milliseconds to wait=u32 35) -> ()  [unwired: 1 out]
        }
        n1064 = for {
          N: 20 -> [_]
          tunnel: w3820 -> [w3827] mode=indexing
          tunnel: w3819 -> [w3826] mode=indexing
          w3824 = T11 0 items=["PercentOutput"=0, "Position"=1, "Velocity"=2, "Current"=3, "Follower"=5, "MotionProfile"=6, "MotionMagic"=7, "MotionProfileArc"=10, "Disabled"=15] ("Control Mode")
          n1065 = Wait (ms)(milliseconds to wait=u32 50) -> ()  [unwired: 1 out]
          n1066 = call <vilib>:"CTRE_Phoenix_MotorControl_Set.vi"("error in (no error)"=w3826, "Output"=0.0, "Control Mode"=w3824, "PhoenixMotorControlDevRef"=w3827) -> ()  [unwired: 6 in, 2 out]
        }
        n1067 = Greater?(x=w3814, y=2) -> (0:w3813:bool)
        n1068 = Wait (ms)(milliseconds to wait=u32 20) -> ()  [unwired: 1 out]
      }
      n1069 = call <vilib>:"WPI_SwitchRefNum Registry Get.vi"("refnum name"="Orange Limit Switch") -> ("error out"=w3768:errorcluster, "SwitchDevRef"=w3767:T4)  [unwired: 9 in]
      n1070 = call <vilib>:"WPI_SwitchRefNum Registry Get.vi"("refnum name"="Blue Limit Switch") -> ("error out"=w3770:errorcluster, "SwitchDevRef"=w3769:T4)  [unwired: 9 in]
      n1071 = while {
        tunnel: w3760 -> [_]
        tunnel: w3759 -> [_]
        tunnel: w3770 -> [w4052]
        tunnel: w3769 -> [w4051]
        tunnel: w3768 -> [w4050]
        tunnel: w3767 -> [w4049]
        tunnel: w3766 -> [w4028]
        tunnel: w3765 -> [w4027]
        tunnel: w3764 -> [w4023]
        tunnel: w3763 -> [w4024]
        tunnel: [w4032] -> w3758
        tunnel: [w4031] -> w3757
        tunnel: [w4030] -> w3756
        tunnel: [w4029] -> w3755
        tunnel: [w4028] -> w3754
        tunnel: [w4027] -> w3753
        tunnel: [w4026] -> w3752
        tunnel: [w4025] -> w3751
        i -> [w4038]
        stop <- w4037 stop-if-true
        w4022 = T11 0 items=["PercentOutput"=0, "Position"=1, "Velocity"=2, "Current"=3, "Follower"=5, "MotionProfile"=6, "MotionMagic"=7, "MotionProfileArc"=10, "Disabled"=15] ("Control Mode")
        n1072 = call <vilib>:"WPI_SwitchGetLimitValue.vi"("error in (no error)"=w4050, "SwitchDevRef"=w4049) -> ("error out"=w4029:errorcluster, "Switch Pressed"=w4048:bool, "SwitchDevRef"=w4030:T4)  [unwired: 7 in]
        "Orange Limit Pressed 9" <- w4048
        n1073 = call <vilib>:"WPI_SwitchGetLimitValue.vi"("error in (no error)"=w4052, "SwitchDevRef"=w4051) -> ("error out"=w4031:errorcluster, "Switch Pressed"=w4047:bool, "SwitchDevRef"=w4032:T4)  [unwired: 7 in]
        "Blue Limit Pressed 9" <- w4047
        n1074 = call-poly <vilib>:"NT Read Value.vi"("Default Value"=0.0, "Name"="/limelight-drtrain/ty") -> ("Numeric"=w4042:dbl)  [unwired: 8 in, 1 out]
        "Ty 15" <- w4042
        n1075 = Greater?(x=w4038, y=5) -> (0:w4037:bool)
        n1076 = call "Turret_Aim.vi"("View Button"=FALSE ("Driver Right Thumb"), "Left Trigger"=2.0, "Orange Limit Pressed"=w4047, "Blue Limit Pressed"=w4048, "Right Bumper"=FALSE, "Left Bumper"=FALSE) -> ()  [unwired: 6 in]
        n1077 = call "Shooter_Equation.vi"("Right Trigger"=2.0, "Ty"=w4042) -> ()  [unwired: 10 in]
        n1078 = Wait (ms)(milliseconds to wait=u32 100) -> ()  [unwired: 1 out]
        n1079 = call "Drive_Vi.vi"("Middle Thumb"=FALSE, "Z"=0.0, "Y"=0.15, "X"=0.0) -> ()  [unwired: 8 in]
        n1080 = call <vilib>:"CTRE_Phoenix_MotorControl_Set.vi"("error in (no error)"=w4023, "Output"=0.0, "Control Mode"=w4022, "PhoenixMotorControlDevRef"=w4024) -> ("error out"=w4025:errorcluster, "PhoenixMotorControlDevRef"=w4026:T7)  [unwired: 6 in]
      }
      n1081 = while {
        tunnel: w3757 -> [w4018]
        tunnel: w3758 -> [w4017]
        tunnel: w3755 -> [w4016]
        tunnel: w3754 -> [w4005]
        tunnel: w3753 -> [w4004]
        tunnel: w3751 -> [w4003]
        tunnel: w3752 -> [w4002]
        tunnel: w3756 -> [w3993]
        tunnel: [w3992] -> w3750
        tunnel: [w3991] -> w3749
        tunnel: [w3990] -> w3748
        tunnel: [w3989] -> w3747
        tunnel: [w3988] -> w3715
        tunnel: [w3987] -> w3714
        i -> [w4007]
        stop <- w4006 stop-if-true
        w4000 = T11 0 items=["PercentOutput"=0, "Position"=1, "Velocity"=2, "Current"=3, "Follower"=5, "MotionProfile"=6, "MotionMagic"=7, "MotionProfileArc"=10, "Disabled"=15] ("Control Mode")
        w4001 = T11 0 items=["PercentOutput"=0, "Position"=1, "Velocity"=2, "Current"=3, "Follower"=5, "MotionProfile"=6, "MotionMagic"=7, "MotionProfileArc"=10, "Disabled"=15] ("Control Mode")
        # "40"
        n1082 = call <vilib>:"WPI_SwitchGetLimitValue.vi"("error in (no error)"=w4016, "SwitchDevRef"=w3993) -> ("Switch Pressed"=w3988:bool)  [unwired: 7 in, 2 out]
        "Orange Limit Pressed 10" <- w3988
        n1083 = call <vilib>:"WPI_SwitchGetLimitValue.vi"("error in (no error)"=w4018, "SwitchDevRef"=w4017) -> ("Switch Pressed"=w3987:bool)  [unwired: 7 in, 2 out]
        "Blue Limit Pressed 10" <- w3987
        n1084 = call-poly <vilib>:"NT Read Value.vi"("Default Value"=0.0, "Name"="/limelight-drtrain/ty") -> ("Numeric"=w4011:dbl)  [unwired: 8 in, 1 out]
        "Ty 16" <- w4011
        n1085 = Greater?(x=w4007, y=20) -> (0:w4006:bool)
        n1086 = call "Turret_Aim.vi"("View Button"=FALSE ("Driver Right Thumb"), "Left Trigger"=2.0, "Orange Limit Pressed"=w3987, "Blue Limit Pressed"=w3988, "Right Bumper"=FALSE, "Left Bumper"=FALSE) -> ()  [unwired: 6 in]
        n1087 = call "Shooter_Equation.vi"("Right Trigger"=2.0, "Ty"=w4011) -> ()  [unwired: 10 in]
        n1088 = Wait (ms)(milliseconds to wait=u32 100) -> ()  [unwired: 1 out]
        n1089 = call "Drive_Vi.vi"("Middle Thumb"=FALSE, "Z"=0.0, "Y"=0.15, "X"=0.0) -> ()  [unwired: 8 in]
        n1090 = call <vilib>:"CTRE_Phoenix_MotorControl_Set.vi"("error in (no error)"=w4003, "Output"=0.35, "Control Mode"=w4000, "PhoenixMotorControlDevRef"=w4002) -> ("error out"=w3992:errorcluster, "PhoenixMotorControlDevRef"=w3991:T7)  [unwired: 6 in]
        n1091 = call <vilib>:"CTRE_Phoenix_MotorControl_Set.vi"("error in (no error)"=w4005, "Output"=-0.35, "Control Mode"=w4001, "PhoenixMotorControlDevRef"=w4004) -> ("error out"=w3989:errorcluster, "PhoenixMotorControlDevRef"=w3990:T7)  [unwired: 6 in]
      }
      n1092 = while {
        tunnel: w3750 -> [w3982]
        tunnel: w3749 -> [w3981]
        tunnel: w3748 -> [w3980]
        tunnel: w3747 -> [w3979]
        tunnel: [w3970] -> w3731
        tunnel: [w3969] -> w3729
        tunnel: [w3968] -> w3727
        tunnel: [w3967] -> w3725
        i -> [w3977]
        stop <- w3976 stop-if-true
        w3985 = T11 0 items=["PercentOutput"=0, "Position"=1, "Velocity"=2, "Current"=3, "Follower"=5, "MotionProfile"=6, "MotionMagic"=7, "MotionProfileArc"=10, "Disabled"=15] ("Control Mode")
        w3986 = T11 0 items=["PercentOutput"=0, "Position"=1, "Velocity"=2, "Current"=3, "Follower"=5, "MotionProfile"=6, "MotionMagic"=7, "MotionProfileArc"=10, "Disabled"=15] ("Control Mode")
        n1093 = call <vilib>:"CTRE_Phoenix_MotorControl_Set.vi"("error in (no error)"=w3982, "Output"=0.0, "Control Mode"=w3985, "PhoenixMotorControlDevRef"=w3981) -> ("error out"=w3969:errorcluster, "PhoenixMotorControlDevRef"=w3970:T7)  [unwired: 6 in]
        n1094 = call <vilib>:"CTRE_Phoenix_MotorControl_Set.vi"("error in (no error)"=w3979, "Output"=0.0, "Control Mode"=w3986, "PhoenixMotorControlDevRef"=w3980) -> ("error out"=w3967:errorcluster, "PhoenixMotorControlDevRef"=w3968:T7)  [unwired: 6 in]
        n1095 = call "Drive_Vi.vi"("Middle Thumb"=FALSE, "Z"=0.22, "Y"=0.0, "X"=0.0) -> ()  [unwired: 8 in]
        n1096 = Greater?(x=w3977, y=4) -> (0:w3976:bool)
        n1097 = Wait (ms)(milliseconds to wait=u32 100) -> ()  [unwired: 1 out]
        n1098 = call-poly <vilib>:"NT Read Value.vi"("Default Value"=0.0, "Name"="/limelight-drtrain/ty") -> ("Numeric"=w3972:dbl)  [unwired: 8 in, 1 out]
        "Ty 17" <- w3972
        n1099 = call "Shooter_Equation.vi"("Right Trigger"=0.0, "Ty"=w3972) -> ()  [unwired: 10 in]
      }
      n1100 = while {
        tunnel: [w3804] -> w3730
        tunnel: w3731 -> [w3804]
        tunnel: [w3803] -> w3728
        tunnel: w3729 -> [w3803]
        tunnel: [w3802] -> w3726
        tunnel: w3727 -> [w3802]
        tunnel: [w3801] -> w3724
        tunnel: w3725 -> [w3801]
        i -> [w3810]
        stop <- w3811 stop-if-true
        n1101 = Wait (ms)(milliseconds to wait=u32 20) -> ()  [unwired: 1 out]
        n1102 = Greater?(x=w3810, y=5) -> (0:w3811:bool)
        n1103 = call "Drive_Vi.vi"("Middle Thumb"=TRUE, "Z"=0.0, "Y"=0.0, "X"=0.0) -> ()  [unwired: 8 in]
      }
      n1104 = while {
        tunnel: w3730 -> [w3946]
        tunnel: w3728 -> [w3945]
        tunnel: w3726 -> [w3944]
        tunnel: w3724 -> [w3943]
        tunnel: [w3942] -> w3746
        tunnel: [w3941] -> w3745
        tunnel: [w3940] -> w3744
        tunnel: [w3939] -> w3743
        i -> [w3957]
        stop <- w3956 stop-if-true
        w3961 = T11 0 items=["PercentOutput"=0, "Position"=1, "Velocity"=2, "Current"=3, "Follower"=5, "MotionProfile"=6, "MotionMagic"=7, "MotionProfileArc"=10, "Disabled"=15] ("Control Mode")
        w3962 = T11 0 items=["PercentOutput"=0, "Position"=1, "Velocity"=2, "Current"=3, "Follower"=5, "MotionProfile"=6, "MotionMagic"=7, "MotionProfileArc"=10, "Disabled"=15] ("Control Mode")
        # "-0.186"
        # "-0.944"
        # ".135"
        n1105 = call "Drive_Vi.vi"("Middle Thumb"=FALSE, "Z"=0.0, "Y"=-0.75, "X"=0.0) -> ()  [unwired: 8 in]
        n1106 = call <vilib>:"CTRE_Phoenix_MotorControl_Set.vi"("error in (no error)"=w3945, "Output"=1.0, "Control Mode"=w3961, "PhoenixMotorControlDevRef"=w3946) -> ("error out"=w3941:errorcluster, "PhoenixMotorControlDevRef"=w3942:T7)  [unwired: 6 in]
        n1107 = call <vilib>:"CTRE_Phoenix_MotorControl_Set.vi"("error in (no error)"=w3943, "Output"=0.0, "Control Mode"=w3962, "PhoenixMotorControlDevRef"=w3944) -> ("error out"=w3939:errorcluster, "PhoenixMotorControlDevRef"=w3940:T7)  [unwired: 6 in]
        n1108 = Greater?(x=w3957, y=3) -> (0:w3956:bool)
        n1109 = Wait (ms)(milliseconds to wait=u32 116) -> ()  [unwired: 1 out]
        n1110 = call-poly <vilib>:"NT Read Value.vi"("Default Value"=0.0, "Name"="/limelight-drtrain/ty") -> ("Numeric"=w3948:dbl)  [unwired: 8 in, 1 out]
        "Ty 18" <- w3948
        n1111 = call "Shooter_Equation.vi"("Right Trigger"=0.0, "Ty"=w3948) -> ()  [unwired: 10 in]
      }
      n1112 = while {
        tunnel: w3746 -> [w3930]
        tunnel: w3745 -> [w3929]
        tunnel: w3744 -> [w3928]
        tunnel: w3743 -> [w3927]
        tunnel: [w3922] -> w3742
        tunnel: [w3921] -> w3741
        tunnel: [w3920] -> w3740
        tunnel: [w3919] -> w3739
        i -> [w3924]
        stop <- w3923 stop-if-true
        w3937 = T11 0 items=["PercentOutput"=0, "Position"=1, "Velocity"=2, "Current"=3, "Follower"=5, "MotionProfile"=6, "MotionMagic"=7, "MotionProfileArc"=10, "Disabled"=15] ("Control Mode")
        w3938 = T11 0 items=["PercentOutput"=0, "Position"=1, "Velocity"=2, "Current"=3, "Follower"=5, "MotionProfile"=6, "MotionMagic"=7, "MotionProfileArc"=10, "Disabled"=15] ("Control Mode")
        # "-0.186"
        # "-0.944"
        # ".135"
        n1113 = call <vilib>:"CTRE_Phoenix_MotorControl_Set.vi"("error in (no error)"=w3929, "Output"=1.0, "Control Mode"=w3937, "PhoenixMotorControlDevRef"=w3930) -> ("error out"=w3921:errorcluster, "PhoenixMotorControlDevRef"=w3922:T7)  [unwired: 6 in]
        n1114 = call <vilib>:"CTRE_Phoenix_MotorControl_Set.vi"("error in (no error)"=w3927, "Output"=0.0, "Control Mode"=w3938, "PhoenixMotorControlDevRef"=w3928) -> ("error out"=w3919:errorcluster, "PhoenixMotorControlDevRef"=w3920:T7)  [unwired: 6 in]
        n1115 = call "Drive_Vi.vi"("Middle Thumb"=FALSE, "Z"=0.0, "Y"=0.0, "X"=0.0) -> ()  [unwired: 8 in]
        n1116 = Greater?(x=w3924, y=35) -> (0:w3923:bool)
        n1117 = call-poly <vilib>:"NT Read Value.vi"("Default Value"=0.0, "Name"="/limelight-drtrain/ty") -> ("Numeric"=w3932:dbl)  [unwired: 8 in, 1 out]
        "Ty 19" <- w3932
        n1118 = Wait (ms)(milliseconds to wait=u32 100) -> ()  [unwired: 1 out]
        n1119 = call "Shooter_Equation.vi"("Right Trigger"=0.0, "Ty"=w3932) -> ()  [unwired: 10 in]
      }
      n1120 = while {
        tunnel: w3742 -> [w3902]
        tunnel: w3741 -> [w3901]
        tunnel: w3740 -> [w3900]
        tunnel: w3739 -> [w3899]
        tunnel: [w3894] -> w3738
        tunnel: [w3893] -> w3737
        tunnel: [w3892] -> w3736
        tunnel: [w3891] -> w3735
        tunnel: w3715 -> [w3885]
        tunnel: w3714 -> [w3886]
        tunnel: [w3886] -> w3713
        tunnel: [w3885] -> w3712
        i -> [w3896]
        stop <- w3895 stop-if-true
        w3913 = T11 0 items=["PercentOutput"=0, "Position"=1, "Velocity"=2, "Current"=3, "Follower"=5, "MotionProfile"=6, "MotionMagic"=7, "MotionProfileArc"=10, "Disabled"=15] ("Control Mode")
        w3914 = T11 0 items=["PercentOutput"=0, "Position"=1, "Velocity"=2, "Current"=3, "Follower"=5, "MotionProfile"=6, "MotionMagic"=7, "MotionProfileArc"=10, "Disabled"=15] ("Control Mode")
        # "-0.186"
        # "-0.944"
        # ".135"
        n1121 = call "Turret_Aim.vi"("View Button"=FALSE, "Left Trigger"=0.0, "Orange Limit Pressed"=w3885, "Blue Limit Pressed"=w3886, "Right Bumper"=FALSE, "Left Bumper"=FALSE) -> ()  [unwired: 6 in]
        n1122 = call "Drive_Vi.vi"("Middle Thumb"=FALSE, "Z"=0.0, "Y"=0.75, "X"=0.0) -> ()  [unwired: 8 in]
        n1123 = call <vilib>:"CTRE_Phoenix_MotorControl_Set.vi"("error in (no error)"=w3901, "Output"=1.0, "Control Mode"=w3913, "PhoenixMotorControlDevRef"=w3902) -> ("error out"=w3893:errorcluster, "PhoenixMotorControlDevRef"=w3894:T7)  [unwired: 6 in]
        n1124 = call <vilib>:"CTRE_Phoenix_MotorControl_Set.vi"("error in (no error)"=w3899, "Output"=-0.1, "Control Mode"=w3914, "PhoenixMotorControlDevRef"=w3900) -> ("error out"=w3891:errorcluster, "PhoenixMotorControlDevRef"=w3892:T7)  [unwired: 6 in]
        n1125 = Greater?(x=w3896, y=5) -> (0:w3895:bool)
        n1126 = Wait (ms)(milliseconds to wait=u32 50) -> ()  [unwired: 1 out]
        n1127 = call-poly <vilib>:"NT Read Value.vi"("Default Value"=0.0, "Name"="/limelight-drtrain/ty") -> ("Numeric"=w3904:dbl)  [unwired: 8 in, 1 out]
        "Ty 20" <- w3904
        n1128 = call "Shooter_Equation.vi"("Right Trigger"=0.0, "Ty"=w3904) -> ()  [unwired: 10 in]
      }
      n1129 = while {
        tunnel: w3738 -> [w3872]
        tunnel: [w3865] -> _
        tunnel: w3736 -> [w3871]
        tunnel: w3735 -> [w3870]
        tunnel: w3737 -> [w3865]
        tunnel: [w3864] -> w3718
        tunnel: [w3863] -> w3717
        tunnel: [w3862] -> w3723
        tunnel: [w3861] -> w3721
        tunnel: w3713 -> [w3857]
        tunnel: w3712 -> [w3856]
        i -> [w3867]
        stop <- w3866 stop-if-true
        (unwired) FALSE ("Orange Limit Pressed")
        w3883 = T11 0 items=["PercentOutput"=0, "Position"=1, "Velocity"=2, "Current"=3, "Follower"=5, "MotionProfile"=6, "MotionMagic"=7, "MotionProfileArc"=10, "Disabled"=15] ("Control Mode")
        w3884 = T11 0 items=["PercentOutput"=0, "Position"=1, "Velocity"=2, "Current"=3, "Follower"=5, "MotionProfile"=6, "MotionMagic"=7, "MotionProfileArc"=10, "Disabled"=15] ("Control Mode")
        # "-0.186"
        # "-0.944"
        # ".135"
        n1130 = call "Turret_Aim.vi"("View Button"=FALSE, "Left Trigger"=2.0, "Orange Limit Pressed"=w3856, "Blue Limit Pressed"=w3857, "Right Bumper"=FALSE, "Left Bumper"=FALSE) -> ()  [unwired: 6 in]
        n1131 = call "Drive_Vi.vi"("Middle Thumb"=FALSE, "Z"=0.0, "Y"=-0.1, "X"=0.0) -> ()  [unwired: 8 in]
        n1132 = call <vilib>:"CTRE_Phoenix_MotorControl_Set.vi"("error in (no error)"=w3865, "Output"=0.0, "Control Mode"=w3883, "PhoenixMotorControlDevRef"=w3872) -> ("error out"=w3861:errorcluster, "PhoenixMotorControlDevRef"=w3862:T7)  [unwired: 6 in]
        n1133 = call <vilib>:"CTRE_Phoenix_MotorControl_Set.vi"("error in (no error)"=w3870, "Output"=-0.35, "Control Mode"=w3884, "PhoenixMotorControlDevRef"=w3871) -> ("error out"=w3864:errorcluster, "PhoenixMotorControlDevRef"=w3863:T7)  [unwired: 6 in]
        n1134 = Greater?(x=w3867, y=10) -> (0:w3866:bool)
        n1135 = Wait (ms)(milliseconds to wait=u32 100) -> ()  [unwired: 1 out]
        n1136 = call-poly <vilib>:"NT Read Value.vi"("Default Value"=0.0, "Name"="/limelight-drtrain/ty") -> ("Numeric"=w3874:dbl)  [unwired: 8 in, 1 out]
        "Ty 21" <- w3874
        n1137 = call "Shooter_Equation.vi"("Right Trigger"=2.0, "Ty"=w3874) -> ()  [unwired: 10 in]
      }
      n1138 = while {
        tunnel: [w3800] -> w3722
        tunnel: w3723 -> [w3800]
        tunnel: [w3799] -> w3720
        tunnel: w3721 -> [w3799]
        tunnel: [w3798] -> w3719
        tunnel: w3718 -> [w3798]
        tunnel: [w3797] -> w3716
        tunnel: w3717 -> [w3797]
        i -> [w3790]
        stop <- w3789 stop-if-true
        n1139 = Greater?(x=w3790, y=4) -> (0:w3789:bool)
        n1140 = call "Drive_Vi.vi"("Middle Thumb"=TRUE, "Z"=0.15, "Y"=0.0, "X"=0.0) -> ()  [unwired: 8 in]
        n1141 = Wait (ms)(milliseconds to wait=u32 100) -> ()  [unwired: 1 out]
      }
      n1142 = while {
        tunnel: w3722 -> [w3842]
        tunnel: w3720 -> [w3835]
        tunnel: w3716 -> [w3841]
        tunnel: w3719 -> [w3840]
        i -> [w3837]
        stop <- w3836 stop-if-true
        w3853 = T11 0 items=["PercentOutput"=0, "Position"=1, "Velocity"=2, "Current"=3, "Follower"=5, "MotionProfile"=6, "MotionMagic"=7, "MotionProfileArc"=10, "Disabled"=15] ("Control Mode")
        w3854 = T11 0 items=["PercentOutput"=0, "Position"=1, "Velocity"=2, "Current"=3, "Follower"=5, "MotionProfile"=6, "MotionMagic"=7, "MotionProfileArc"=10, "Disabled"=15] ("Control Mode")
        # "-0.186"
        # "-0.944"
        # ".135"
        n1143 = call "Drive_Vi.vi"("Middle Thumb"=FALSE, "Z"=0.0, "Y"=0.0, "X"=0.0) -> ()  [unwired: 8 in]
        n1144 = call <vilib>:"CTRE_Phoenix_MotorControl_Set.vi"("error in (no error)"=w3835, "Output"=0.0, "Control Mode"=w3853, "PhoenixMotorControlDevRef"=w3842) -> ()  [unwired: 6 in, 2 out]
        n1145 = call <vilib>:"CTRE_Phoenix_MotorControl_Set.vi"("error in (no error)"=w3840, "Output"=0.0, "Control Mode"=w3854, "PhoenixMotorControlDevRef"=w3841) -> ()  [unwired: 6 in, 2 out]
        n1146 = Greater?(x=w3837, y=20) -> (0:w3836:bool)
        n1147 = Wait (ms)(milliseconds to wait=u32 100) -> ()  [unwired: 1 out]
        n1148 = call-poly <vilib>:"NT Read Value.vi"("Default Value"=0.0, "Name"="/limelight-drtrain/ty") -> ("Numeric"=w3844:dbl)  [unwired: 8 in, 1 out]
        "Ty 22" <- w3844
        n1149 = call "Shooter_Equation.vi"("Right Trigger"=0.0, "Ty"=w3844) -> ()  [unwired: 10 in]
      }
    }
    frame "Angle Test" {
      n1150 = call <vilib>:"CTRE_Phoenix_MotorControl_RefNumRegistryGet.vi"("refnum name"="Orange Back Turn") -> ("error out"=w4142:errorcluster, "PhoenixMotorControlDevRef"=w4143:T7)  [unwired: 9 in]
      n1151 = call <vilib>:"CTRE_Phoenix_MotorControl_RefNumRegistryGet.vi"("refnum name"="Orange Back Drive") -> ("error out"=w4140:errorcluster, "PhoenixMotorControlDevRef"=w4141:T7)  [unwired: 9 in]
      n1152 = while {
        tunnel: w4143 -> [w4186]
        tunnel: w4142 -> [w4184]
        tunnel: w4141 -> [w4179]
        tunnel: w4140 -> [w4178]
        tunnel: [w4175] -> w4137
        tunnel: [w4174] -> w4136
        tunnel: [w4173] -> w4135
        tunnel: [w4172] -> w4134
        i -> [w4189]
        stop <- w4187 stop-if-true
        w4176 = T11 0 items=["PercentOutput"=0, "Position"=1, "Velocity"=2, "Current"=3, "Follower"=5, "MotionProfile"=6, "MotionMagic"=7, "MotionProfileArc"=10, "Disabled"=15] ("Control Mode")
        w4181 = T11 0 items=["PercentOutput"=0, "Position"=1, "Velocity"=2, "Current"=3, "Follower"=5, "MotionProfile"=6, "MotionMagic"=7, "MotionProfileArc"=10, "Disabled"=15] ("Control Mode")
        n1153 = call <vilib>:"CTRE_Phoenix_MotorControl_SetSelectedSensorPosition.vi"("error in (no error)"=w4184, "New Sensor Position"=0, "PhoenixMotorControlDevRef"=w4186) -> ("error out"=w4183:errorcluster, "PhoenixMotorControlDevRef"=w4185:T7)  [unwired: 7 in]
        n1154 = Wait (ms)(milliseconds to wait=u32 20) -> ()  [unwired: 1 out]
        n1155 = call <vilib>:"CTRE_Phoenix_MotorControl_Set.vi"("error in (no error)"=w4178, "Output"=0.0, "Control Mode"=w4176, "PhoenixMotorControlDevRef"=w4179) -> ("error out"=w4172:errorcluster, "PhoenixMotorControlDevRef"=w4173:T7)  [unwired: 6 in]
        n1156 = call <vilib>:"CTRE_Phoenix_MotorControl_Set.vi"("error in (no error)"=w4183, "Output"=0.0, "Control Mode"=w4181, "PhoenixMotorControlDevRef"=w4185) -> ("error out"=w4174:errorcluster, "PhoenixMotorControlDevRef"=w4175:T7)  [unwired: 6 in]
        n1157 = Greater?(x=w4189, y=u32 10) -> (0:w4187:bool)
      }
      n1158 = while {
        tunnel: w4137 -> [w4160]
        tunnel: w4136 -> [w4161]
        tunnel: w4135 -> [w4165]
        tunnel: w4134 -> [w4164]
        tunnel: [w4159] -> w4133
        tunnel: [w4158] -> w4132
        tunnel: [w4157] -> w4131
        tunnel: [w4156] -> w4130
        i -> [w4170]
        stop <- w4168 stop-if-true
        w4162 = T11 0 items=["PercentOutput"=0, "Position"=1, "Velocity"=2, "Current"=3, "Follower"=5, "MotionProfile"=6, "MotionMagic"=7, "MotionProfileArc"=10, "Disabled"=15] ("Control Mode")
        w4167 = T11 1 items=["PercentOutput"=0, "Position"=1, "Velocity"=2, "Current"=3, "Follower"=5, "MotionProfile"=6, "MotionMagic"=7, "MotionProfileArc"=10, "Disabled"=15] ("Control Mode")
        n1159 = Wait (ms)(milliseconds to wait=u32 20) -> ()  [unwired: 1 out]
        n1160 = call <vilib>:"CTRE_Phoenix_MotorControl_Set.vi"("error in (no error)"=w4164, "Output"=0.0, "Control Mode"=w4162, "PhoenixMotorControlDevRef"=w4165) -> ("error out"=w4156:errorcluster, "PhoenixMotorControlDevRef"=w4157:T7)  [unwired: 6 in]
        n1161 = call <vilib>:"CTRE_Phoenix_MotorControl_Set.vi"("error in (no error)"=w4161, "Output"=1024.0, "Control Mode"=w4167, "PhoenixMotorControlDevRef"=w4160) -> ("error out"=w4158:errorcluster, "PhoenixMotorControlDevRef"=w4159:T7)  [unwired: 6 in]
        n1162 = Greater?(x=w4170, y=u32 10) -> (0:w4168:bool)
      }
      n1163 = while {
        tunnel: w4133 -> [w4144]
        tunnel: w4132 -> [w4145]
        tunnel: w4131 -> [w4149]
        tunnel: w4130 -> [w4148]
        i -> [w4154]
        stop <- w4152 stop-if-true
        w4146 = T11 0 items=["PercentOutput"=0, "Position"=1, "Velocity"=2, "Current"=3, "Follower"=5, "MotionProfile"=6, "MotionMagic"=7, "MotionProfileArc"=10, "Disabled"=15] ("Control Mode")
        w4151 = T11 0 items=["PercentOutput"=0, "Position"=1, "Velocity"=2, "Current"=3, "Follower"=5, "MotionProfile"=6, "MotionMagic"=7, "MotionProfileArc"=10, "Disabled"=15] ("Control Mode")
        n1164 = Wait (ms)(milliseconds to wait=u32 20) -> ()  [unwired: 1 out]
        n1165 = call <vilib>:"CTRE_Phoenix_MotorControl_Set.vi"("error in (no error)"=w4148, "Output"=-0.1, "Control Mode"=w4146, "PhoenixMotorControlDevRef"=w4149) -> ()  [unwired: 6 in, 2 out]
        n1166 = call <vilib>:"CTRE_Phoenix_MotorControl_Set.vi"("error in (no error)"=w4145, "Output"=0.0, "Control Mode"=w4151, "PhoenixMotorControlDevRef"=w4144) -> ()  [unwired: 6 in, 2 out]
        n1167 = Greater?(x=w4154, y=u32 10) -> (0:w4152:bool)
      }
    }
  }
